vi "myRIO_BRig_RT_v0,79__PortC.vi"() -> ()   [LabVIEW 2014]
uses:
  myRIO_BRig_RT__Case_Exp_stateList.ctl
  myRIO_BRig_RT__Case_NonExp_stateList.ctl
  <vilib>/Platform/TimedLoop/XDataNode/timing_clust.ctl
  <vilib>/Platform/TimedLoop/XDataNode/nitl_modes.ctl
  <vilib>/Platform/TimedLoop/XDataNode/wakeup.ctl
  <vilib>/WebDAVClient/Advanced/SessionHandle.ctl
  <vilib>/myRIO/Common/Instrument Driver Framework/myRIO v1.0/UART/vis/myRIO v1.0 Close UART.vi
  <vilib>/FPGAPlugInAG/myRIO-1900/niLvFpga_Open_myRIO-1900.vi
  <vilib>/rvi/interface/common/dynamic/niFpgaDynamicAddResources.vi
  <vilib>/Utility/error.llb/Error Cluster From Error Code.vi
  <vilib>/rvi/errors/niLvFpgaAdjustHostInterfaceError.vi
  <vilib>/FPGAPlugInAG/Dynamic/niLvFpga_Close_Dynamic.vi
  <vilib>/myRIO/Common/Instrument Driver Framework/Utilities/vis/FPGA Ref Manager.vi
  <vilib>/myRIO/Common/Instrument Driver Framework/myRIO v1.0/myRIO v1.0 Reset FPGA.vi
  <vilib>/myRIO/Common/Instrument Driver Framework/myRIO v1.0/IRQ/vis/myRIO v1.0 IRQ Info FGV.vi
  <vilib>/myRIO/Common/Instrument Driver Framework/myRIO v1.0/IRQ/vis/myRIO v1.0 Timer IRQ Info FGV.vi
  <vilib>/myRIO/Common/Instrument Driver Framework/myRIO v1.0/IRQ/vis/myRIO v1.0 ISR Agent.vi
  <vilib>/rvi/interface/nirviOpenFPGA/nirviOpenFPGA.xnode
  FPGA Bitfiles/myRIOBRig_FPGATarget_myRIOBRigFPGAv3,_Jim92IOu6W4.lvbitx
  myRIO_BRig_FPGA_v3,70__PortC.vi
  <vilib>/rvi/interface/nirviReadWriteControl/nirviReadWriteControl.xnode
  <vilib>/Platform/TimedLoop/XDataNode/XDataNode.xnode
  <vilib>/rvi/interface/nirviCloseFPGA/nirviCloseFPGA.xnode
  <vilib>/Platform/TimedLoop/XDataNode/XDNodeRunTimeDep.lvlib
  <vilib>/rvi/interface/Simulation/niFpgaSimulationCallBeginRW.vi
  <vilib>/myRIO/Instrument Drivers/Utilities/Utilities.lvlib
  <vilib>/WebDAVClient/NI_WebDAV.lvlib
  NiFpgaLv.dll
panel:
  out "power_l2":dbl
  out "error out 6":errorcluster
  in  "MTrig_Laser_Switch":bool
  in  "Cue1Param_AudioLed_Count_NS":u16
  in  "Cue1Param_AudioLed_Count_Switch":u16
  in  "Cue1Param_AudioLed_Probability_NS":u16
  in  "Cue1Param_CueType_NS":u16(slide) max=2 step=1 scale=0.0..2.0
  in  "Cue1Param_AudioLed_Probability_Switch":u16
  in  "Cue1Param_CueType_Switch":u16(slide) max=2 step=1 scale=0.0..2.0
  in  "CueLed_Freq":dbl=10.0
  in  "CueLed_Tpeak":dbl=2.0
  in  "CueLed_duration":u16
  in  "Laser_power_step_l2":dbl
  in  "Laser_power_max_l2":dbl
  in  "Laser_power_min_l2":dbl
  in  "Laser_Tshutter_l2":dbl=2.0
  in  "Laser_Freq_l2":dbl=10.0
  in  "Laser_Tpeak_l2":dbl=2.0
  in  "Laser_duration_l2":u16
  in  "LC_Sel_Count_NS_l2":u16
  in  "LC_Sel_Count_Switch_l2":u16
  in  "LC_Sel_Probability_NS_l2":u16
  in  "LC_Sel_Block_NS_l2":u16(slide) max=2 step=1 scale=0.0..2.0
  in  "LC_Sel_OnOff_NS_l2":bool
  in  "LC_Sel_Probability_Switch_l2":u16
  in  "LC_Sel_Block_Switch_l2":u16(slide) max=2 step=1 scale=0.0..2.0
  in  "LC_Sel_OnOff_Switch_l2":bool
  in  "LC_Sel_Tdelay_NS_l2":u16
  in  "LC_Sel_Tdelay_Switch_l2":u16
  in  "LC_Cue1_Count_NS_l2":u16
  in  "LC_Cue1_Count_Switch_l2":u16
  in  "LC_Cue1_delayOpt_NS_l2":bool
  in  "LC_ENL1_delayOpt_NS_l2":bool
  in  "LC_ENL1_Count_NS_l2":u16
  in  "LC_ENL1_Count_Switch_l2":u16
  in  "LC_Cue1_delayOpt_Switch_l2":bool
  in  "LC_ENL1_delayOpt_Switch_l2":bool
  in  "LC_Cue1_Probability_NS_l2":u16
  in  "LC_Cue1_Block_NS_l2":u16(slide) max=2 step=1 scale=0.0..2.0
  in  "LC_Cue1_OnOff_NS_l2":bool
  in  "LC_Cue1_Probability_Switch_l2":u16
  in  "LC_Cue1_Block_Switch_l2":u16(slide) max=2 step=1 scale=0.0..2.0
  in  "LC_Cue1_OnOff_Switch_l2":bool
  in  "LC_ENL1_Probability_NS_l2":u16 max=100 step=1
  in  "LC_ENL1_Block_NS_l2":u16(slide) max=2 step=1 scale=0.0..2.0
  in  "LC_ENL1_OnOff_NS_l2":bool
  in  "LC_ENL1_Probability_Switch_l2":u16 max=100 step=1
  in  "LC_ENL1_Block_Switch_l2":u16(slide) max=2 step=1 scale=0.0..2.0
  in  "LC_Cue1_Tdelay_NS_l2":u16
  in  "LC_ENL1_Tdelay_NS_l2":u16
  in  "LC_Cue1_Tdelay_Switch_l2":u16
  in  "LC_ENL1_Tdelay_Switch_l2":u16
  in  "LC_ENL1_OnOff_Switch_l2":bool
  in  "LC_Wrong_Probability_l2":u16
  in  "LC_Wrong_Trial_l2":u16(slide) max=2 step=1 scale=0.0..2.0
  in  "LC_Wrong_Block_l2":u16(slide) max=2 step=1 scale=0.0..2.0
  in  "LC_Wrong_OnOff_l2":bool
  in  "LC_Reward_Probability_l2":u16
  in  "LC_Reward_Trial_l2":u16(slide) max=2 step=1 scale=0.0..2.0
  in  "LC_Reward_Block_l2":u16(slide) max=2 step=1 scale=0.0..2.0
  in  "LC_Reward_OnOff_l2":bool
  in  "LC_Wrong_Tdelay_l2":u16
  in  "LC_Reward_Tdelay_l2":u16
  in  "LC_Sel_Count_NS_l1":u16
  in  "LC_Sel_Count_Switch_l1":u16
  in  "LC_Sel_Probability_NS_l1":u16
  in  "LC_Sel_Block_NS_l1":u16(slide) max=2 step=1 scale=0.0..2.0
  in  "LC_Sel_OnOff_NS_l1":bool
  in  "LC_Sel_Probability_Switch_l1":u16
  in  "LC_Sel_Block_Switch_l1":u16(slide) max=2 step=1 scale=0.0..2.0
  in  "LC_Sel_OnOff_Switch_l1":bool
  in  "LC_Sel_Tdelay_NS_l1":u16
  in  "LC_Sel_Tdelay_Switch_l1":u16
  out "I_connect_TCP":bool
  out "error out 5":errorcluster
  in  "get_countPerMS":bool
  in  "count_warmup_R_reset":bool
  in  "count_warmup_L_reset":bool
  out "count_warmup_R":u16
  out "count_warmup_L":u16
  out "SolenoidReward":bool
  in  "SolenoidProbability_L":u16=50 caption="Reward Time [ms]" min=1 max=1000 step=1
  in  "SolenoidProbability_R":u16=50 caption="Reward Time [ms]" min=1 max=1000 step=1
  out "power_l1":dbl caption="LaserPower"
  out "error out 4":errorcluster
  in  "Laser_power_step_l1":dbl
  in  "Laser_power_max_l1":dbl
  in  "Recording":bool
  out "error out 3":errorcluster
  out "error out 2":errorcluster
  in  "Laser_power_min_l1":dbl
  in  "FPGA_count2ms":dbl=159.0
  in  "Laser_Tshutter_l1":dbl=2.0
  in  "Laser_Freq_l1":dbl=10.0
  in  "Laser_Tpeak_l1":dbl=2.0
  in  "Laser_duration_l1":u16
  out "error out":errorcluster
  in  "LC_Cue1_Count_NS_l1":u16
  in  "LC_Cue1_Count_Switch_l1":u16
  in  "LC_Cue1_delayOpt_NS_l1":bool
  in  "LC_ENL1_delayOpt_NS_l1":bool
  in  "LC_ENL1_Count_NS_l1":u16
  in  "LC_ENL1_Count_Switch_l1":u16
  in  "LC_Cue1_delayOpt_Switch_l1":bool
  in  "LC_ENL1_delayOpt_Switch_l1":bool
  in  "Tcycle_Cue_max":u16=1000 caption="Max" min=5 max=5000 step=5
  in  "Tcycle_Cue_min":u16=1000 caption="Min" min=5 max=5000 step=5
  in  "SendData":bool
  out "cSpout":enum16{"Left", "Right"}(ring) caption="Left or Right Spout"
  out "A4":u32 caption="LickCounter_Right"
  out "A2":u32 caption="LickCounter_Left"
  in  "LR_wrong_Event":bool
  out "error_initTrial":errorcluster
  out "error_Selection_pre":errorcluster
  out "error_Selection":errorcluster
  out "SelectWrong":bool
  out "SelectReward":bool
  in  "Left(F)_or_Right(T)":bool
  in  "ignoreWrong":bool
  in  "SelectionState":bool
  in  "LR_wrong_Laser":bool
  in  "LR_reward_Laser":bool
  in  "LR_reward_Event":bool
  out "nRewards_Right":u16 caption="# Rewards Total (Right)"
  out "nRewards_Left":u16 caption="# Rewards Total (Left)"
  out "nRewards_cur":u16 caption="# Rewards in Current Block"
  out "TpB_target":u16 caption="Target Trials Per Block"
  out "cState_NonExp":T1 caption="WarmUp State"
  out "iBlock":u16 caption="Current Block"
  out "cState":T2 caption="Experimental State"
  out "iTrial":u16 caption="Current Trial"
  in  "warmupType":u8(slide) max=2 step=1 scale=0.0..2.0
  in  "TestConnection":bool
  in  "warmup":bool caption="WarmUp"
  in  "Data Set Prefix":string="Exp1_TM2"
  out "Connected To Host?":bool
  in  "Host Password":string="sabalab"
  in  "Host UserName":string="Test2"
  in  "sp_RightSpout":u16(slide)=2 max=2 step=1 scale=0.0..2.0
  in  "sp_LeftSpout":u16(slide)=2 max=2 step=1 scale=0.0..2.0
  in  "BUR_max":u16 caption="Count Reward Structure  (0 = off)"
  in  "LC_Wrong_Probability_l1":u16
  in  "LC_Wrong_Trial_l1":u16(slide) max=2 step=1 scale=0.0..2.0
  in  "LC_Wrong_Block_l1":u16(slide) max=2 step=1 scale=0.0..2.0
  in  "LC_Wrong_OnOff_l1":bool
  in  "LC_Reward_Probability_l1":u16
  in  "LC_Reward_Trial_l1":u16(slide) max=2 step=1 scale=0.0..2.0
  in  "LC_Reward_Block_l1":u16(slide) max=2 step=1 scale=0.0..2.0
  in  "LC_Reward_OnOff_l1":bool
  in  "LC_Cue1_Probability_NS_l1":u16
  in  "LC_Cue1_Block_NS_l1":u16(slide) max=2 step=1 scale=0.0..2.0
  in  "LC_Cue1_OnOff_NS_l1":bool
  in  "LC_Cue1_Probability_Switch_l1":u16
  in  "LC_Cue1_Block_Switch_l1":u16(slide) max=2 step=1 scale=0.0..2.0
  in  "LC_Cue1_OnOff_Switch_l1":bool
  in  "LC_ENL1_Probability_NS_l1":u16 max=100 step=1
  in  "LC_ENL1_Block_NS_l1":u16(slide) max=2 step=1 scale=0.0..2.0
  in  "LC_ENL1_OnOff_NS_l1":bool
  in  "LC_ENL1_Probability_Switch_l1":u16 max=100 step=1
  in  "LC_ENL1_Block_Switch_l1":u16(slide) max=2 step=1 scale=0.0..2.0
  in  "Tcycle_Timeout":u16=1000 caption="Timeout Time [ms]" min=10 max=10000 step=1
  in  "Tcycle_Wrong":u16=1000 caption="Wrong Time [ms]" min=10 max=10000 step=1
  in  "Tcycle_Selection":u16=1000 caption="Answer Time [ms]" min=1 max=10000 step=1
  in  "Tcycle_RewardPost":u16=1000 caption="Consumption Time [ms]" min=250 max=10000 step=250
  in  "Tcycle_Reward_L":u16=500 caption="Reward Time [ms]" min=1 max=1000 step=1
  in  "Tcycle_Reward_R":u16=500 caption="Reward Time [ms]" min=1 max=1000 step=1
  in  "TpB_Max_R":u16=4 caption="Max TrialsPerBlock" min=1 max=12 step=1
  in  "TpB_Min_R":u16=4 caption="Min TrialsPerBlock" min=1 max=12 step=1
  in  "TpB_Max_L":u16=4 caption="Max TrialsPerBlock" min=1 max=12 step=1
  in  "TpB_Min_L":u16=4 caption="Min TrialsPerBlock" min=1 max=12 step=1
  in  "BUR_min":u16 caption="Count Reward Structure\n(0 = off)"
  in  "TrialUntilReward":bool caption="Ignore Wrong Selection"
  in  "CueCycles":u16=1 caption="Cue Structure" min=1 max=1 step=1
  in  "MTrig_Laser_Tcycle":u16=10 caption="Time [ms]"
  in  "MTrig_Laser_trig":bool
  in  "MTrig_Audio_trig__R":bool caption="Trigger Audio"
  in  "MTrig_Audio_trig__L":bool caption="Trigger Audio"
  in  "RewCalib_Trig_R":bool caption="Calibrate_R"
  in  "RewCalib_Trig_L":bool caption="Calibrate_L"
  in  "MTrig_Solenoid_Tcycle__R":u16=300 caption="Time [ms]"
  in  "MTrig_Solenoid_Tcycle__L":u16=300 caption="Time [ms]"
  in  "MTrig_Solenoid_trig__R":bool caption="Solenoid"
  in  "MTrig_Solenoid_trig__L":bool caption="Solenoid"
  in  "STOP_abort":bool caption="Stop LabView\n(Stops myRio and FPGA)"
  in  "STOP_endBlock":bool caption="Stop Experiment\n@ End of Block"
  in  "STOP_endTrial":bool caption="Stop Experiment\n@ End of Trial"
  in  "START":bool caption="Start Experiment"
  in  "Tcycle_CuePenalty":u16=1000 caption="Penalty" min=1 max=10000 step=1
  in  "Audio_Amp__R":u16=100 caption="Amp"
  in  "Audio_Freq__R":u8=5 caption="Freq [kHz]" max=14 step=1
  in  "Audio_Amp__L":u16=100 caption="Amp"
  in  "Audio_Freq__L":u8=5 caption="Freq [kHz]" max=14 step=1
  in  "LC_Wrong_Tdelay_l1":u16
  in  "LC_Cue1_Tdelay_NS_l1":u16
  in  "LC_ENL1_Tdelay_NS_l1":u16
  in  "LC_Reward_Tdelay_l1":u16
  in  "LC_Cue1_Tdelay_Switch_l1":u16
  in  "LC_ENL1_Tdelay_Switch_l1":u16
  in  "LC_ENL1_OnOff_Switch_l1":bool
  in  "Tcycle_ENLPenalty":u16=100 caption="Penalty" min=10 max=10000 step=10
  in  "Tcycle_ENL_max":u16=1000 caption="Max" min=250 max=10000 step=250
  in  "Tcycle_ENL_min":u16=1000 caption="Min" min=250 max=10000 step=250
  # "Communication (Host PC)"
  # "Recording Rig"
  # "Experimental Run"
  # "Current State"
  # "STOP experiment at"
  # "Global Parameters                                                         Trial Parameters"
  # "Left/Right        Give Reward?        Laser Power [V]"
  # "Laser1      Laser2"
  # "FPGA Count per [ms]"
  # "Experiment Task Structure"
  # "Timing [ms]"
  # "Block                   Trial            Target Trials       # Rewards \n                                                            Per Block             Current"
  # "Min            Max            Penalty"
  # "(1) = Switching\n(2) = Two Choice"
  # "WarmUp State"
  # "Lick Counter"
  # "Enforced\nNonLick"
  # "WarmUp"
  # "Left           Right"
  # "Cue then reward (no lick)\n \nLeft                    Right"
  # "# Rewards Total\n                                                                  Left                    Right"
  # "Cue"
  # "Experimental State"
  # "Selection\n \n\n \nReward\n    Dispense\n    Time\n \n    Dispense\n    Probability\n \n\n    Consumption\n    Time\n\nWrong Choice\n \n \nTimeout Penalty"
  # "Left                  Right"
  # "Manual Control"
  # "Min"
  # "Max"
  # "Solenoid\n \nLeft              Right"
  # "Speaker\n \nLeft                    Right"
  # "Laser 1  |  Laser 2"
  # "Trial Per Block Structure \n               Left                        Right"
  # "Time\n[ms]"
  # "Time\n[ms]"
  # "Time = Cue Min"
  # "Min"
  # "Power = Min"
  # "Max"
  # "Cue1 Control\n                                  Cue Type           LED Probability [%]      Count"
  # "Laser1 Control\n                               On/Off      Block        Probability [%]   Delay [ms]                              Count"
  # "Laser2 Control\n                               On/Off      Block        Probability [%]   Delay [ms]                              Count"
  # "Audio or LED"
  # "Cue 1"
  # "Enforced\nNonLick\n      1"
  # "Enforced\nNonLick\n      1"
  # "from end"
  # "from end"
  # "Switch\nTrial"
  # "Switch\nTrial"
  # "Switch\nTrial"
  # "from start"
  # "from start"
  # "from end"
  # "from end"
  # "NonSwitch\nTrials"
  # "NonSwitch\nTrials"
  # "NonSwitch\nTrials"
  # "from start"
  # "from start"
  # "Cue 1"
  # "Cue 1"
  # "from end"
  # "from end"
  # "Switch\nTrial"
  # "Switch\nTrial"
  # "Cue Audio Parameters"
  # "Cue LED Parameters"
  # "from start"
  # "from start"
  # "Left                  Right"
  # "Frequency\n[Hz]"
  # "Frequency\n[kHz]"
  # "from end"
  # "from end"
  # "NonSwitch\nTrials"
  # "NonSwitch\nTrials"
  # "Timing [ms]\n Duration     Peak Width"
  # "from start"
  # "from start"
  # "Amp\n(0 - 32,000)"
  # "Selection"
  # "Selection"
  # "from start"
  # "from start"
  # "Switch\nTrial"
  # "Switch\nTrial"
  # "Speaker\nPattern\nDuring Cue"
  # "from start"
  # "from start"
  # "NonSwitch\nTrials"
  # "NonSwitch\nTrials"
  # "Laser1 Parameters"
  # "Laser2 Parameters"
  # "Laser1 Response\n                               On/Off      Block       Trial       Probability [%]   Delay [ms]"
  # "Laser2 Response\n                               On/Off      Block       Trial       Probability [%]   Delay [ms]"
  # "Frequency\n[Hz]"
  # "Frequency\n[Hz]"
  # "Timing [ms]\n Duration     Peak Width   Shutter"
  # "Timing [ms]\n Duration     Peak Width   Shutter"
  # "Selection Reward"
  # "Selection Reward"
  # "Laser Power [V]\nMin          Max              Step"
  # "Laser Power [V]\nMin          Max              Step"
  # "Selection Wrong"
  # "Selection Wrong"
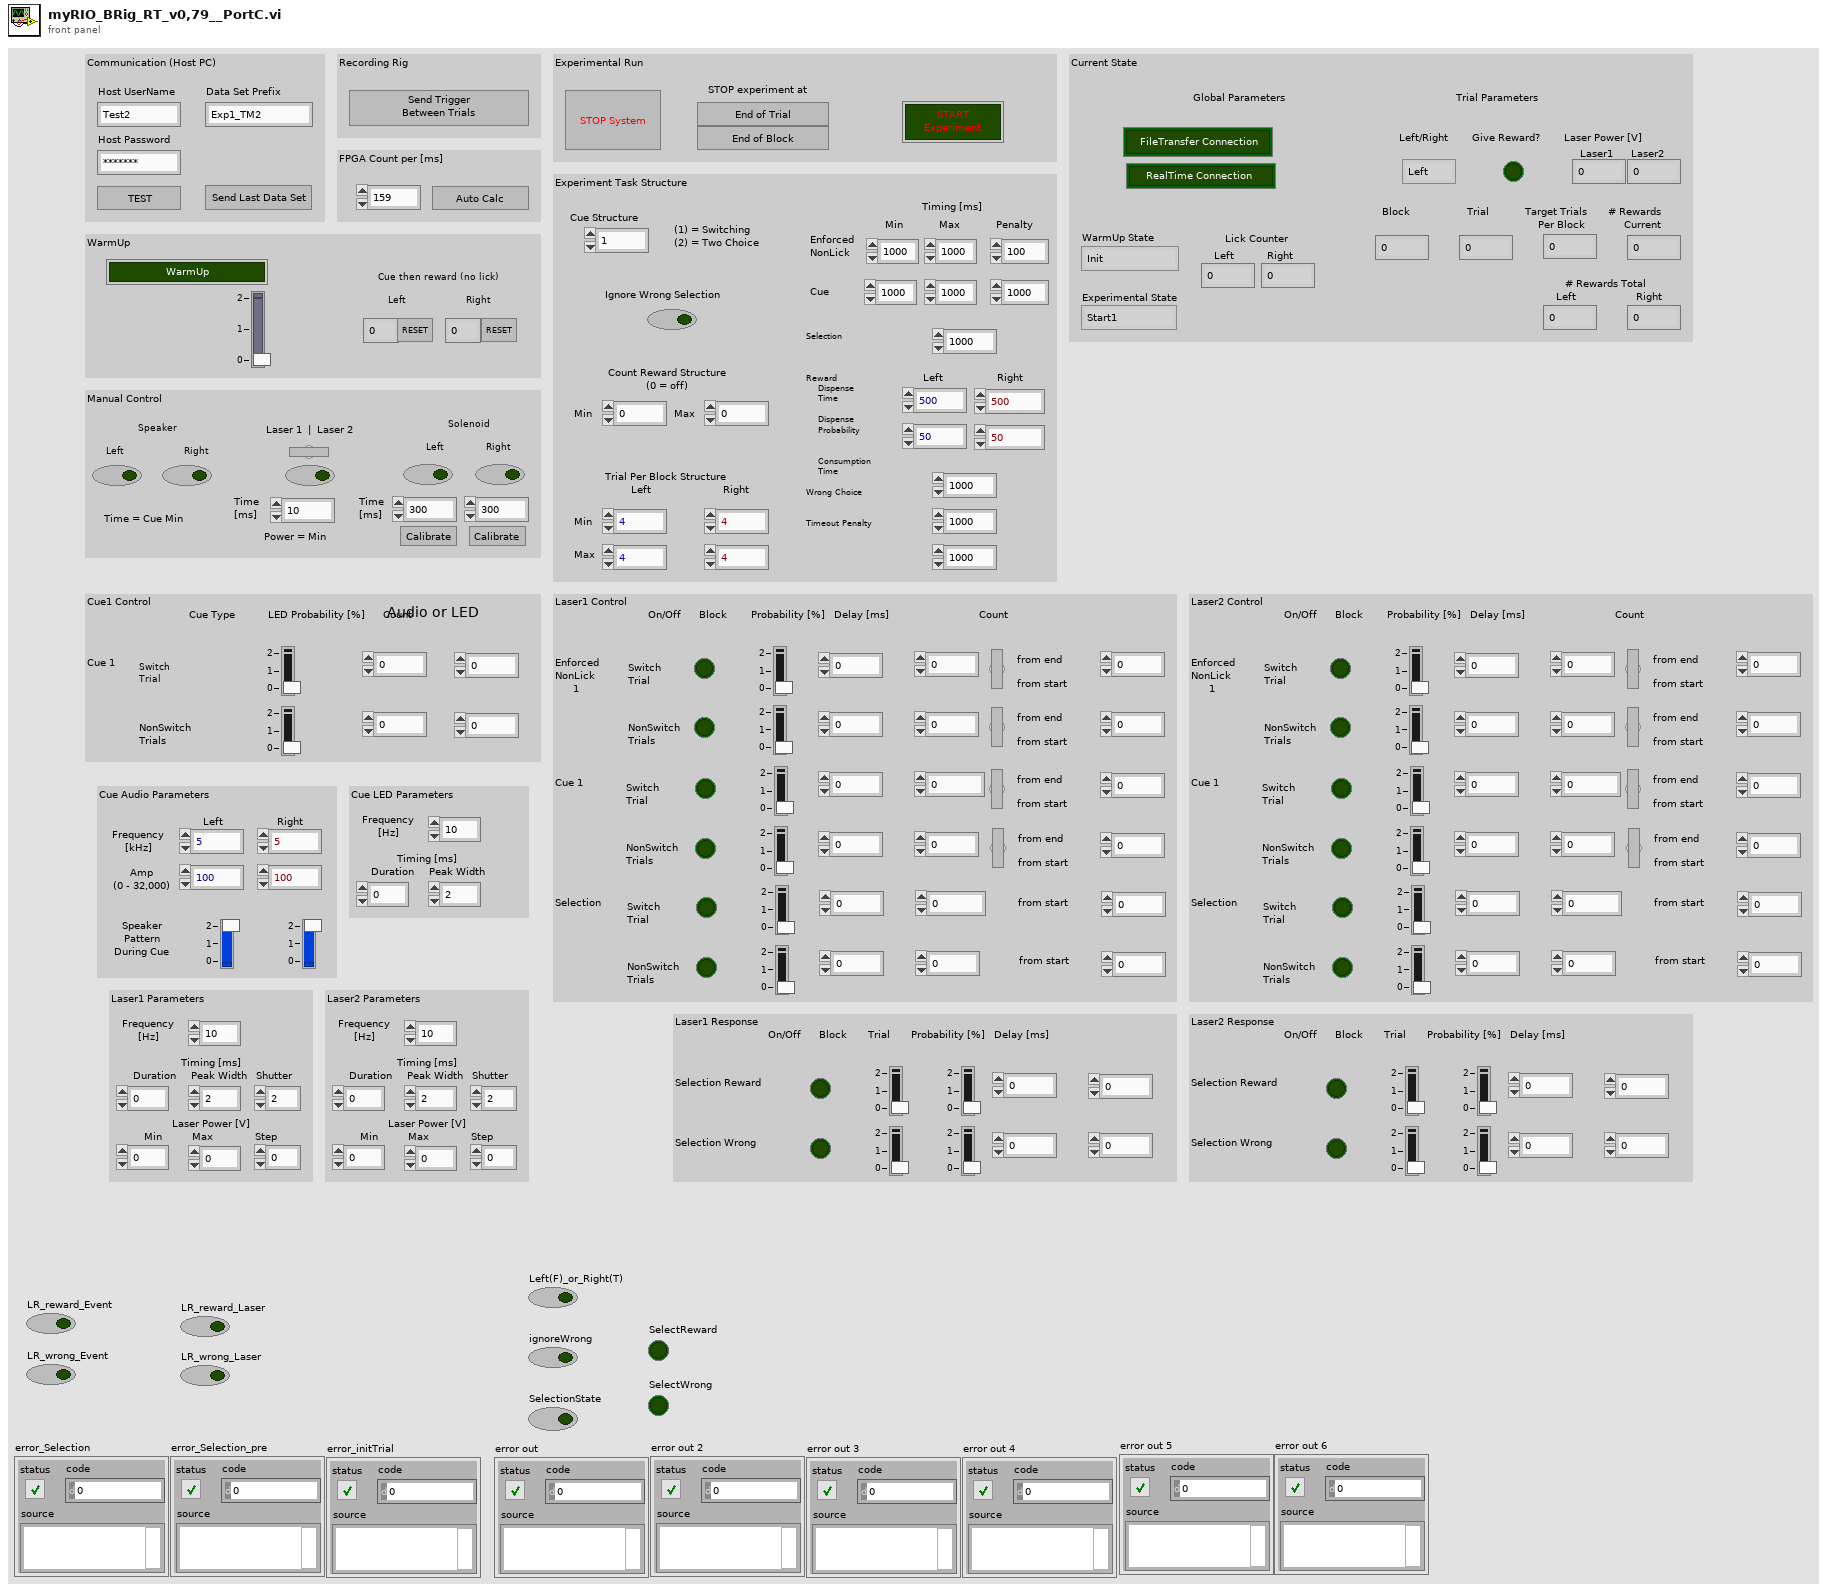
[diagram p1: front panel]
types:
  T1 = typedef "myRIO_BRig_RT__Case_NonExp_stateList.ctl" = enum16{"Init", "UploadSettings_pre", "UploadSettings_Read_dataExp", "UploadSettings_dataExp_1", "UploadSettings_dataExp_2", "UploadSettings_Read_dataLC", "UploadSettings_dataLC_1", "UploadSettings_dataLC_2", "UploadSettings_dataLC_3", "UploadSettings_dataLC_4", "UploadSettings_Read_dataMTrig", "UploadSettings_dataMTrig_1", "UploadSettings_post", "Idle_pre", "IdleEmpty", "IdleEmpty2", "IdleEmpty3", "IdleEmpty4", "Idle", "Idle_2", "Idle_3", "Idle_4", "Idle_5", "Idle_6", "Idle_post", "Cue_pre__pre", "Cue_pre", "Cue", "Cue_LED", "Cue_post", "RewardCalibration_pre", "DispenseWater_pre__pre", "DispenseWater_pre", "DispenseWater", "DispenseWater_post", "TestConnection", "SendData", "Get_FPGA_count_per_ms", "End"}
  T2 = typedef "myRIO_BRig_RT__Case_Exp_stateList.ctl" = enum16{"Start1", "Start2", "Start3", "saveSettings1", "saveSettings2", "saveSettings3", "saveSettings4", "saveSettings_LC_ENL_l1", "saveSettings_LC_ENL_l2", "saveSettings_LC_Cue_l1", "saveSettings_LC_Cue_l2", "saveSettings6_LC_l1_Other", "SaveSettings6_LC_l2_Other", "setSettings_Audio", "setSettings_Laser", "initBlock_pre", "initBlock", "initBlock2", "initBlock_post", "initTrial_pre", "initTrial", "initTrial2", "initTrial3", "initTrial4", "initTrial_LC_ENL1", "initTrial_LC_Cue1", "initTrial_LC_Cue1_2", "initTrial_LC_Sel", "initTrial_post", "ENL1_pre", "ENL1", "ENL1_post", "ENL1Penalty_pre", "ENL1Penalty", "ENL2_pre", "ENL2", "ENL2Penalty_pre", "ENL2Penalty", "Cue1_pre", "Cue1", "Cue1_post", "Cue1Penalty_pre", "Cue1Penalty", "Cue2_pre", "Cue2", "Cue2Penalty_pre", "Cue2Penalty", "Selection_pre", "Selection", "Select_post", "SelectReward_pre", "SelectReward", "SelectRewardPost_pre", "SelectRewardPost", "SelectWrong_pre", "SelectWrong", "SelectWrong_post", "SelectTimeout_pre", "SelectTimeout", "SelectTimeout_post", "endTrial_pre", "endTrial1", "endTrial2", "endTrial3", "endTrial_post", "endBlock_pre", "endBlock", "endBlock_post", "endExp", "commConnect", "commUpload_pre", "commUpload_dataBlock", "commUpload_dataCurrent", "commUpload_dataExp", "commUpload_dataLC", "commUpload_dataTrial", "commUpload_post", "saveData_pre", "saveData_dataBlock", "saveData_dataCurrent", "saveData_dataExp", "saveData_dataLC", "saveData_dataTrial", "saveData_post", "empty_endBlock1", "empty_endBlock2", "empty_endTrial1", "empty_endTrial2", "empty_endTrial3", "empty_endTrial4", "empty_endTrial5", "dummyState", "dummyState_endBlock"}
  T3 = typedef "XDNodeRunTimeDep.lvlib/timing_clust.ctl" = cluster{"Expected End [f-1]":u64, "Actual End [f-1]":u64, "Finished Late? [f-1]":bool, "Expected End [i-1]":u64, "Actual End [i-1]":u64, "Finished Late? [i-1]":bool, "Expected Start [i]":u64, "Actual Start [i]":u64, "Expected Start [f]":u64, "Actual Start [f]":u64, "Source Name":string, "Structure Name":string, "Period":i64, "Deadline":i64, "Offset":i64, "Start":i64, "Priority":i32, "Timeout":i32, "Mode":T4, "Wakeup Reason":T5, "Error":errorcluster, "Source Type":string, "Secondary Source Type":string, "Global End Time":u64, "Global Start Time":u64, "Frame Duration":u64, "Iteration Duration":u64, "Assigned CPU":i32, "I/O Scan Engine Mode":u32}
  T4 = typedef "XDNodeRunTimeDep.lvlib/nitl_modes.ctl" = enum32{"No Change", "Process missed periods, maintain original phase", "Discard missed periods, maintain original phase", "Process missed periods, ignore original phase", "Discard missed periods, ignore original phase"}
  T5 = typedef "XDNodeRunTimeDep.lvlib/wakeup.ctl" = enum32{"Normal", "Aborted", "Asynchronous wakeup", "Timing source error", "Timed loop error", "Timeout"}
  T6 = typedef "NI_WebDAV.lvlib/SessionHandle.ctl" = refnum<k1>
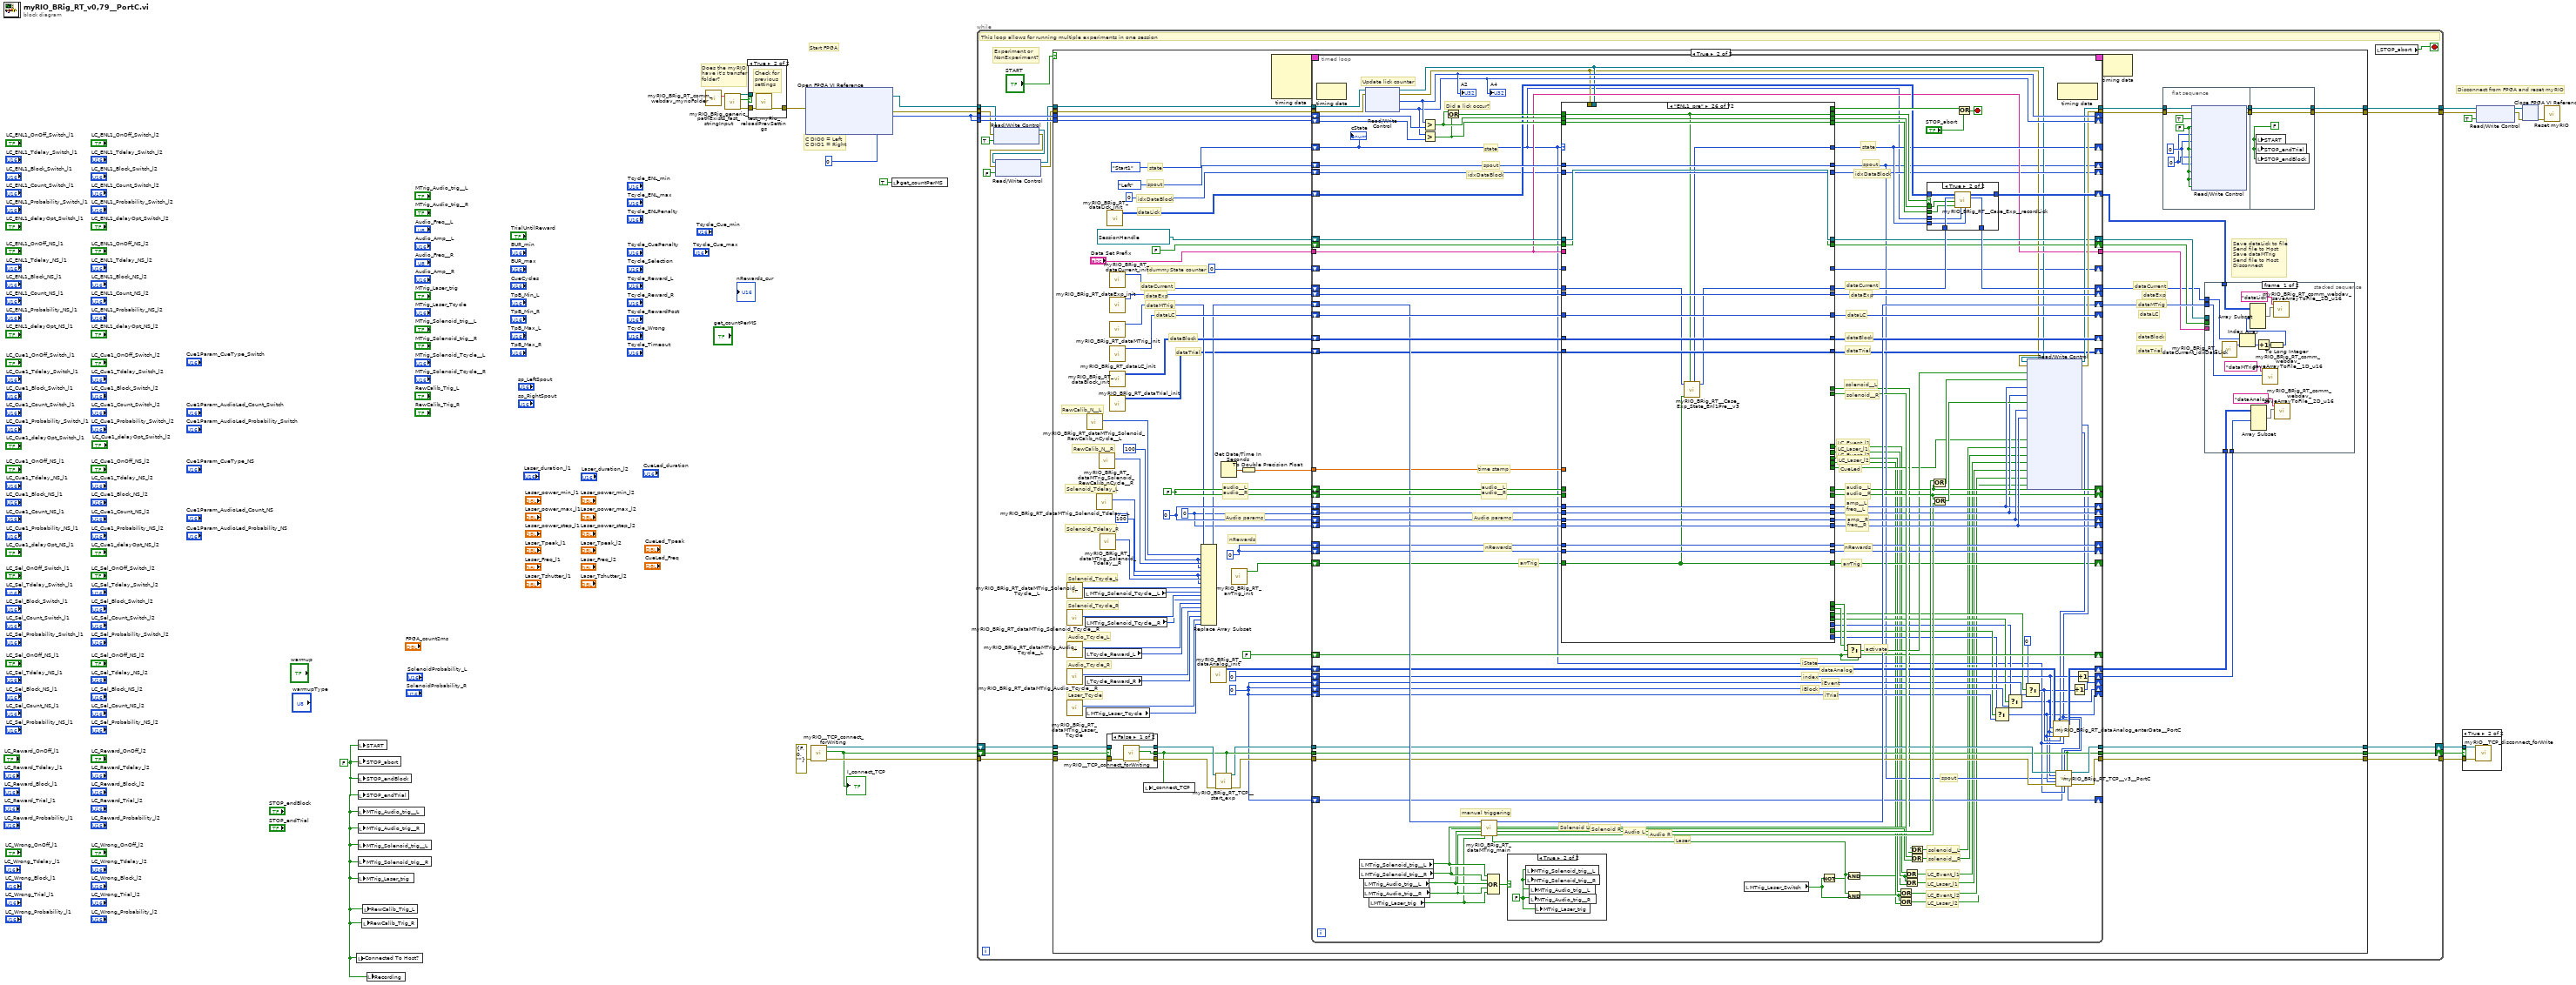
[diagram p0: block diagram]
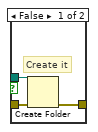
[diagram p3: hidden frame]
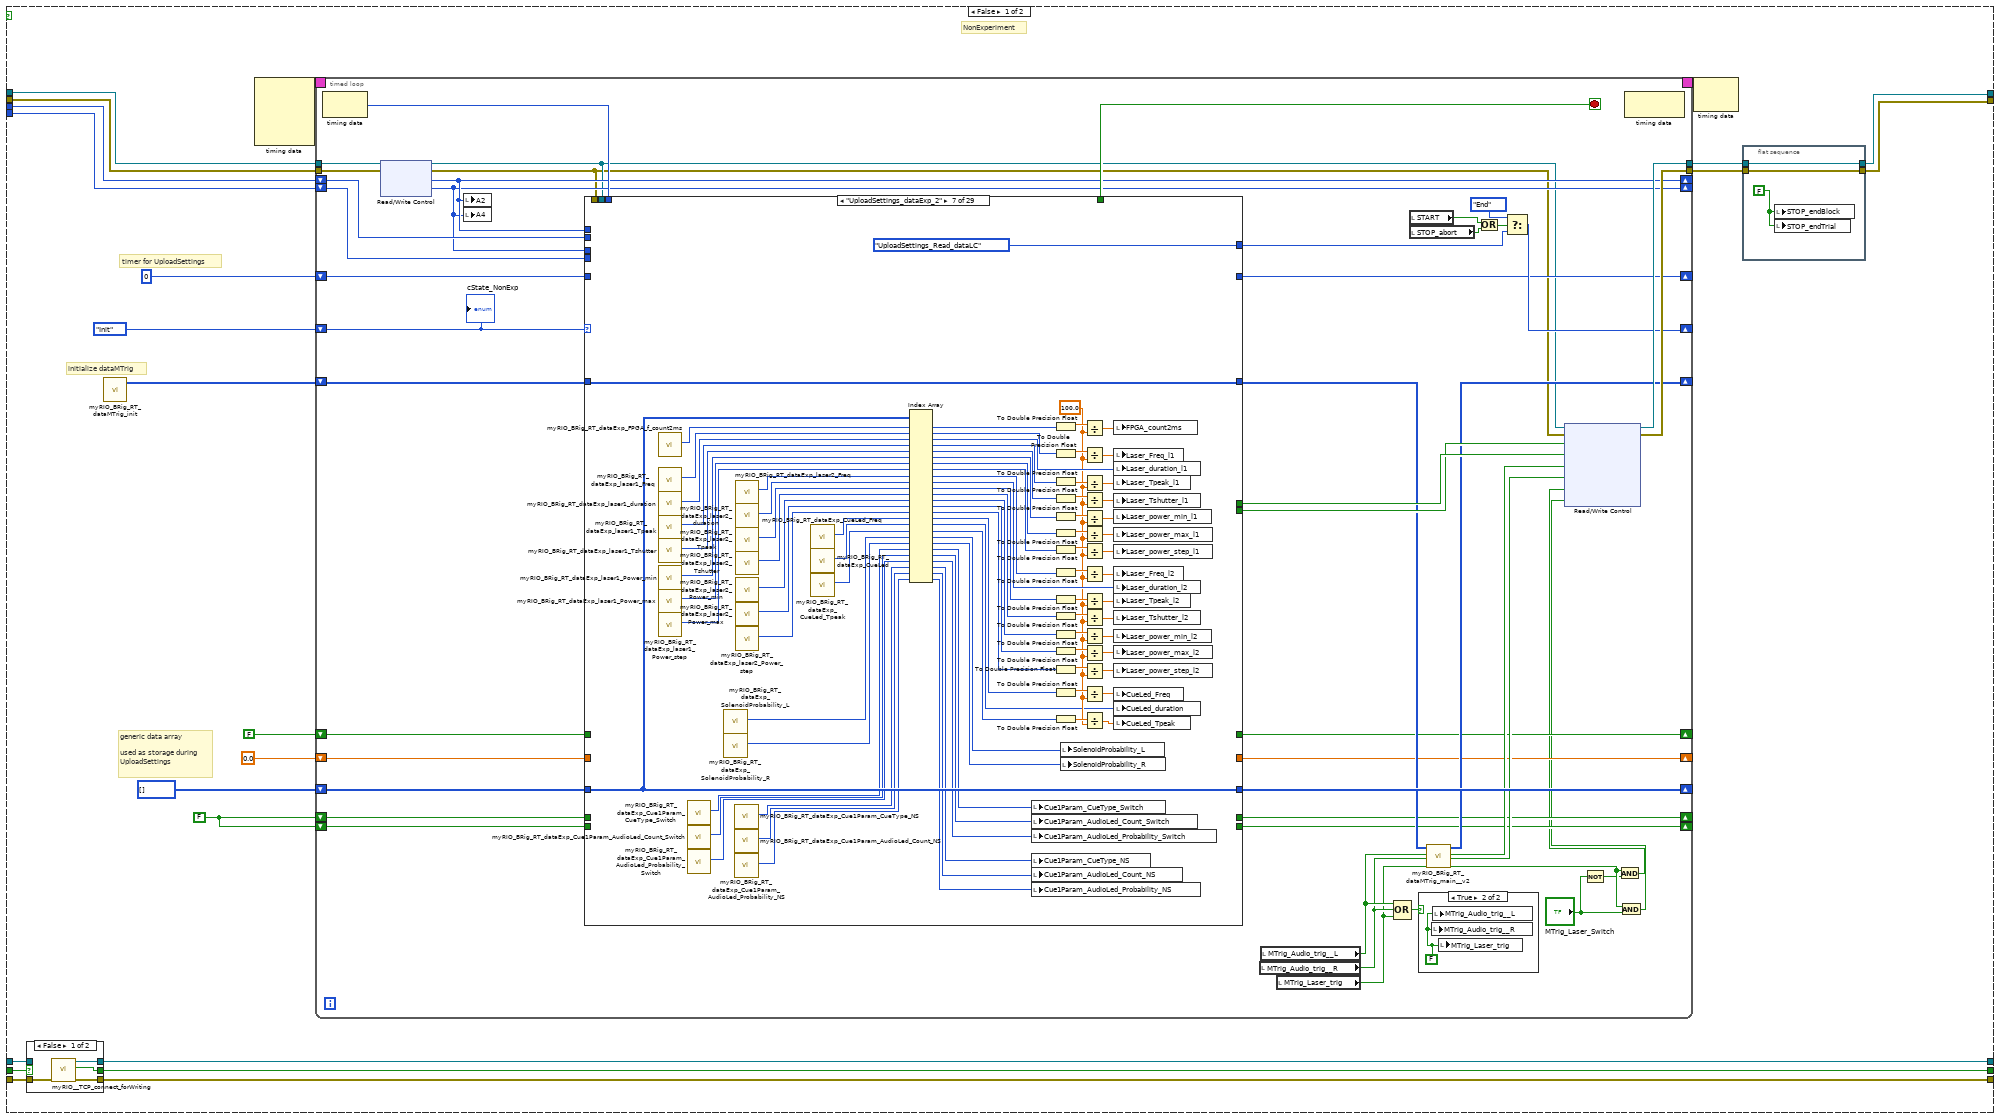
[diagram p4: hidden frame]
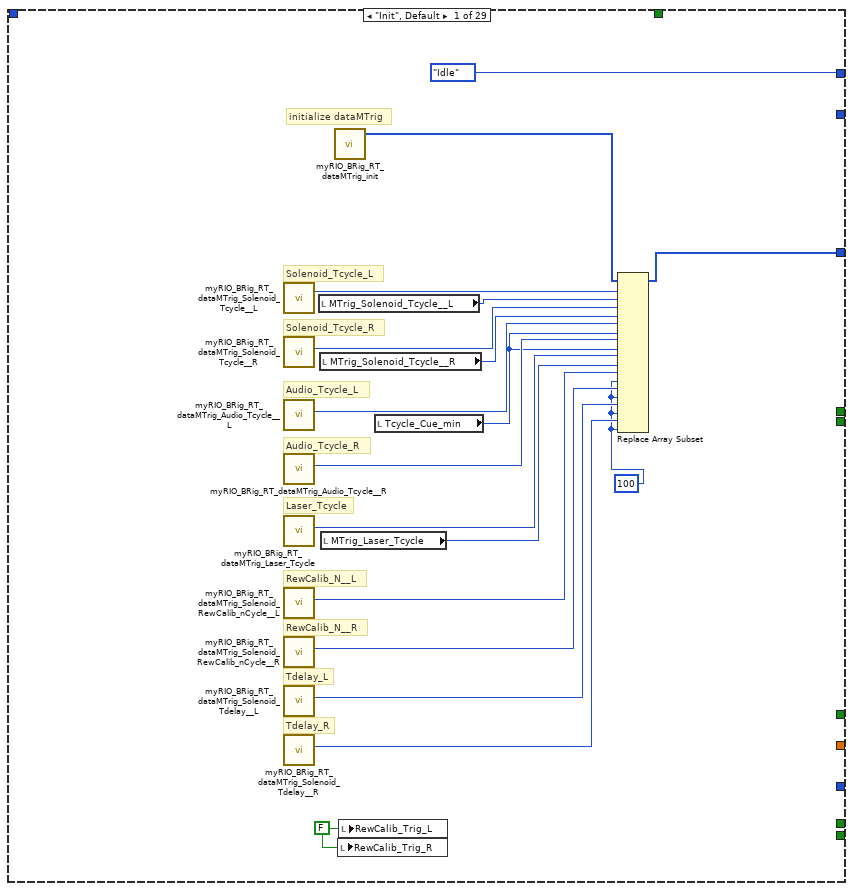
[diagram p7: hidden frame]
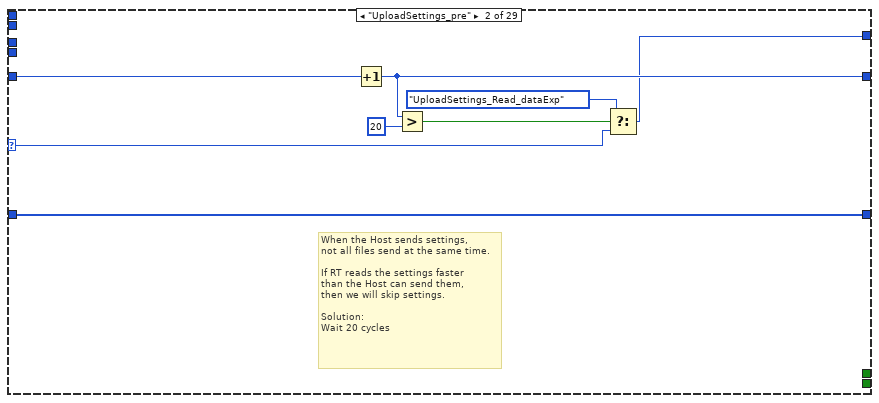
[diagram p8: hidden frame]
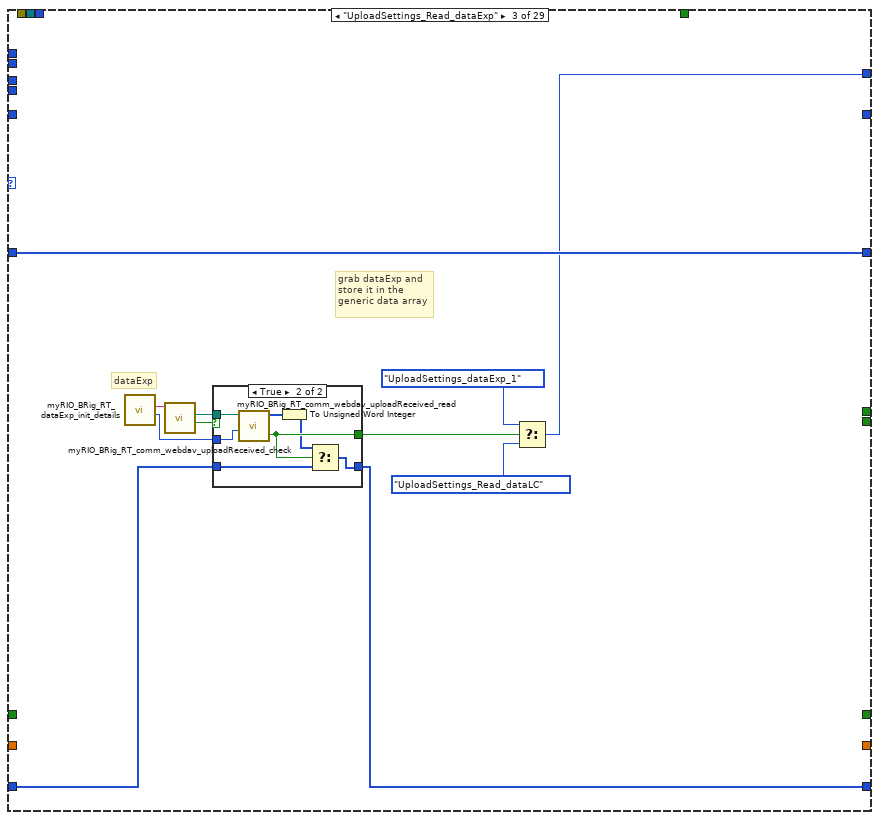
[diagram p9: hidden frame]
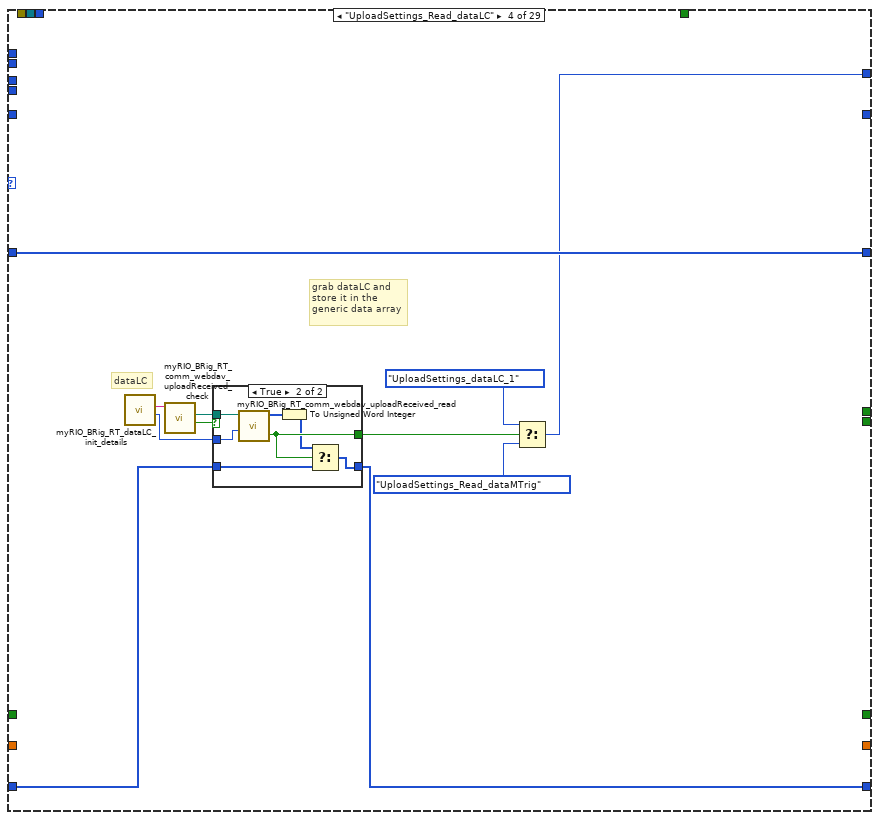
[diagram p11: hidden frame]
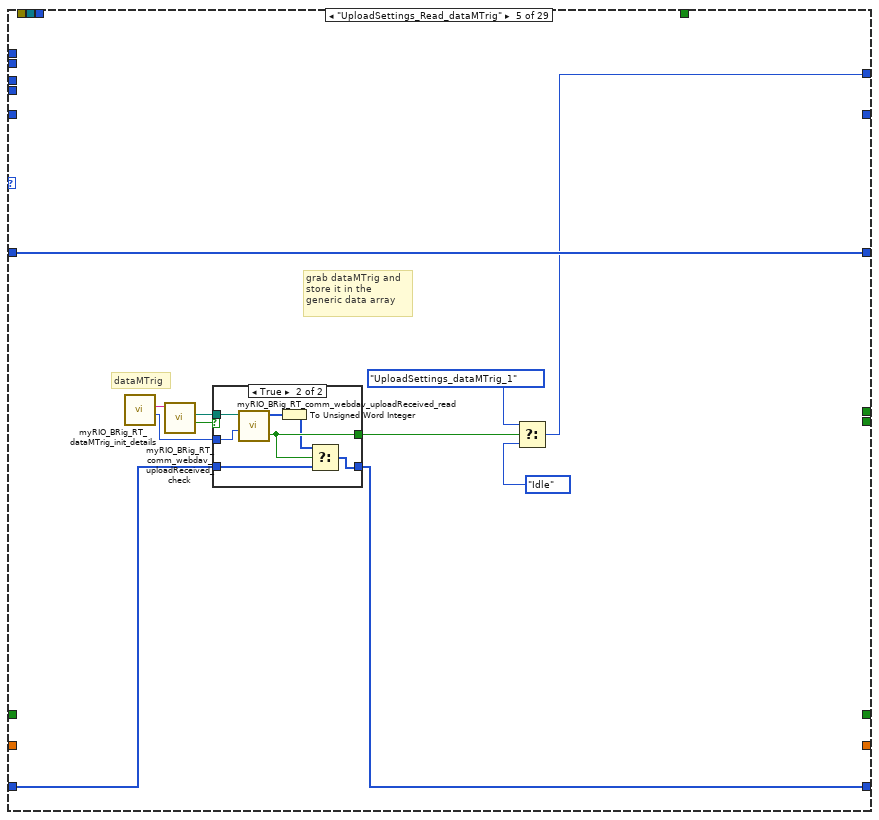
[diagram p13: hidden frame]
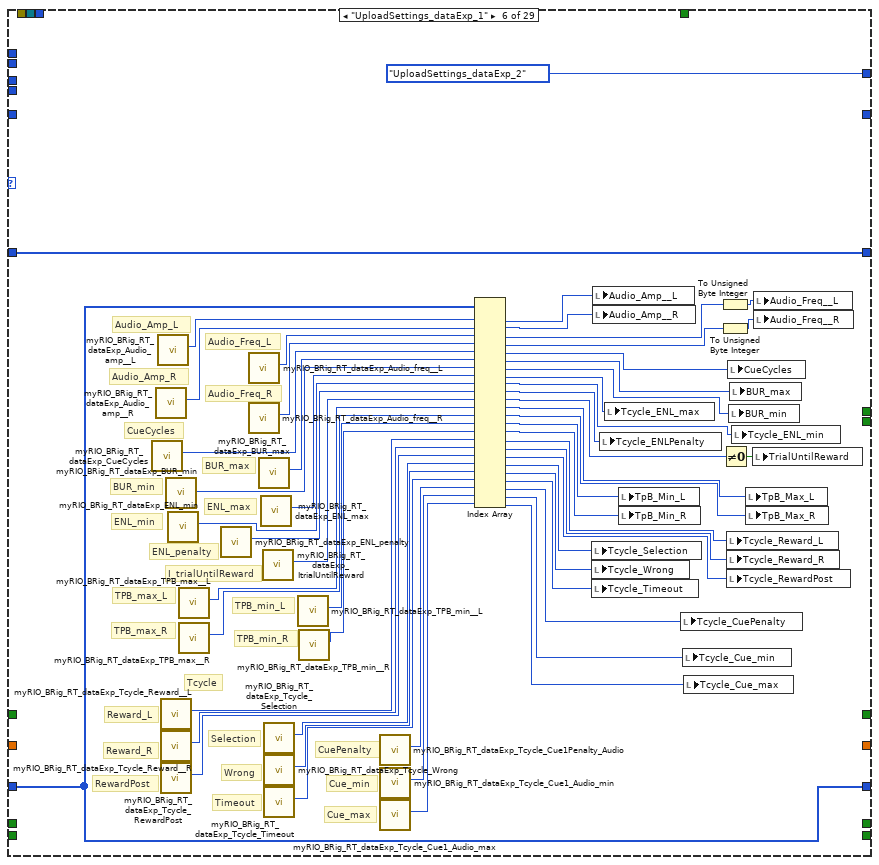
[diagram p15: hidden frame]
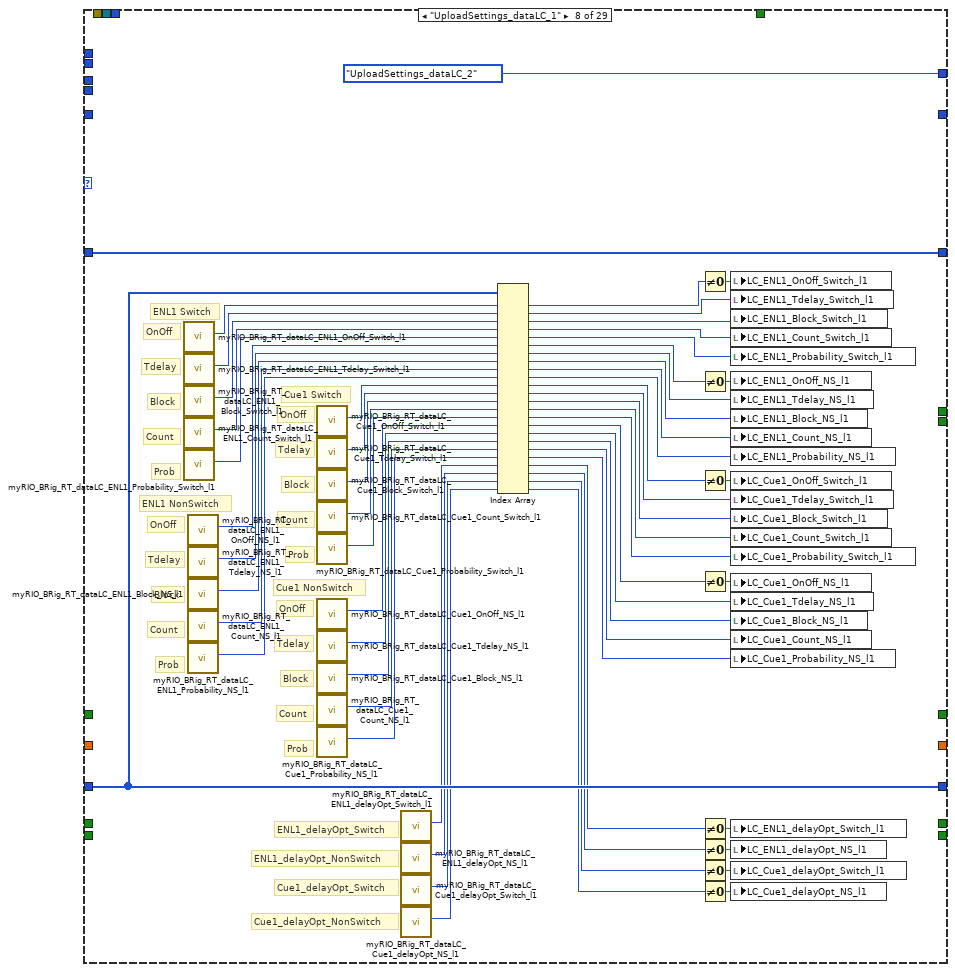
[diagram p16: hidden frame]
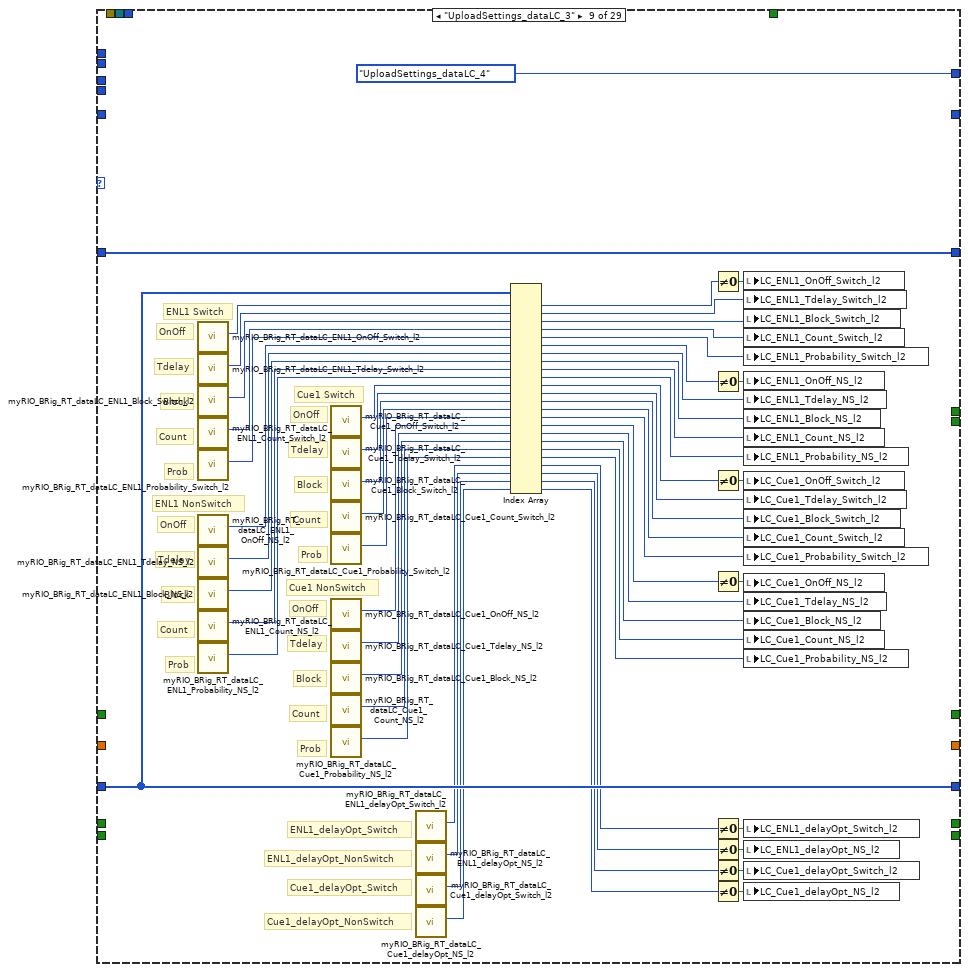
[diagram p17: hidden frame]
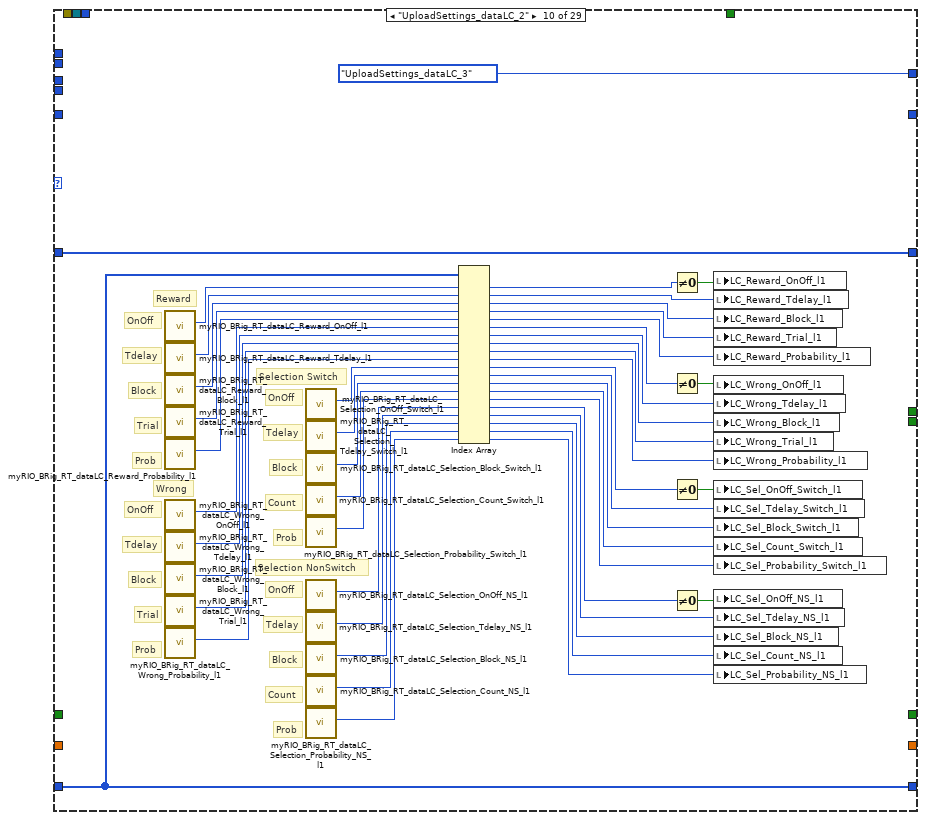
[diagram p18: hidden frame]
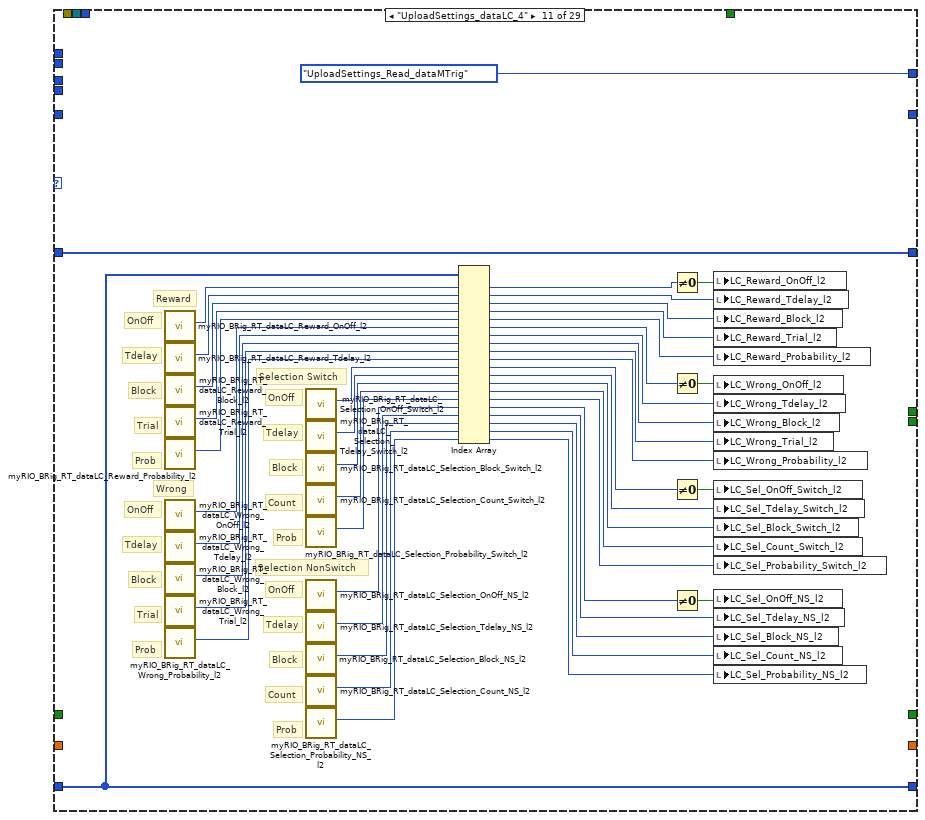
[diagram p19: hidden frame]
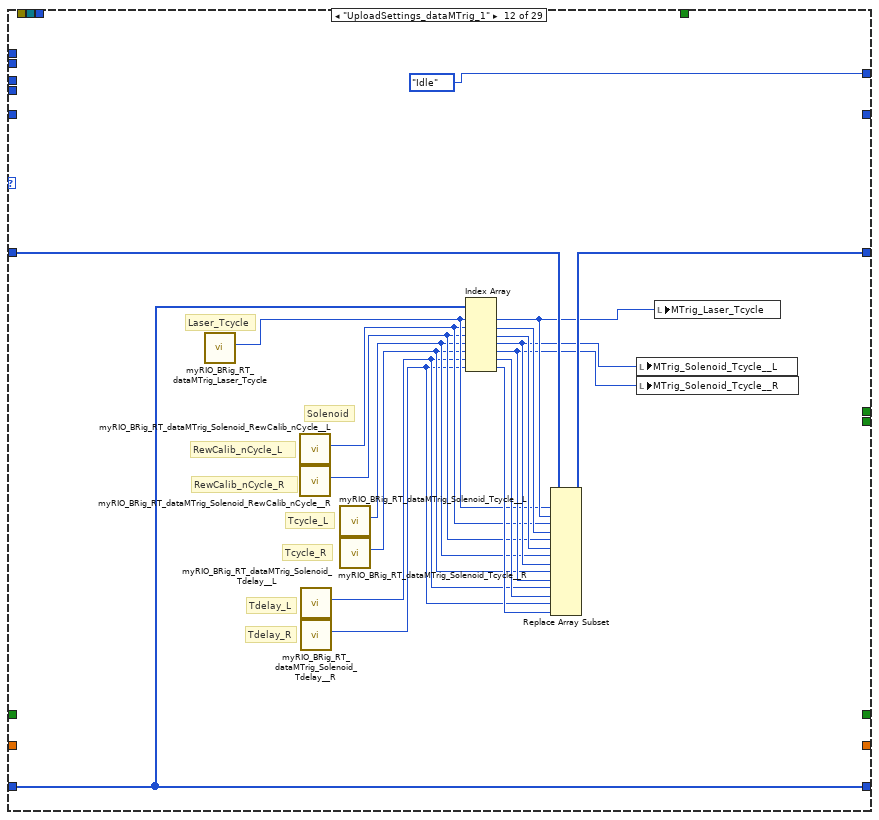
[diagram p20: hidden frame]
diagram:
  w17 = u32 0
  w1 = FALSE
  # "Does the myRIO\nhave it's transfer\nfolder?"
  # "C DIO0 = Left\nC DIO1 = Right"
  # "Start FPGA"
  # "Disconnect from FPGA and reset myRIO"
  n1 = local write "Connected To Host?"(w1) -> ()
  n2 = local write "START"(w1) -> ()
  n3 = local write "STOP_abort"(w1) -> ()
  n4 = local write "STOP_endBlock"(w1) -> ()
  n5 = local write "STOP_endTrial"(w1) -> ()
  n6 = local write "MTrig_Audio_trig__L"(w1) -> ()
  n7 = local write "MTrig_Audio_trig__R"(w1) -> ()
  n8 = local write "MTrig_Solenoid_trig__L"(w1) -> ()
  n9 = local write "MTrig_Solenoid_trig__R"(w1) -> ()
  n10 = local write "MTrig_Laser_trig"(w1) -> ()
  n11 = local write "RewCalib_Trig_R"(w1) -> ()
  n12 = local write "RewCalib_Trig_L"(w1) -> ()
  n13 = local write "Recording"(w1) -> ()
  n14 = call "myRIO_BRig_RT_comm_webdav_myrioFolder.vi"() -> ("output_myrioFolder"=w14:string)  [unwired: 11 in]
  n15 = call "myRIO_BRig_generic_pathExists_fast_stringInput.vi"("input_filePath"=w14) -> ("output_error"=w13:errorcluster, "output_Iexist"=w12:bool, "output_filePath"=w11:path)  [unwired: 8 in]
  n16 = case shown="True" w12 {
    tunnel: w11 -> [w26 _]
    tunnel: w13 -> [w25 w28]
    tunnel: [w24 w27] -> w9
    frame False {
      # "Create it"
      n17 = Create Folder(path (use dialog)=w26, error in=w25) -> (error out=w24:errorcluster)  [unwired: 1 in, 2 out]
    }
    frame True {
      # "Check for\nprevious\nsettings"
      n18 = call "test_myRio_reloadPrevSettings.vi"("input_error"=w28) -> ("output_error"=w27:errorcluster)  [unwired: 10 in]
    }
  }
  n19 = xnode "Open FPGA VI Reference"("error in"=w9) -> ("FPGA VI Reference Out"=w19:refnum<k20>, "error out"=w18:errorcluster)  [unwired: 1 in]
  n20 = call "myRIO__TCP_connect_forWriting.vi"("input_error"=errorcluster {"status"=FALSE, "code"=0, "source"=""}) -> ("output_error"=w7:errorcluster, "output_connected"=w6:bool, "output_hTCP"=w10:refnum<k5>)  [unwired: 8 in]
  "I_connect_TCP" <- w6
  n21 = local write "get_countPerMS"(TRUE ("get_countPerMS")) -> ()
  n22 = while {
    tunnel: w19 -> [w38]
    tunnel: w18 -> [w43]
    tunnel: w17 -> [w46]
    tunnel: w17 -> [w45]
    tunnel: [w36] -> w16
    tunnel: [w35] -> w15
    shift-right: [w32] -> w5
    shift-left: w6 -> [w33]
    tunnel: w7 -> [w31]
    shift-right: [w30] -> w4
    shift-left: w10 -> [w34]
    tunnel: [w29] -> w3
    stop <- w44 stop-if-true
    # "Experiment or\nNonExperiment?"
    # "This loop allows for running multiple experiments in one session"
    n23 = xnode "Read/Write Control"("FPGA VI Reference In"=w38, "error in"=w43, "Counts_Reset"=TRUE) -> ("FPGA VI Reference Out"=w40:refnum<k20>, "error out"=w41:errorcluster)
    n24 = xnode "Read/Write Control"("FPGA VI Reference In"=w40, "error in"=w41, "Counts_Reset"=FALSE) -> ("FPGA VI Reference Out"=w37:refnum<k20>, "error out"=w39:errorcluster)
    n25 = case shown="True" "START" {
      tunnel: w46 -> [w67 w1290]
      tunnel: w45 -> [w66 w1289]
      tunnel: w39 -> [w64 w1221]
      tunnel: w37 -> [w65 w1222]
      tunnel: [w62 w1286] -> w36
      tunnel: [w60 w1281] -> w35
      tunnel: w34 -> [w53 w1232]
      tunnel: [w51 w1236] -> w30
      tunnel: w33 -> [w52 w1234]
      tunnel: [w50 w1235] -> w32
      tunnel: w31 -> [w54 w1233]
      tunnel: [w49 w1231] -> w29
      frame False {
        w57 = FALSE
        # "generic data array\n\nused as storage during\nUploadSettings"
        # "timer for UploadSettings"
        # "initialize dataMTrig"
        # "NonExperiment"
        n26 = case shown="False" w52 {
          selector: w52 -> [_ w76]
          tunnel: w54 -> [w73 w78]
          tunnel: [w74 w78] -> w49
          tunnel: w53 -> [_ w77]
          tunnel: [w75 w77] -> w51
          tunnel: [w72 w76] -> w50
          frame False {
            n27 = call "myRIO__TCP_connect_forWriting.vi"("input_error"=w73) -> ("output_error"=w74:errorcluster, "output_connected"=w72:bool, "output_hTCP"=w75:refnum<k5>)  [unwired: 8 in]
          }
          frame True {
          }
        }
        n28 = call "myRIO_BRig_RT_dataMTrig_init.vi"() -> ("output_dataMTrig"=w68:u16[])  [unwired: 5 in]
        n29 = node-c288() -> (w71:T3)  [unwired: 4 in]
        n30 = timed-loop {
          timing: w71 -> [_]
          timing-out: [_] -> w70
          shift-right: [w115] -> _
          shift-left: w68 -> [w127]
          shift-right: [w109] -> _
          shift-left: myRIO_BRig_RT__Case_NonExp_stateList."Init" ("Enum") -> [w121]
          shift-right: [w103] -> _
          shift-left: w67 -> [w104]
          shift-right: [w101] -> _
          shift-left: w66 -> [w102]
          tunnel: [w123] -> w63
          tunnel: [w122] -> w61
          tunnel: w64 -> [w125]
          tunnel: w65 -> [w124]
          shift-right: [w120] -> _
          shift-left: u16[] [] ("output_data") -> [w119]
          shift-right: [w105] -> _
          shift-left: u16 0 ("Audio_Amp__L") -> [w106]
          shift-right: [w98] -> _
          shift-left: w57 -> [w100]
          shift-right: [w97] -> _
          shift-left: w57 -> [w99]
          shift-right: [w93] -> _
          shift-left: FALSE -> [w94]
          shift-right: [w91] -> _
          shift-left: 0.0 -> [w92]
          stop <- w128 stop-if-true
          n31 = node-c288() -> (w126:i64)  [unwired: 1 in]
          n32 = xnode "Read/Write Control"("FPGA VI Reference In"=w124, "error in"=w125) -> ("FPGA VI Reference Out"=w96:refnum<k20>, "error out"=w95:errorcluster, "A2_LickL"=w103:u32, "A4_LickR"=w101:u32)
          n33 = local write "A2"(w103) -> ()
          n34 = local write "A4"(w101) -> ()
          n35 = case shown="\"UploadSettings_dataExp_2\"" w121 {
            selector: w121 -> [_ w151 _ _ _ _ _ _ _ _ _ _ _ _ _ _ _ _ _ w840 w896 _ _ w1101 _ _ _ w1173 w1215]
            tunnel: [myRIO_BRig_RT__Case_NonExp_stateList."Idle" ("Enum") w149 w156 w175 w194 myRIO_BRig_RT__Case_NonExp_stateList."UploadSettings_dataExp_2" ("Enum") myRIO_BRig_RT__Case_NonExp_stateList."UploadSettings_Read_dataLC" ("Enum") myRIO_BRig_RT__Case_NonExp_stateList."UploadSettings_dataLC_2" ("Enum") myRIO_BRig_RT__Case_NonExp_stateList."UploadSettings_dataLC_4" ("Enum") myRIO_BRig_RT__Case_NonExp_stateList."UploadSettings_dataLC_3" ("f") myRIO_BRig_RT__Case_NonExp_stateList."UploadSettings_Read_dataMTrig" ("f") myRIO_BRig_RT__Case_NonExp_stateList."Idle" ("Enum") w600 w615 myRIO_BRig_RT__Case_NonExp_stateList."Idle_4" ("Enum") myRIO_BRig_RT__Case_NonExp_stateList."Idle_5" ("Enum") w712 w792 w802 w835 w891 myRIO_BRig_RT__Case_NonExp_stateList."DispenseWater_pre" ("Enum") w1047 w1099 w1121 myRIO_BRig_RT__Case_NonExp_stateList."Idle" ("Enum") myRIO_BRig_RT__Case_NonExp_stateList."Idle" ("Enum") w1172 w1215] -> w110
            tunnel: [w139 w148 w166 w185 w204 w266 w352 w405 w464 w517 w564 w580 w604 w630 w643 w698 w717 w790 w817 w841 w897 w958 w1084 w1106 w1132 w1166 w1171 w1183 w1213] -> w116
            tunnel: [_ _ _ _ _ _ _ _ _ _ _ _ _ _ _ _ _ _ _ _ _ _ _ _ _ _ _ _ TRUE] -> w128
            tunnel: w127 -> [_ w148 w166 w185 w204 w266 w352 w405 w464 w517 w564 w581 w603 w630 w643 w698 w718 w790 w818 w842 w898 w944 w1080 w1107 w1133 w1166 w1171 w1183 w1213]
            tunnel: w126 -> [_ _ _ _ _ _ _ _ _ _ _ _ _ _ _ _ _ _ _ _ _ _ _ w1111 _ _ _ _ _]
            tunnel: [_ _ w157 w176 w195 w215 w350 w406 w465 w513 w560 w565 _ _ _ _ _ _ w798 _ w885 _ _ _ _ _ _ _ _] -> w120
            tunnel: w119 -> [_ _ w158 w177 w196 w215 w350 w406 w465 w513 w560 w565 _ _ _ _ _ _ _ _ w886 _ _ _ _ _ _ _ _]
            tunnel: [_ _ _ _ _ _ _ _ _ _ _ _ _ _ _ _ _ _ _ _ _ _ _ w1108 _ _ _ _ _] -> w118
            tunnel: [_ _ _ _ _ _ _ _ _ _ _ _ _ _ _ _ _ _ _ _ _ _ _ w1090 _ _ _ _ _] -> w117
            tunnel: w106 -> [_ w155 _ _ _ _ _ _ _ _ _ _ _ _ _ _ _ _ _ _ _ _ _ _ _ _ _ _ _]
            tunnel: [_ w154 _ _ _ _ _ _ _ _ _ _ _ _ _ _ _ _ _ _ _ _ _ _ _ _ _ _ _] -> w105
            tunnel: w104 -> [_ _ _ _ _ _ _ _ _ _ _ _ _ _ _ _ _ _ _ w846 w902 _ _ _ _ _ _ _ _]
            tunnel: w103 -> [_ _ _ _ _ _ _ _ _ _ _ _ _ _ _ _ _ _ _ w847 w903 _ _ _ _ _ _ _ _]
            tunnel: w102 -> [_ _ _ _ _ _ _ _ _ _ _ _ _ _ _ _ _ _ _ w844 w900 _ _ _ _ _ _ _ _]
            tunnel: w101 -> [_ _ _ _ _ _ _ _ _ _ _ _ _ _ _ _ _ _ _ w845 w901 _ _ _ _ _ _ _ _]
            tunnel: w100 -> [_ _ _ _ _ _ _ _ _ _ _ _ _ _ _ _ _ _ _ w832 w888 _ _ _ _ _ _ _ _]
            tunnel: w99 -> [_ _ _ _ _ _ _ _ _ _ _ _ _ _ _ _ _ _ _ w831 w887 _ _ _ _ _ _ _ _]
            tunnel: [_ _ _ _ _ _ _ _ _ _ _ _ _ _ _ _ _ _ w800 w832 w888 _ _ _ _ _ _ _ _] -> w98
            tunnel: [_ _ _ _ _ _ _ _ _ _ _ _ _ _ _ _ _ _ w799 w831 w887 _ _ _ _ _ _ _ _] -> w97
            tunnel: w96 -> [_ _ _ _ _ _ _ _ _ _ _ _ w593 _ w664 w700 _ _ _ _ w884 _ _ _ _ _ _ w1178 _]
            tunnel: w95 -> [_ _ _ _ _ _ _ _ _ _ _ _ w592 _ w663 w699 _ _ _ _ w883 _ _ _ _ _ _ w1177 _]
            tunnel: w94 -> [_ _ _ _ _ _ _ _ _ _ _ _ _ _ _ _ _ _ _ _ _ _ _ _ _ _ _ w1182 _]
            tunnel: [_ _ _ _ _ _ _ _ _ _ _ _ _ _ _ _ _ _ _ _ _ _ _ _ _ _ _ TRUE _] -> w93
            tunnel: w92 -> [_ _ _ _ _ _ _ _ _ _ _ _ _ _ _ _ _ _ _ _ _ _ _ _ _ _ _ w1180 _]
            tunnel: [_ _ _ _ _ _ _ _ _ _ _ _ _ _ _ _ _ _ _ _ _ _ _ _ _ _ _ w1179 _] -> w91
            frame "Init", Default {
              w133 = FALSE ("RewCalib_Trig_L")
              w130 = u16 100 ("new element/subarray")
              # "Tdelay_R"
              # "Tdelay_L"
              # "RewCalib_N__R"
              # "RewCalib_N__L"
              # "Solenoid_Tcycle_R"
              # "Solenoid_Tcycle_L"
              # "Laser_Tcycle"
              # "Audio_Tcycle_R"
              # "Audio_Tcycle_L"
              # "initialize dataMTrig"
              n36 = call "myRIO_BRig_RT_dataMTrig_Solenoid_Tcycle__L.vi"() -> ("output_Solenoid_Tcycle__L"=w141:i32)  [unwired: 11 in]
              n37 = call "myRIO_BRig_RT_dataMTrig_Solenoid_Tcycle__R.vi"() -> ("output_Solenoid_Tcycle__R"=w142:i32)  [unwired: 11 in]
              n38 = call "myRIO_BRig_RT_dataMTrig_Audio_Tcycle__L.vi"() -> ("output_Audio_Tcycle__L"=w143:i32)  [unwired: 11 in]
              n39 = call "myRIO_BRig_RT_dataMTrig_Audio_Tcycle__R.vi"() -> ("output_Audio_Tcycle__R"=w144:i32)  [unwired: 11 in]
              n40 = call "myRIO_BRig_RT_dataMTrig_Laser_Tcycle.vi"() -> ("output_Laser_Tcycle"=w145:i32)  [unwired: 11 in]
              n41 = call "myRIO_BRig_RT_dataMTrig_Solenoid_RewCalib_nCycle__L.vi"() -> ("output_Solenoid_RewCalib_nCycle__L"=w137:i32)  [unwired: 11 in]
              n42 = call "myRIO_BRig_RT_dataMTrig_Solenoid_RewCalib_nCycle__R.vi"() -> ("output_Solenoid_RewCalib_nCycle__R"=w136:i32)  [unwired: 11 in]
              n43 = call "myRIO_BRig_RT_dataMTrig_Solenoid_Tdelay__L.vi"() -> ("output_Solenoid_Tdelay__L"=w135:i32)  [unwired: 11 in]
              n44 = call "myRIO_BRig_RT_dataMTrig_Solenoid_Tdelay__R.vi"() -> ("output_Solenoid_Tdelay__R"=w134:i32)  [unwired: 11 in]
              n45 = local read "MTrig_Solenoid_Tcycle__L"() -> (w146:u16)
              n46 = local read "MTrig_Solenoid_Tcycle__R"() -> (w147:u16)
              n47 = local read "MTrig_Laser_Tcycle"() -> (w131:u16)
              n48 = call "myRIO_BRig_RT_dataMTrig_init.vi"() -> ("output_dataMTrig"=w140:u16[])  [unwired: 5 in]
              n49 = local write "RewCalib_Trig_R"(w133) -> ()
              n50 = local write "RewCalib_Trig_L"(w133) -> ()
              n51 = local read "Tcycle_Cue_min"() -> (w132:u16)
              n52 = Replace Array Subset(array=w140, new element #1=w146, index #1=w141, new element #2=w147, index #2=w142, new element #3=w132, index #3=w143, new element #4=w132, index #4=w144, new element #5=w131, index #5=w145, new element #6=w130, index #6=w137, new element #7=w130, index #7=w136, new element #8=w130, index #8=w135, new element #9=w130, index #9=w134) -> (w139:u16[])
            }
            frame "UploadSettings_pre" {
              # "When the Host sends settings,\nnot all files send at the same time.\n\nIf RT reads the settings faster\nthan the Host can send them,\nthen we will skip settings.\n\nSolution:\nWait 20 cycles"
              n53 = Increment(x=w155) -> (x+1=w154:u16)
              n54 = Greater?(x=w154, y=u16 20) -> (0:w152:bool)
              n55 = Select(t=myRIO_BRig_RT__Case_NonExp_stateList."UploadSettings_Read_dataExp", s=w152, f=w151) -> (s? t:f=w149:T1)
            }
            frame "UploadSettings_Read_dataExp" {
              # "grab dataExp and\nstore it in the\ngeneric data array"
              # "dataExp"
              n56 = call "myRIO_BRig_RT_dataExp_init_details.vi"() -> ("output_dataSize"=w162:i32, "output_dataName"=w165:string)  [unwired: 10 in]
              n57 = call "myRIO_BRig_RT_comm_webdav_uploadReceived_check.vi"("input_dataName"=w165) -> ("output_Iexist"=w164:bool, "output_dataPath"=w163:path)  [unwired: 9 in]
              n58 = case shown="True" w164 {
                tunnel: w163 -> [_ w174]
                tunnel: w162 -> [_ w173]
                tunnel: [_ w172] -> w161
                tunnel: w158 -> [w167 w171]
                tunnel: [w167 w168] -> w157
                frame False {
                }
                frame True {
                  n59 = call "myRIO_BRig_RT_comm_webdav_uploadReceived_read.vi"("input_dataSize"=w173, "input_filePath"=w174) -> ("output_Ivalid"=w172:bool, "output_data"=w170:i64[])  [unwired: 8 in]
                  n60 = To Unsigned Word Integer(number=w170) -> (unsigned 16bit integer=w169:u16[])
                  n61 = Select(t=w169, s=w172, f=w171) -> (s? t:f=w168:u16[])
                }
              }
              n62 = Select(t=myRIO_BRig_RT__Case_NonExp_stateList."UploadSettings_dataExp_1", s=w161, f=myRIO_BRig_RT__Case_NonExp_stateList."UploadSettings_Read_dataLC" ("t")) -> (s? t:f=w156:T1)
            }
            frame "UploadSettings_Read_dataLC" {
              # "grab dataLC and\nstore it in the\ngeneric data array"
              # "dataLC"
              n63 = call "myRIO_BRig_RT_dataLC_init_details.vi"() -> ("output_dataSize"=w181:i32, "output_dataName"=w184:string)  [unwired: 10 in]
              n64 = call "myRIO_BRig_RT_comm_webdav_uploadReceived_check.vi"("input_dataName"=w184) -> ("output_Iexist"=w183:bool, "output_dataPath"=w182:path)  [unwired: 9 in]
              n65 = case shown="True" w183 {
                tunnel: w182 -> [_ w193]
                tunnel: w181 -> [_ w192]
                tunnel: [_ w191] -> w180
                tunnel: w177 -> [w186 w190]
                tunnel: [w186 w187] -> w176
                frame False {
                }
                frame True {
                  n66 = call "myRIO_BRig_RT_comm_webdav_uploadReceived_read.vi"("input_dataSize"=w192, "input_filePath"=w193) -> ("output_Ivalid"=w191:bool, "output_data"=w189:i64[])  [unwired: 8 in]
                  n67 = To Unsigned Word Integer(number=w189) -> (unsigned 16bit integer=w188:u16[])
                  n68 = Select(t=w188, s=w191, f=w190) -> (s? t:f=w187:u16[])
                }
              }
              n69 = Select(t=myRIO_BRig_RT__Case_NonExp_stateList."UploadSettings_dataLC_1", s=w180, f=myRIO_BRig_RT__Case_NonExp_stateList."UploadSettings_Read_dataMTrig" ("t")) -> (s? t:f=w175:T1)
            }
            frame "UploadSettings_Read_dataMTrig" {
              # "grab dataMTrig and\nstore it in the\ngeneric data array"
              # "dataMTrig"
              n70 = call "myRIO_BRig_RT_dataMTrig_init_details.vi"() -> ("output_dataSize"=w200:i32, "output_dataName"=w203:string)  [unwired: 10 in]
              n71 = call "myRIO_BRig_RT_comm_webdav_uploadReceived_check.vi"("input_dataName"=w203) -> ("output_Iexist"=w202:bool, "output_dataPath"=w201:path)  [unwired: 9 in]
              n72 = case shown="True" w202 {
                tunnel: w201 -> [_ w212]
                tunnel: w200 -> [_ w211]
                tunnel: [_ w210] -> w199
                tunnel: w196 -> [w205 w209]
                tunnel: [w205 w206] -> w195
                frame False {
                }
                frame True {
                  n73 = call "myRIO_BRig_RT_comm_webdav_uploadReceived_read.vi"("input_dataSize"=w211, "input_filePath"=w212) -> ("output_Ivalid"=w210:bool, "output_data"=w208:i64[])  [unwired: 8 in]
                  n74 = To Unsigned Word Integer(number=w208) -> (unsigned 16bit integer=w207:u16[])
                  n75 = Select(t=w207, s=w210, f=w209) -> (s? t:f=w206:u16[])
                }
              }
              n76 = Select(t=myRIO_BRig_RT__Case_NonExp_stateList."UploadSettings_dataMTrig_1", s=w199, f=myRIO_BRig_RT__Case_NonExp_stateList."Idle" ("t")) -> (s? t:f=w194:T1)
            }
            frame "UploadSettings_dataExp_1" {
              # "Cue_max"
              # "Cue_min"
              # "CuePenalty"
              # "Timeout"
              # "Wrong"
              # "Selection"
              # "RewardPost"
              # "Reward_R"
              # "Reward_L"
              # "Tcycle"
              # "TPB_min_R"
              # "TPB_min_L"
              # "TPB_max_R"
              # "TPB_max_L"
              # "I_trialUntilReward"
              # "ENL_penalty"
              # "ENL_min"
              # "ENL_max"
              # "BUR_max"
              # "BUR_min"
              # "CueCycles"
              # "Audio_Freq_R"
              # "Audio_Freq_L"
              # "Audio_Amp_R"
              # "Audio_Amp_L"
              n77 = call "myRIO_BRig_RT_dataExp_CueCycles.vi"() -> ("output_CueCycles"=w258:i32)  [unwired: 11 in]
              n78 = call "myRIO_BRig_RT_dataExp_Audio_amp__R.vi"() -> ("output_Audio_amp__R"=w262:i32)  [unwired: 11 in]
              n79 = call "myRIO_BRig_RT_dataExp_Audio_amp__L.vi"() -> ("output_Audio_amp__L"=w264:i32)  [unwired: 11 in]
              n80 = call "myRIO_BRig_RT_dataExp_Tcycle_Reward__L.vi"() -> ("output_Tcycle_Reward__L"=w235:i32)  [unwired: 11 in]
              n81 = call "myRIO_BRig_RT_dataExp_Tcycle_Reward__R.vi"() -> ("output_Tcycle_Reward__R"=w234:i32)  [unwired: 11 in]
              n82 = call "myRIO_BRig_RT_dataExp_Tcycle_RewardPost.vi"() -> ("output_Tcycle_RewardPost"=w233:i32)  [unwired: 11 in]
              n83 = call "myRIO_BRig_RT_dataExp_BUR_min.vi"() -> ("output_BUR_min"=w255:i32)  [unwired: 11 in]
              n84 = call "myRIO_BRig_RT_dataExp_ENL_min.vi"() -> ("output_ENL_min"=w251:i32)  [unwired: 11 in]
              n85 = call "myRIO_BRig_RT_dataExp_TPB_max__L.vi"() -> ("output_TPB_max__L"=w243:i32)  [unwired: 11 in]
              n86 = call "myRIO_BRig_RT_dataExp_TPB_max__R.vi"() -> ("output_TPB_max__R"=w242:i32)  [unwired: 11 in]
              n87 = call "myRIO_BRig_RT_dataExp_ENL_penalty.vi"() -> ("output_ENL_penalty"=w250:i32)  [unwired: 11 in]
              n88 = call "myRIO_BRig_RT_dataExp_Audio_freq__L.vi"() -> ("output_Audio_freq__L"=w260:i32)  [unwired: 11 in]
              n89 = call "myRIO_BRig_RT_dataExp_Audio_freq__R.vi"() -> ("output_Audio_freq__R"=w259:i32)  [unwired: 11 in]
              n90 = call "myRIO_BRig_RT_dataExp_BUR_max.vi"() -> ("output_BUR_max"=w256:i32)  [unwired: 11 in]
              n91 = call "myRIO_BRig_RT_dataExp_ENL_max.vi"() -> ("output_ENL_max"=w252:i32)  [unwired: 11 in]
              n92 = call "myRIO_BRig_RT_dataExp_ItrialUntilReward.vi"() -> ("output_I_trialUntilReward"=w246:i32)  [unwired: 11 in]
              n93 = call "myRIO_BRig_RT_dataExp_Tcycle_Selection.vi"() -> ("output_Tcycle_Selection"=w232:i32)  [unwired: 11 in]
              n94 = call "myRIO_BRig_RT_dataExp_Tcycle_Wrong.vi"() -> ("output_Tcycle_Wrong"=w231:i32)  [unwired: 11 in]
              n95 = call "myRIO_BRig_RT_dataExp_Tcycle_Timeout.vi"() -> ("output_Tcycle_Timeout"=w230:i32)  [unwired: 11 in]
              n96 = call "myRIO_BRig_RT_dataExp_TPB_min__L.vi"() -> ("output_TPB_min__L"=w241:i32)  [unwired: 11 in]
              n97 = call "myRIO_BRig_RT_dataExp_TPB_min__R.vi"() -> ("output_TPB_min__R"=w240:i32)  [unwired: 11 in]
              n98 = call "myRIO_BRig_RT_dataExp_Tcycle_Cue1Penalty_Audio.vi"() -> ("output_Tcycle_Cue1Penalty_Audio"=w223:i32)  [unwired: 11 in]
              n99 = call "myRIO_BRig_RT_dataExp_Tcycle_Cue1_Audio_min.vi"() -> ("output_Tcycle_Cue1_Audio_min"=w222:i32)  [unwired: 11 in]
              n100 = call "myRIO_BRig_RT_dataExp_Tcycle_Cue1_Audio_max.vi"() -> ("output_Tcycle_Cue1_Audio_max"=w221:i32)  [unwired: 11 in]
              n101 = Index Array(array=w215, index #1=w264, index #2=w262, index #3=w260, index #4=w259, index #5=w258, index #6=w256, index #7=w255, index #8=w252, index #9=w251, index #10=w250, index #11=w246, index #12=w243, index #13=w242, index #14=w241, index #15=w240, index #16=w235, index #17=w234, index #18=w233, index #19=w232, index #20=w231, index #21=w230, index #22=w223, index #23=w222, index #24=w221) -> (element #1=w263:u16, element #2=w261:u16, element #3=w218:u16, element #4=w217:u16, element #5=w257:u16, element #6=w254:u16, element #7=w253:u16, element #8=w249:u16, element #9=w248:u16, element #10=w247:u16, element #11=w244:u16, element #12=w239:u16, element #13=w238:u16, element #14=w237:u16, element #15=w236:u16, element #16=w229:u16, element #17=w228:u16, element #18=w227:u16, element #19=w226:u16, element #20=w225:u16, element #21=w224:u16, element #22=w220:u16, element #23=w214:u16, element #24=w213:u16)
              n102 = local write "Tcycle_Selection"(w226) -> ()
              n103 = local write "Tcycle_Wrong"(w225) -> ()
              n104 = local write "Tcycle_Timeout"(w224) -> ()
              n105 = local write "Audio_Amp__L"(w263) -> ()
              n106 = local write "Audio_Amp__R"(w261) -> ()
              n107 = local write "Tcycle_ENLPenalty"(w247) -> ()
              n108 = local write "Tcycle_ENL_max"(w249) -> ()
              n109 = local write "TpB_Min_L"(w237) -> ()
              n110 = local write "TpB_Min_R"(w236) -> ()
              n111 = local write "Tcycle_CuePenalty"(w220) -> ()
              n112 = local write "Tcycle_Cue_min"(w214) -> ()
              n113 = local write "Tcycle_Cue_max"(w213) -> ()
              n114 = To Unsigned Byte Integer(number=w218) -> (unsigned 8bit integer=w219:u8)
              n115 = To Unsigned Byte Integer(number=w217) -> (unsigned 8bit integer=w216:u8)
              n116 = Not Equal To 0?(x=w244) -> (x != 0?=w245:bool)
              n117 = local write "Tcycle_Reward_L"(w229) -> ()
              n118 = local write "Tcycle_Reward_R"(w228) -> ()
              n119 = local write "Tcycle_RewardPost"(w227) -> ()
              n120 = local write "CueCycles"(w257) -> ()
              n121 = local write "BUR_min"(w253) -> ()
              n122 = local write "BUR_max"(w254) -> ()
              n123 = local write "Tcycle_ENL_min"(w248) -> ()
              n124 = local write "TpB_Max_L"(w239) -> ()
              n125 = local write "TpB_Max_R"(w238) -> ()
              n126 = local write "TrialUntilReward"(w245) -> ()
              n127 = local write "Audio_Freq__L"(w219) -> ()
              n128 = local write "Audio_Freq__R"(w216) -> ()
            }
            frame "UploadSettings_dataExp_2" {
              w286 = 100.0 ("y")
              n129 = call "myRIO_BRig_RT_dataExp_FPGA_f_count2ms.vi"() -> ("output_FPGA_f_count2ms"=w349:i32)  [unwired: 11 in]
              n130 = call "myRIO_BRig_RT_dataExp_laser1_Freq.vi"() -> ("output_laser1_Freq"=w337:i32)  [unwired: 11 in]
              n131 = call "myRIO_BRig_RT_dataExp_laser1_duration.vi"() -> ("output_laser1_duration"=w336:i32)  [unwired: 11 in]
              n132 = call "myRIO_BRig_RT_dataExp_laser1_Tpeak.vi"() -> ("output_laser1_Tpeak"=w335:i32)  [unwired: 11 in]
              n133 = call "myRIO_BRig_RT_dataExp_laser1_Tshutter.vi"() -> ("output_laser1_Tshutter"=w334:i32)  [unwired: 11 in]
              n134 = call "myRIO_BRig_RT_dataExp_laser1_Power_min.vi"() -> ("output_laser1_Power_min"=w333:i32)  [unwired: 11 in]
              n135 = call "myRIO_BRig_RT_dataExp_laser1_Power_max.vi"() -> ("output_laser1_Power_max"=w332:i32)  [unwired: 11 in]
              n136 = call "myRIO_BRig_RT_dataExp_laser1_Power_step.vi"() -> ("output_laser1_Power_step"=w331:i32)  [unwired: 11 in]
              n137 = call "myRIO_BRig_RT_dataExp_Cue1Param_CueType_Switch.vi"() -> ("output_Cue1Param_CueType_Switch"=w278:i32)  [unwired: 11 in]
              n138 = call "myRIO_BRig_RT_dataExp_Cue1Param_AudioLed_Count_Switch.vi"() -> ("output_Cue1Param_AudioLed_Count_Switch"=w277:i32)  [unwired: 11 in]
              n139 = call "myRIO_BRig_RT_dataExp_Cue1Param_AudioLed_Probability_Switch.vi"() -> ("output_Cue1Param_AudioLed_Probability_Switch"=w276:i32)  [unwired: 11 in]
              n140 = call "myRIO_BRig_RT_dataExp_SolenoidProbability_L.vi"() -> ("output_SolenoidProbability_L"=w282:i32)  [unwired: 11 in]
              n141 = call "myRIO_BRig_RT_dataExp_SolenoidProbability_R.vi"() -> ("output_SolenoidProbability_R"=w281:i32)  [unwired: 11 in]
              n142 = call "myRIO_BRig_RT_dataExp_Cue1Param_CueType_NS.vi"() -> ("output_Cue1Param_CueType_NS"=w275:i32)  [unwired: 11 in]
              n143 = call "myRIO_BRig_RT_dataExp_Cue1Param_AudioLed_Count_NS.vi"() -> ("output_Cue1Param_AudioLed_Count_NS"=w274:i32)  [unwired: 11 in]
              n144 = call "myRIO_BRig_RT_dataExp_Cue1Param_AudioLed_Probability_NS.vi"() -> ("output_Cue1Param_AudioLed_Probability_NS"=w273:i32)  [unwired: 11 in]
              n145 = call "myRIO_BRig_RT_dataExp_laser2_Freq.vi"() -> ("output_laser2_Freq"=w330:i32)  [unwired: 11 in]
              n146 = call "myRIO_BRig_RT_dataExp_laser2_duration.vi"() -> ("output_laser2_duration"=w329:i32)  [unwired: 11 in]
              n147 = call "myRIO_BRig_RT_dataExp_laser2_Tpeak.vi"() -> ("output_laser2_Tpeak"=w328:i32)  [unwired: 11 in]
              n148 = call "myRIO_BRig_RT_dataExp_laser2_Tshutter.vi"() -> ("output_laser2_Tshutter"=w327:i32)  [unwired: 11 in]
              n149 = call "myRIO_BRig_RT_dataExp_laser2_Power_min.vi"() -> ("output_laser2_Power_min"=w326:i32)  [unwired: 11 in]
              n150 = call "myRIO_BRig_RT_dataExp_laser2_Power_max.vi"() -> ("output_laser2_Power_max"=w325:i32)  [unwired: 11 in]
              n151 = call "myRIO_BRig_RT_dataExp_laser2_Power_step.vi"() -> ("output_laser2_Power_step"=w324:i32)  [unwired: 11 in]
              n152 = call "myRIO_BRig_RT_dataExp_CueLed_Freq.vi"() -> ("output_CueLed_Freq"=w293:i32)  [unwired: 11 in]
              n153 = call "myRIO_BRig_RT_dataExp_CueLed.vi"() -> ("output_CueLed"=w292:i32)  [unwired: 11 in]
              n154 = call "myRIO_BRig_RT_dataExp_CueLed_Tpeak.vi"() -> ("output_CueLed_Tpeak"=w291:i32)  [unwired: 11 in]
              n155 = Index Array(array=w350, index #1=w349, index #2=w337, index #3=w336, index #4=w335, index #5=w334, index #6=w333, index #7=w332, index #8=w331, index #9=w330, index #10=w329, index #11=w328, index #12=w327, index #13=w326, index #14=w325, index #15=w324, index #16=w293, index #17=w292, index #18=w291, index #19=w282, index #20=w281, index #21=w278, index #22=w277, index #23=w276, index #24=w275, index #25=w274, index #26=w273) -> (element #1=w348:u16, element #2=w323:u16, element #3=w322:u16, element #4=w321:u16, element #5=w320:u16, element #6=w319:u16, element #7=w309:u16, element #8=w308:u16, element #9=w304:u16, element #10=w303:u16, element #11=w302:u16, element #12=w301:u16, element #13=w300:u16, element #14=w295:u16, element #15=w294:u16, element #16=w285:u16, element #17=w284:u16, element #18=w283:u16, element #19=w280:u16, element #20=w279:u16, element #21=w272:u16, element #22=w271:u16, element #23=w270:u16, element #24=w269:u16, element #25=w268:u16, element #26=w267:u16)
              n156 = local write "Cue1Param_CueType_Switch"(w272) -> ()
              n157 = local write "Cue1Param_AudioLed_Count_Switch"(w271) -> ()
              n158 = local write "Cue1Param_AudioLed_Probability_Switch"(w270) -> ()
              n159 = local write "Cue1Param_CueType_NS"(w269) -> ()
              n160 = local write "Cue1Param_AudioLed_Count_NS"(w268) -> ()
              n161 = local write "Cue1Param_AudioLed_Probability_NS"(w267) -> ()
              n162 = To Double Precision Float(number=w348) -> (double precision float=w347:dbl)
              n163 = To Double Precision Float(number=w323) -> (double precision float=w345:dbl)
              n164 = To Double Precision Float(number=w321) -> (double precision float=w342:dbl)
              n165 = To Double Precision Float(number=w320) -> (double precision float=w341:dbl)
              n166 = To Double Precision Float(number=w319) -> (double precision float=w343:dbl)
              n167 = To Double Precision Float(number=w309) -> (double precision float=w314:dbl)
              n168 = To Double Precision Float(number=w308) -> (double precision float=w310:dbl)
              n169 = To Double Precision Float(number=w304) -> (double precision float=w315:dbl)
              n170 = To Double Precision Float(number=w302) -> (double precision float=w317:dbl)
              n171 = To Double Precision Float(number=w301) -> (double precision float=w318:dbl)
              n172 = To Double Precision Float(number=w300) -> (double precision float=w316:dbl)
              n173 = To Double Precision Float(number=w295) -> (double precision float=w298:dbl)
              n174 = To Double Precision Float(number=w294) -> (double precision float=w299:dbl)
              n175 = To Double Precision Float(number=w285) -> (double precision float=w290:dbl)
              n176 = To Double Precision Float(number=w283) -> (double precision float=w289:dbl)
              n177 = local write "SolenoidProbability_L"(w280) -> ()
              n178 = local write "SolenoidProbability_R"(w279) -> ()
              n179 = Divide(x=w347, y=w286) -> (x/y=w346:dbl)
              n180 = Divide(x=w345, y=w286) -> (x/y=w344:dbl)
              n181 = Divide(x=w342, y=w286) -> (x/y=w339:dbl)
              n182 = Divide(x=w341, y=w286) -> (x/y=w338:dbl)
              n183 = Divide(x=w343, y=w286) -> (x/y=w340:dbl)
              n184 = Divide(x=w314, y=w286) -> (x/y=w312:dbl)
              n185 = Divide(x=w310, y=w286) -> (x/y=w311:dbl)
              n186 = Divide(x=w315, y=w286) -> (x/y=w313:dbl)
              n187 = Divide(x=w317, y=w286) -> (x/y=w307:dbl)
              n188 = Divide(x=w318, y=w286) -> (x/y=w306:dbl)
              n189 = Divide(x=w316, y=w286) -> (x/y=w305:dbl)
              n190 = Divide(x=w298, y=w286) -> (x/y=w297:dbl)
              n191 = Divide(x=w299, y=w286) -> (x/y=w296:dbl)
              n192 = Divide(x=w290, y=w286) -> (x/y=w288:dbl)
              n193 = Divide(x=w289, y=w286) -> (x/y=w287:dbl)
              n194 = local write "FPGA_count2ms"(w346) -> ()
              n195 = local write "Laser_Freq_l1"(w344) -> ()
              n196 = local write "Laser_duration_l1"(w322) -> ()
              n197 = local write "Laser_Tpeak_l1"(w339) -> ()
              n198 = local write "Laser_Tshutter_l1"(w338) -> ()
              n199 = local write "Laser_power_min_l1"(w340) -> ()
              n200 = local write "Laser_power_max_l1"(w312) -> ()
              n201 = local write "Laser_power_step_l1"(w311) -> ()
              n202 = local write "Laser_Freq_l2"(w313) -> ()
              n203 = local write "Laser_duration_l2"(w303) -> ()
              n204 = local write "Laser_Tpeak_l2"(w307) -> ()
              n205 = local write "Laser_Tshutter_l2"(w306) -> ()
              n206 = local write "Laser_power_min_l2"(w305) -> ()
              n207 = local write "Laser_power_max_l2"(w297) -> ()
              n208 = local write "Laser_power_step_l2"(w296) -> ()
              n209 = local write "CueLed_Freq"(w288) -> ()
              n210 = local write "CueLed_duration"(w284) -> ()
              n211 = local write "CueLed_Tpeak"(w287) -> ()
            }
            frame "UploadSettings_dataLC_1" {
              # "Cue1_delayOpt_NonSwitch"
              # "ENL1_delayOpt_NonSwitch"
              # "Cue1_delayOpt_Switch"
              # "ENL1_delayOpt_Switch"
              # "Count"
              # "Tdelay"
              # "Prob"
              # "OnOff"
              # "Block"
              # "Count"
              # "Tdelay"
              # "Prob"
              # "OnOff"
              # "Block"
              # "Count"
              # "Tdelay"
              # "Prob"
              # "OnOff"
              # "Block"
              # "ENL1 Switch"
              # "Cue1 NonSwitch"
              # "Cue1 Switch"
              # "ENL1 NonSwitch"
              # "Count"
              # "Tdelay"
              # "Prob"
              # "OnOff"
              # "Block"
              n212 = call "myRIO_BRig_RT_dataLC_ENL1_OnOff_Switch_l1.vi"() -> ("output_ENL1_OnOff_Switch_l1"=w404:i32)  [unwired: 11 in]
              n213 = call "myRIO_BRig_RT_dataLC_ENL1_Tdelay_Switch_l1.vi"() -> ("output_ENL1_Tdelay_Switch_l1"=w403:i32)  [unwired: 11 in]
              n214 = call "myRIO_BRig_RT_dataLC_ENL1_Block_Switch_l1.vi"() -> ("output_ENL1_Block_Switch_l1"=w402:i32)  [unwired: 11 in]
              n215 = call "myRIO_BRig_RT_dataLC_ENL1_Count_Switch_l1.vi"() -> ("output_ENL1_Count_Switch_l1"=w401:i32)  [unwired: 11 in]
              n216 = call "myRIO_BRig_RT_dataLC_ENL1_Probability_Switch_l1.vi"() -> ("output_ENL1_Probability_Switch_l1"=w400:i32)  [unwired: 11 in]
              n217 = call "myRIO_BRig_RT_dataLC_ENL1_OnOff_NS_l1.vi"() -> ("output_ENL1_OnOff_NS_l1"=w399:i32)  [unwired: 11 in]
              n218 = call "myRIO_BRig_RT_dataLC_ENL1_Tdelay_NS_l1.vi"() -> ("output_ENL1_Tdelay_NS_l1"=w398:i32)  [unwired: 11 in]
              n219 = call "myRIO_BRig_RT_dataLC_ENL1_Block_NS_l1.vi"() -> ("output_ENL1_All_Block"=w397:i32)  [unwired: 11 in]
              n220 = call "myRIO_BRig_RT_dataLC_ENL1_Count_NS_l1.vi"() -> ("output_ENL1_Count_NS_l1"=w396:i32)  [unwired: 11 in]
              n221 = call "myRIO_BRig_RT_dataLC_ENL1_Probability_NS_l1.vi"() -> ("output_ENL1_Probability_NS_l1"=w395:i32)  [unwired: 11 in]
              n222 = call "myRIO_BRig_RT_dataLC_Cue1_OnOff_Switch_l1.vi"() -> ("output_Cue1_OnOff_Switch_l1"=w394:i32)  [unwired: 11 in]
              n223 = call "myRIO_BRig_RT_dataLC_Cue1_Tdelay_Switch_l1.vi"() -> ("output_Cue1_Tdelay_Switch_l1"=w393:i32)  [unwired: 11 in]
              n224 = call "myRIO_BRig_RT_dataLC_Cue1_Block_Switch_l1.vi"() -> ("output_Cue1_Block_Switch_l1"=w392:i32)  [unwired: 11 in]
              n225 = call "myRIO_BRig_RT_dataLC_Cue1_Count_Switch_l1.vi"() -> ("output_Cue1_Count_Switch_l1"=w391:i32)  [unwired: 11 in]
              n226 = call "myRIO_BRig_RT_dataLC_Cue1_Probability_Switch_l1.vi"() -> ("output_Cue1_Probability_Switch_l1"=w390:i32)  [unwired: 11 in]
              n227 = call "myRIO_BRig_RT_dataLC_Cue1_OnOff_NS_l1.vi"() -> ("output_Cue1_OnOff_NS_l1"=w389:i32)  [unwired: 11 in]
              n228 = call "myRIO_BRig_RT_dataLC_Cue1_Tdelay_NS_l1.vi"() -> ("output_Cue1_Tdelay_NS_l1"=w388:i32)  [unwired: 11 in]
              n229 = call "myRIO_BRig_RT_dataLC_Cue1_Block_NS_l1.vi"() -> ("output_Cue1_Block_NS_l1"=w387:i32)  [unwired: 11 in]
              n230 = call "myRIO_BRig_RT_dataLC_Cue1_Count_NS_l1.vi"() -> ("output_Cue1_Count_NS_l1"=w386:i32)  [unwired: 11 in]
              n231 = call "myRIO_BRig_RT_dataLC_Cue1_Probability_NS_l1.vi"() -> ("output_Cue1_l1_All_Probability"=w385:i32)  [unwired: 11 in]
              n232 = call "myRIO_BRig_RT_dataLC_ENL1_delayOpt_Switch_l1.vi"() -> ("output_ENL1_delayOpt_Switch_l1"=w364:i32)  [unwired: 11 in]
              n233 = call "myRIO_BRig_RT_dataLC_ENL1_delayOpt_NS_l1.vi"() -> ("output_ENL1_delayOpt_NS_l1"=w363:i32)  [unwired: 11 in]
              n234 = call "myRIO_BRig_RT_dataLC_Cue1_delayOpt_Switch_l1.vi"() -> ("output_Cue1_delayOpt_Switch_l1"=w362:i32)  [unwired: 11 in]
              n235 = call "myRIO_BRig_RT_dataLC_Cue1_delayOpt_NS_l1.vi"() -> ("output_Cue1_delayOpt_NS_l1"=w361:i32)  [unwired: 11 in]
              n236 = Index Array(array=w406, index #1=w404, index #2=w403, index #3=w402, index #4=w401, index #5=w400, index #6=w399, index #7=w398, index #8=w397, index #9=w396, index #10=w395, index #11=w394, index #12=w393, index #13=w392, index #14=w391, index #15=w390, index #16=w389, index #17=w388, index #18=w387, index #19=w386, index #20=w385, index #21=w364, index #22=w363, index #23=w362, index #24=w361) -> (element #1=w384:u16, element #2=w383:u16, element #3=w382:u16, element #4=w381:u16, element #5=w380:u16, element #6=w379:u16, element #7=w378:u16, element #8=w377:u16, element #9=w376:u16, element #10=w375:u16, element #11=w374:u16, element #12=w373:u16, element #13=w372:u16, element #14=w371:u16, element #15=w370:u16, element #16=w369:u16, element #17=w368:u16, element #18=w367:u16, element #19=w366:u16, element #20=w365:u16, element #21=w356:u16, element #22=w355:u16, element #23=w354:u16, element #24=w353:u16)
              n237 = Not Equal To 0?(x=w384) -> (x != 0?=w408:bool)
              n238 = Not Equal To 0?(x=w379) -> (x != 0?=w407:bool)
              n239 = Not Equal To 0?(x=w374) -> (x != 0?=w410:bool)
              n240 = Not Equal To 0?(x=w369) -> (x != 0?=w409:bool)
              n241 = Not Equal To 0?(x=w356) -> (x != 0?=w358:bool)
              n242 = Not Equal To 0?(x=w355) -> (x != 0?=w359:bool)
              n243 = Not Equal To 0?(x=w354) -> (x != 0?=w360:bool)
              n244 = Not Equal To 0?(x=w353) -> (x != 0?=w357:bool)
              n245 = local write "LC_ENL1_OnOff_Switch_l1"(w408) -> ()
              n246 = local write "LC_ENL1_Tdelay_Switch_l1"(w383) -> ()
              n247 = local write "LC_ENL1_Block_Switch_l1"(w382) -> ()
              n248 = local write "LC_ENL1_Count_Switch_l1"(w381) -> ()
              n249 = local write "LC_ENL1_Probability_Switch_l1"(w380) -> ()
              n250 = local write "LC_ENL1_OnOff_NS_l1"(w407) -> ()
              n251 = local write "LC_ENL1_Tdelay_NS_l1"(w378) -> ()
              n252 = local write "LC_ENL1_Block_NS_l1"(w377) -> ()
              n253 = local write "LC_ENL1_Count_NS_l1"(w376) -> ()
              n254 = local write "LC_ENL1_Probability_NS_l1"(w375) -> ()
              n255 = local write "LC_Cue1_OnOff_Switch_l1"(w410) -> ()
              n256 = local write "LC_Cue1_Tdelay_Switch_l1"(w373) -> ()
              n257 = local write "LC_Cue1_Block_Switch_l1"(w372) -> ()
              n258 = local write "LC_Cue1_Count_Switch_l1"(w371) -> ()
              n259 = local write "LC_Cue1_Probability_Switch_l1"(w370) -> ()
              n260 = local write "LC_Cue1_OnOff_NS_l1"(w409) -> ()
              n261 = local write "LC_Cue1_Tdelay_NS_l1"(w368) -> ()
              n262 = local write "LC_Cue1_Block_NS_l1"(w367) -> ()
              n263 = local write "LC_Cue1_Count_NS_l1"(w366) -> ()
              n264 = local write "LC_Cue1_Probability_NS_l1"(w365) -> ()
              n265 = local write "LC_ENL1_delayOpt_Switch_l1"(w358) -> ()
              n266 = local write "LC_ENL1_delayOpt_NS_l1"(w359) -> ()
              n267 = local write "LC_Cue1_delayOpt_Switch_l1"(w360) -> ()
              n268 = local write "LC_Cue1_delayOpt_NS_l1"(w357) -> ()
            }
            frame "UploadSettings_dataLC_3" {
              # "Cue1_delayOpt_NonSwitch"
              # "ENL1_delayOpt_NonSwitch"
              # "Cue1_delayOpt_Switch"
              # "ENL1_delayOpt_Switch"
              # "Count"
              # "Tdelay"
              # "Prob"
              # "OnOff"
              # "Block"
              # "Count"
              # "Tdelay"
              # "Prob"
              # "OnOff"
              # "Block"
              # "Count"
              # "Tdelay"
              # "Prob"
              # "OnOff"
              # "Block"
              # "ENL1 Switch"
              # "Cue1 NonSwitch"
              # "Cue1 Switch"
              # "ENL1 NonSwitch"
              # "Count"
              # "Tdelay"
              # "Prob"
              # "OnOff"
              # "Block"
              n269 = call "myRIO_BRig_RT_dataLC_ENL1_OnOff_Switch_l2.vi"() -> ("output_ENL1_OnOff_Switch_l2"=w431:i32)  [unwired: 11 in]
              n270 = call "myRIO_BRig_RT_dataLC_ENL1_Tdelay_Switch_l2.vi"() -> ("output_ENL1_Tdelay_Switch_l2"=w432:i32)  [unwired: 11 in]
              n271 = call "myRIO_BRig_RT_dataLC_ENL1_Block_Switch_l2.vi"() -> ("output_ENL1_Block_Switch_l2"=w433:i32)  [unwired: 11 in]
              n272 = call "myRIO_BRig_RT_dataLC_ENL1_Count_Switch_l2.vi"() -> ("output_ENL1_Count_Switch_l2"=w434:i32)  [unwired: 11 in]
              n273 = call "myRIO_BRig_RT_dataLC_ENL1_Probability_Switch_l2.vi"() -> ("output_ENL1_Probability_Switch_l2"=w435:i32)  [unwired: 11 in]
              n274 = call "myRIO_BRig_RT_dataLC_ENL1_OnOff_NS_l2.vi"() -> ("output_ENL1_OnOff_NS_l2"=w426:i32)  [unwired: 11 in]
              n275 = call "myRIO_BRig_RT_dataLC_ENL1_Tdelay_NS_l2.vi"() -> ("output_ENL1_Tdelay_NS_l2"=w427:i32)  [unwired: 11 in]
              n276 = call "myRIO_BRig_RT_dataLC_ENL1_Block_NS_l2.vi"() -> ("output_ENL1_Block_NS_l2"=w428:i32)  [unwired: 11 in]
              n277 = call "myRIO_BRig_RT_dataLC_ENL1_Count_NS_l2.vi"() -> ("output_ENL1_Count_NS_l2"=w429:i32)  [unwired: 11 in]
              n278 = call "myRIO_BRig_RT_dataLC_ENL1_Probability_NS_l2.vi"() -> ("output_ENL1_Probability_NS_l2"=w430:i32)  [unwired: 11 in]
              n279 = call "myRIO_BRig_RT_dataLC_Cue1_OnOff_Switch_l2.vi"() -> ("output_Cue1_OnOff_Switch_l2"=w421:i32)  [unwired: 11 in]
              n280 = call "myRIO_BRig_RT_dataLC_Cue1_Tdelay_Switch_l2.vi"() -> ("output_Cue1_Tdelay_Switch_l2"=w422:i32)  [unwired: 11 in]
              n281 = call "myRIO_BRig_RT_dataLC_Cue1_Block_Switch_l2.vi"() -> ("output_Cue1_Block_Switch_l2"=w423:i32)  [unwired: 11 in]
              n282 = call "myRIO_BRig_RT_dataLC_Cue1_Count_Switch_l2.vi"() -> ("output_Cue1_Count_Switch_l2"=w424:i32)  [unwired: 11 in]
              n283 = call "myRIO_BRig_RT_dataLC_Cue1_Probability_Switch_l2.vi"() -> ("output_Cue1_l2_First_Probability"=w425:i32)  [unwired: 11 in]
              n284 = call "myRIO_BRig_RT_dataLC_Cue1_OnOff_NS_l2.vi"() -> ("output_Cue1_OnOff_NS_l2"=w416:i32)  [unwired: 11 in]
              n285 = call "myRIO_BRig_RT_dataLC_Cue1_Tdelay_NS_l2.vi"() -> ("output_Cue1_Tdelay_NS_l2"=w417:i32)  [unwired: 11 in]
              n286 = call "myRIO_BRig_RT_dataLC_Cue1_Block_NS_l2.vi"() -> ("output_Cue1_Block_NS_l2"=w418:i32)  [unwired: 11 in]
              n287 = call "myRIO_BRig_RT_dataLC_Cue1_Count_NS_l2.vi"() -> ("output_Cue1_Count_NS_l2"=w419:i32)  [unwired: 11 in]
              n288 = call "myRIO_BRig_RT_dataLC_Cue1_Probability_NS_l2.vi"() -> ("output_Cue1_l2_All_Probability"=w420:i32)  [unwired: 11 in]
              n289 = call "myRIO_BRig_RT_dataLC_ENL1_delayOpt_Switch_l2.vi"() -> ("output_ENL1_delayOpt_Switch_l2"=w412:i32)  [unwired: 11 in]
              n290 = call "myRIO_BRig_RT_dataLC_ENL1_delayOpt_NS_l2.vi"() -> ("output_ENL1_delayOpt_NS_l2"=w413:i32)  [unwired: 11 in]
              n291 = call "myRIO_BRig_RT_dataLC_Cue1_delayOpt_Switch_l2.vi"() -> ("output_Cue1_delayOpt_Switch_l2"=w414:i32)  [unwired: 11 in]
              n292 = call "myRIO_BRig_RT_dataLC_Cue1_delayOpt_NS_l2.vi"() -> ("output_Cue1_delayOpt_NS_l2"=w415:i32)  [unwired: 11 in]
              n293 = Index Array(array=w465, index #1=w431, index #2=w432, index #3=w433, index #4=w434, index #5=w435, index #6=w426, index #7=w427, index #8=w428, index #9=w429, index #10=w430, index #11=w421, index #12=w422, index #13=w423, index #14=w424, index #15=w425, index #16=w416, index #17=w417, index #18=w418, index #19=w419, index #20=w420, index #21=w412, index #22=w413, index #23=w414, index #24=w415) -> (element #1=w463:u16, element #2=w462:u16, element #3=w461:u16, element #4=w460:u16, element #5=w459:u16, element #6=w458:u16, element #7=w457:u16, element #8=w456:u16, element #9=w455:u16, element #10=w454:u16, element #11=w453:u16, element #12=w452:u16, element #13=w451:u16, element #14=w450:u16, element #15=w449:u16, element #16=w448:u16, element #17=w447:u16, element #18=w446:u16, element #19=w445:u16, element #20=w444:u16, element #21=w439:u16, element #22=w438:u16, element #23=w437:u16, element #24=w436:u16)
              n294 = Not Equal To 0?(x=w463) -> (x != 0?=w467:bool)
              n295 = Not Equal To 0?(x=w458) -> (x != 0?=w466:bool)
              n296 = Not Equal To 0?(x=w453) -> (x != 0?=w469:bool)
              n297 = Not Equal To 0?(x=w448) -> (x != 0?=w468:bool)
              n298 = Not Equal To 0?(x=w439) -> (x != 0?=w441:bool)
              n299 = Not Equal To 0?(x=w438) -> (x != 0?=w442:bool)
              n300 = Not Equal To 0?(x=w437) -> (x != 0?=w443:bool)
              n301 = Not Equal To 0?(x=w436) -> (x != 0?=w440:bool)
              n302 = local write "LC_ENL1_OnOff_Switch_l2"(w467) -> ()
              n303 = local write "LC_ENL1_Tdelay_Switch_l2"(w462) -> ()
              n304 = local write "LC_ENL1_Block_Switch_l2"(w461) -> ()
              n305 = local write "LC_ENL1_Count_Switch_l2"(w460) -> ()
              n306 = local write "LC_ENL1_Probability_Switch_l2"(w459) -> ()
              n307 = local write "LC_ENL1_OnOff_NS_l2"(w466) -> ()
              n308 = local write "LC_ENL1_Tdelay_NS_l2"(w457) -> ()
              n309 = local write "LC_ENL1_Block_NS_l2"(w456) -> ()
              n310 = local write "LC_ENL1_Count_NS_l2"(w455) -> ()
              n311 = local write "LC_ENL1_Probability_NS_l2"(w454) -> ()
              n312 = local write "LC_Cue1_OnOff_Switch_l2"(w469) -> ()
              n313 = local write "LC_Cue1_Tdelay_Switch_l2"(w452) -> ()
              n314 = local write "LC_Cue1_Block_Switch_l2"(w451) -> ()
              n315 = local write "LC_Cue1_Count_Switch_l2"(w450) -> ()
              n316 = local write "LC_Cue1_Probability_Switch_l2"(w449) -> ()
              n317 = local write "LC_Cue1_OnOff_NS_l2"(w468) -> ()
              n318 = local write "LC_Cue1_Tdelay_NS_l2"(w447) -> ()
              n319 = local write "LC_Cue1_Block_NS_l2"(w446) -> ()
              n320 = local write "LC_Cue1_Count_NS_l2"(w445) -> ()
              n321 = local write "LC_Cue1_Probability_NS_l2"(w444) -> ()
              n322 = local write "LC_ENL1_delayOpt_Switch_l2"(w441) -> ()
              n323 = local write "LC_ENL1_delayOpt_NS_l2"(w442) -> ()
              n324 = local write "LC_Cue1_delayOpt_Switch_l2"(w443) -> ()
              n325 = local write "LC_Cue1_delayOpt_NS_l2"(w440) -> ()
            }
            frame "UploadSettings_dataLC_2" {
              # "Count"
              # "Tdelay"
              # "Prob"
              # "OnOff"
              # "Block"
              # "Selection NonSwitch"
              # "Count"
              # "Tdelay"
              # "Prob"
              # "OnOff"
              # "Block"
              # "Selection Switch"
              # "Trial"
              # "Tdelay"
              # "Prob"
              # "OnOff"
              # "Block"
              # "Wrong"
              # "Reward"
              # "Trial"
              # "Tdelay"
              # "Prob"
              # "OnOff"
              # "Block"
              n326 = call "myRIO_BRig_RT_dataLC_Reward_OnOff_l1.vi"() -> ("output_Reward_OnOff_l1"=w512:i32)  [unwired: 11 in]
              n327 = call "myRIO_BRig_RT_dataLC_Reward_Tdelay_l1.vi"() -> ("output_Reward_Tdelay_l1"=w511:i32)  [unwired: 11 in]
              n328 = call "myRIO_BRig_RT_dataLC_Reward_Block_l1.vi"() -> ("output_Reward_Block_l1"=w510:i32)  [unwired: 11 in]
              n329 = call "myRIO_BRig_RT_dataLC_Reward_Trial_l1.vi"() -> ("output_Reward_Trial_l1"=w509:i32)  [unwired: 11 in]
              n330 = call "myRIO_BRig_RT_dataLC_Reward_Probability_l1.vi"() -> ("output_Reward_Probability_l1"=w508:i32)  [unwired: 11 in]
              n331 = call "myRIO_BRig_RT_dataLC_Wrong_OnOff_l1.vi"() -> ("output_Wrong_OnOff_l1"=w501:i32)  [unwired: 11 in]
              n332 = call "myRIO_BRig_RT_dataLC_Wrong_Tdelay_l1.vi"() -> ("output_Wrong_Tdelay_l1"=w500:i32)  [unwired: 11 in]
              n333 = call "myRIO_BRig_RT_dataLC_Wrong_Block_l1.vi"() -> ("output_Wrong_Block_l1"=w499:i32)  [unwired: 11 in]
              n334 = call "myRIO_BRig_RT_dataLC_Wrong_Trial_l1.vi"() -> ("output_Wrong_Trial_l1"=w498:i32)  [unwired: 11 in]
              n335 = call "myRIO_BRig_RT_dataLC_Wrong_Probability_l1.vi"() -> ("output_Wrong_Probability_l1"=w497:i32)  [unwired: 11 in]
              n336 = call "myRIO_BRig_RT_dataLC_Selection_OnOff_Switch_l1.vi"() -> ("output_Selection_OnOff_Switch_l1"=w492:i32)  [unwired: 11 in]
              n337 = call "myRIO_BRig_RT_dataLC_Selection_Tdelay_Switch_l1.vi"() -> ("output_Selection_Tdelay_Switch_l1"=w491:i32)  [unwired: 11 in]
              n338 = call "myRIO_BRig_RT_dataLC_Selection_Block_Switch_l1.vi"() -> ("output_Selection_Block_Switch_l1"=w490:i32)  [unwired: 11 in]
              n339 = call "myRIO_BRig_RT_dataLC_Selection_Count_Switch_l1.vi"() -> ("output_Selection_Count_Switch_l1"=w489:i32)  [unwired: 11 in]
              n340 = call "myRIO_BRig_RT_dataLC_Selection_Probability_Switch_l1.vi"() -> ("output_Selection_Probability_Switch_l1"=w488:i32)  [unwired: 11 in]
              n341 = call "myRIO_BRig_RT_dataLC_Selection_OnOff_NS_l1.vi"() -> ("output_Selection_OnOff_NS_l1"=w487:i32)  [unwired: 11 in]
              n342 = call "myRIO_BRig_RT_dataLC_Selection_Tdelay_NS_l1.vi"() -> ("output_Selection_Tdelay_NS_l1"=w486:i32)  [unwired: 11 in]
              n343 = call "myRIO_BRig_RT_dataLC_Selection_Block_NS_l1.vi"() -> ("output_Selection_Block_NS_l1"=w485:i32)  [unwired: 11 in]
              n344 = call "myRIO_BRig_RT_dataLC_Selection_Count_NS_l1.vi"() -> ("output_Selection_Count_NS_l1"=w484:i32)  [unwired: 11 in]
              n345 = call "myRIO_BRig_RT_dataLC_Selection_Probability_NS_l1.vi"() -> ("output_Selection_Probability_NS_l1"=w483:i32)  [unwired: 11 in]
              n346 = Index Array(array=w513, index #1=w512, index #2=w511, index #3=w510, index #4=w509, index #5=w508, index #6=w501, index #7=w500, index #8=w499, index #9=w498, index #10=w497, index #11=w492, index #12=w491, index #13=w490, index #14=w489, index #15=w488, index #16=w487, index #17=w486, index #18=w485, index #19=w484, index #20=w483) -> (element #1=w507:u16, element #2=w506:u16, element #3=w505:u16, element #4=w504:u16, element #5=w503:u16, element #6=w502:u16, element #7=w496:u16, element #8=w495:u16, element #9=w494:u16, element #10=w493:u16, element #11=w480:u16, element #12=w479:u16, element #13=w478:u16, element #14=w477:u16, element #15=w476:u16, element #16=w475:u16, element #17=w474:u16, element #18=w473:u16, element #19=w472:u16, element #20=w471:u16)
              n347 = Not Equal To 0?(x=w507) -> (x != 0?=w515:bool)
              n348 = Not Equal To 0?(x=w502) -> (x != 0?=w514:bool)
              n349 = Not Equal To 0?(x=w480) -> (x != 0?=w482:bool)
              n350 = Not Equal To 0?(x=w475) -> (x != 0?=w481:bool)
              n351 = local write "LC_Reward_OnOff_l1"(w515) -> ()
              n352 = local write "LC_Reward_Tdelay_l1"(w506) -> ()
              n353 = local write "LC_Reward_Block_l1"(w505) -> ()
              n354 = local write "LC_Reward_Trial_l1"(w504) -> ()
              n355 = local write "LC_Reward_Probability_l1"(w503) -> ()
              n356 = local write "LC_Wrong_OnOff_l1"(w514) -> ()
              n357 = local write "LC_Wrong_Tdelay_l1"(w496) -> ()
              n358 = local write "LC_Wrong_Block_l1"(w495) -> ()
              n359 = local write "LC_Wrong_Trial_l1"(w494) -> ()
              n360 = local write "LC_Wrong_Probability_l1"(w493) -> ()
              n361 = local write "LC_Sel_OnOff_Switch_l1"(w482) -> ()
              n362 = local write "LC_Sel_Tdelay_Switch_l1"(w479) -> ()
              n363 = local write "LC_Sel_Block_Switch_l1"(w478) -> ()
              n364 = local write "LC_Sel_Count_Switch_l1"(w477) -> ()
              n365 = local write "LC_Sel_Probability_Switch_l1"(w476) -> ()
              n366 = local write "LC_Sel_OnOff_NS_l1"(w481) -> ()
              n367 = local write "LC_Sel_Tdelay_NS_l1"(w474) -> ()
              n368 = local write "LC_Sel_Block_NS_l1"(w473) -> ()
              n369 = local write "LC_Sel_Count_NS_l1"(w472) -> ()
              n370 = local write "LC_Sel_Probability_NS_l1"(w471) -> ()
            }
            frame "UploadSettings_dataLC_4" {
              # "Count"
              # "Tdelay"
              # "Prob"
              # "OnOff"
              # "Block"
              # "Selection NonSwitch"
              # "Count"
              # "Tdelay"
              # "Prob"
              # "OnOff"
              # "Block"
              # "Selection Switch"
              # "Trial"
              # "Tdelay"
              # "Prob"
              # "OnOff"
              # "Block"
              # "Wrong"
              # "Reward"
              # "Trial"
              # "Tdelay"
              # "Prob"
              # "OnOff"
              # "Block"
              n371 = call "myRIO_BRig_RT_dataLC_Reward_OnOff_l2.vi"() -> ("output_Reward_OnOff_l2"=w523:i32)  [unwired: 11 in]
              n372 = call "myRIO_BRig_RT_dataLC_Reward_Tdelay_l2.vi"() -> ("output_Reward_Tdelay_l2"=w524:i32)  [unwired: 11 in]
              n373 = call "myRIO_BRig_RT_dataLC_Reward_Block_l2.vi"() -> ("output_Reward_Block_l2"=w525:i32)  [unwired: 11 in]
              n374 = call "myRIO_BRig_RT_dataLC_Reward_Trial_l2.vi"() -> ("output_Reward_Trial_l2"=w526:i32)  [unwired: 11 in]
              n375 = call "myRIO_BRig_RT_dataLC_Reward_Probability_l2.vi"() -> ("output_Reward_Probability_l2"=w527:i32)  [unwired: 11 in]
              n376 = call "myRIO_BRig_RT_dataLC_Wrong_OnOff_l2.vi"() -> ("output_Wrong_OnOff_l2"=w518:i32)  [unwired: 11 in]
              n377 = call "myRIO_BRig_RT_dataLC_Wrong_Tdelay_l2.vi"() -> ("output_Wrong_Tdelay_l2"=w519:i32)  [unwired: 11 in]
              n378 = call "myRIO_BRig_RT_dataLC_Wrong_Block_l2.vi"() -> ("output_Wrong_Block_l2"=w520:i32)  [unwired: 11 in]
              n379 = call "myRIO_BRig_RT_dataLC_Wrong_Trial_l2.vi"() -> ("output_Wrong_Trial_l2"=w521:i32)  [unwired: 11 in]
              n380 = call "myRIO_BRig_RT_dataLC_Wrong_Probability_l2.vi"() -> ("output_Wrong_Probability_l2"=w522:i32)  [unwired: 11 in]
              n381 = call "myRIO_BRig_RT_dataLC_Selection_OnOff_Switch_l2.vi"() -> ("output_Selection_OnOff_Switch_l2"=w533:i32)  [unwired: 11 in]
              n382 = call "myRIO_BRig_RT_dataLC_Selection_Tdelay_Switch_l2.vi"() -> ("output_Selection_Tdelay_Switch_l2"=w534:i32)  [unwired: 11 in]
              n383 = call "myRIO_BRig_RT_dataLC_Selection_Block_Switch_l2.vi"() -> ("output_Selection_Block_Switch_l2"=w535:i32)  [unwired: 11 in]
              n384 = call "myRIO_BRig_RT_dataLC_Selection_Count_Switch_l2.vi"() -> ("output_Selection_Count_Switch_l2"=w536:i32)  [unwired: 11 in]
              n385 = call "myRIO_BRig_RT_dataLC_Selection_Probability_Switch_l2.vi"() -> ("output_Selection_Probability_Switch_l1"=w537:i32)  [unwired: 11 in]
              n386 = call "myRIO_BRig_RT_dataLC_Selection_OnOff_NS_l2.vi"() -> ("output_Selection_OnOff_NS_l2"=w528:i32)  [unwired: 11 in]
              n387 = call "myRIO_BRig_RT_dataLC_Selection_Tdelay_NS_l2.vi"() -> ("output_Selection_Tdelay_NS_l2"=w529:i32)  [unwired: 11 in]
              n388 = call "myRIO_BRig_RT_dataLC_Selection_Block_NS_l2.vi"() -> ("output_Selection_Block_NS_l2"=w530:i32)  [unwired: 11 in]
              n389 = call "myRIO_BRig_RT_dataLC_Selection_Count_NS_l2.vi"() -> ("output_Selection_Count_NS_l2"=w531:i32)  [unwired: 11 in]
              n390 = call "myRIO_BRig_RT_dataLC_Selection_Probability_NS_l2.vi"() -> ("output_Selection_Probability_NS_l2"=w532:i32)  [unwired: 11 in]
              n391 = Index Array(array=w560, index #1=w523, index #2=w524, index #3=w525, index #4=w526, index #5=w527, index #6=w518, index #7=w519, index #8=w520, index #9=w521, index #10=w522, index #11=w533, index #12=w534, index #13=w535, index #14=w536, index #15=w537, index #16=w528, index #17=w529, index #18=w530, index #19=w531, index #20=w532) -> (element #1=w559:u16, element #2=w558:u16, element #3=w557:u16, element #4=w556:u16, element #5=w555:u16, element #6=w554:u16, element #7=w553:u16, element #8=w552:u16, element #9=w551:u16, element #10=w550:u16, element #11=w547:u16, element #12=w546:u16, element #13=w545:u16, element #14=w544:u16, element #15=w543:u16, element #16=w542:u16, element #17=w541:u16, element #18=w540:u16, element #19=w539:u16, element #20=w538:u16)
              n392 = Not Equal To 0?(x=w559) -> (x != 0?=w562:bool)
              n393 = Not Equal To 0?(x=w554) -> (x != 0?=w561:bool)
              n394 = Not Equal To 0?(x=w547) -> (x != 0?=w549:bool)
              n395 = Not Equal To 0?(x=w542) -> (x != 0?=w548:bool)
              n396 = local write "LC_Reward_OnOff_l2"(w562) -> ()
              n397 = local write "LC_Reward_Tdelay_l2"(w558) -> ()
              n398 = local write "LC_Reward_Block_l2"(w557) -> ()
              n399 = local write "LC_Reward_Trial_l2"(w556) -> ()
              n400 = local write "LC_Reward_Probability_l2"(w555) -> ()
              n401 = local write "LC_Wrong_OnOff_l2"(w561) -> ()
              n402 = local write "LC_Wrong_Tdelay_l2"(w553) -> ()
              n403 = local write "LC_Wrong_Block_l2"(w552) -> ()
              n404 = local write "LC_Wrong_Trial_l2"(w551) -> ()
              n405 = local write "LC_Wrong_Probability_l2"(w550) -> ()
              n406 = local write "LC_Sel_OnOff_Switch_l2"(w549) -> ()
              n407 = local write "LC_Sel_Tdelay_Switch_l2"(w546) -> ()
              n408 = local write "LC_Sel_Block_Switch_l2"(w545) -> ()
              n409 = local write "LC_Sel_Count_Switch_l2"(w544) -> ()
              n410 = local write "LC_Sel_Probability_Switch_l2"(w543) -> ()
              n411 = local write "LC_Sel_OnOff_NS_l2"(w548) -> ()
              n412 = local write "LC_Sel_Tdelay_NS_l2"(w541) -> ()
              n413 = local write "LC_Sel_Block_NS_l2"(w540) -> ()
              n414 = local write "LC_Sel_Count_NS_l2"(w539) -> ()
              n415 = local write "LC_Sel_Probability_NS_l2"(w538) -> ()
            }
            frame "UploadSettings_dataMTrig_1" {
              # "Tdelay_R"
              # "Tdelay_L"
              # "Tcycle_R"
              # "Tcycle_L"
              # "RewCalib_nCycle_R"
              # "RewCalib_nCycle_L"
              # "Solenoid"
              # "Laser_Tcycle"
              n416 = call "myRIO_BRig_RT_dataMTrig_Laser_Tcycle.vi"() -> ("output_Laser_Tcycle"=w572:i32)  [unwired: 11 in]
              n417 = call "myRIO_BRig_RT_dataMTrig_Solenoid_RewCalib_nCycle__L.vi"() -> ("output_Solenoid_RewCalib_nCycle__L"=w571:i32)  [unwired: 11 in]
              n418 = call "myRIO_BRig_RT_dataMTrig_Solenoid_RewCalib_nCycle__R.vi"() -> ("output_Solenoid_RewCalib_nCycle__R"=w570:i32)  [unwired: 11 in]
              n419 = call "myRIO_BRig_RT_dataMTrig_Solenoid_Tdelay__L.vi"() -> ("output_Solenoid_Tdelay__L"=w567:i32)  [unwired: 11 in]
              n420 = call "myRIO_BRig_RT_dataMTrig_Solenoid_Tdelay__R.vi"() -> ("output_Solenoid_Tdelay__R"=w566:i32)  [unwired: 11 in]
              n421 = call "myRIO_BRig_RT_dataMTrig_Solenoid_Tcycle__L.vi"() -> ("output_Solenoid_Tcycle__L"=w569:i32)  [unwired: 11 in]
              n422 = call "myRIO_BRig_RT_dataMTrig_Solenoid_Tcycle__R.vi"() -> ("output_Solenoid_Tcycle__R"=w568:i32)  [unwired: 11 in]
              n423 = Index Array(array=w565, index #1=w572, index #2=w571, index #3=w570, index #4=w569, index #5=w568, index #6=w567, index #7=w566) -> (element #1=w579:u16, element #2=w578:u16, element #3=w577:u16, element #4=w576:u16, element #5=w575:u16, element #6=w574:u16, element #7=w573:u16)
              n424 = Replace Array Subset(array=w581, new element #1=w579, index #1=w572, new element #2=w578, index #2=w571, new element #3=w577, index #3=w570, new element #4=w576, index #4=w569, new element #5=w575, index #5=w568, new element #6=w574, index #6=w567, new element #7=w573, index #7=w566) -> (w580:u16[])
              n425 = local write "MTrig_Solenoid_Tcycle__L"(w576) -> ()
              n426 = local write "MTrig_Solenoid_Tcycle__R"(w575) -> ()
              n427 = local write "MTrig_Laser_Tcycle"(w579) -> ()
            }
            frame "Idle" {
              # "To ensure timing, we split the\nidle state into 4 phases"
              # "Laser_Tcycle"
              # "Audio_Tcycle_R"
              # "Audio_Tcycle_L"
              n428 = local read "Laser_power_min_l1"() -> (w587:dbl)
              n429 = local read "Laser_power_min_l2"() -> (w585:dbl)
              n430 = local read "Audio_Amp__R"() -> (w589:u16)
              n431 = local read "Audio_Amp__L"() -> (w591:u16)
              n432 = local read "Audio_Freq__R"() -> (w588:u8)
              n433 = local read "Audio_Freq__L"() -> (w590:u8)
              n434 = Select(t=myRIO_BRig_RT__Case_NonExp_stateList."SendData" ("Enum"), s="SendData", f=myRIO_BRig_RT__Case_NonExp_stateList."Idle_2" ("Enum")) -> (s? t:f=w596:T1)
              n435 = call "myRIO__convert__Voltage_to_FPGAvalue.vi"("input_voltage"=w587) -> ("output_PortC"=w586:i16)  [unwired: 9 in, 1 out]
              n436 = call "myRIO__convert__Voltage_to_FPGAvalue.vi"("input_voltage"=w585) -> ("output_PortC"=w584:i16)  [unwired: 9 in, 1 out]
              n437 = Select(t=myRIO_BRig_RT__Case_NonExp_stateList."TestConnection" ("Enum"), s="TestConnection", f=w596) -> (s? t:f=w600:T1)
              n438 = xnode "Read/Write Control"("FPGA VI Reference In"=w593, "error in"=w592, "audioAmp_L"=w591, "audioFreq_L_kHz"=w590, "audioAmp_R"=w589, "audioFreq_R_kHz"=w588, "AnaOut_0"=w586, "AnaOut_1"=w584) -> ("error out"=w583:errorcluster)  [unwired: 1 out]
              n439 = local write "error out"(w583) -> ()
              n440 = call "myRIO_BRig_RT_dataMTrig_Audio_Tcycle__L.vi"() -> ("output_Audio_Tcycle__L"=w607:i32)  [unwired: 11 in]
              n441 = call "myRIO_BRig_RT_dataMTrig_Audio_Tcycle__R.vi"() -> ("output_Audio_Tcycle__R"=w606:i32)  [unwired: 11 in]
              n442 = call "myRIO_BRig_RT_dataMTrig_Laser_Tcycle.vi"() -> ("output_Laser_Tcycle"=w605:i32)  [unwired: 11 in]
              n443 = local read "MTrig_Laser_Tcycle"() -> (w594:u16)
              n444 = local read "Tcycle_Cue_min"() -> (w595:u16)
              n445 = Replace Array Subset(array=w603, new element #1=w595, index #1=w607, new element #2=w595, index #2=w606, new element #3=w594, index #3=w605) -> (w604:u16[])
            }
            frame "Idle_2" {
              w609 = u16 0 ("t")
              # "To ensure timing, we split the\nidle state into 4 phases"
              # "Ncycles"
              # "Ncycles"
              # "RewCalib"
              # "RewCalib"
              # "Solenoid R"
              # "Solenoid L"
              n446 = call "myRIO_BRig_RT_dataMTrig_Solenoid_RewCalib_OnOff__L.vi"() -> ("output_Solenoid_RewCalib_OnOff__L"=w639:i32)  [unwired: 11 in]
              n447 = call "myRIO_BRig_RT_dataMTrig_Solenoid_N__L.vi"() -> ("output_Solenoid_N__L"=w627:i32)  [unwired: 11 in]
              n448 = call "myRIO_BRig_RT_dataMTrig_Solenoid_RewCalib_OnOff__R.vi"() -> ("output_Solenoid_RewCalib_OnOff__R"=w624:i32)  [unwired: 11 in]
              n449 = call "myRIO_BRig_RT_dataMTrig_Solenoid_N__R.vi"() -> ("output_Solenoid_N__R"=w623:i32)  [unwired: 11 in]
              n450 = Index Array(array=w630, index #1=w639, index #2=w627, index #3=w624, index #4=w623) -> (element #1=w626:u16, element #2=w621:u16, element #3=w622:u16, element #4=w620:u16)
              n451 = local read "RewCalib_Trig_L"() -> (w619:bool)
              n452 = local read "RewCalib_Trig_R"() -> (w618:bool)
              n453 = Equal To 0?(x=w621) -> (x = 0?=w629:bool)
              n454 = Equal To 0?(x=w620) -> (x = 0?=w628:bool)
              n455 = Not Equal To 0?(x=w622) -> (x != 0?=w640:bool)
              n456 = Not Equal To 0?(x=w626) -> (x != 0?=w641:bool)
              n457 = And(x=w629, y=w628) -> (x .and. y?=w633:bool)
              n458 = Or(x=w619, y=w618) -> (x .or. y?=w634:bool)
              n459 = Not Exclusive Or(1:w641, 2:w619) -> (0:w636:bool)
              n460 = Not Exclusive Or(1:w640, 2:w618) -> (0:w638:bool)
              n461 = And(x=w634, y=w633) -> (x .and. y?=w616:bool)
              n462 = Not(x=w636) -> (.not. x?=w635:bool)
              n463 = Not(x=w638) -> (.not. x?=w637:bool)
              n464 = Or(x=w635, y=w637) -> (x .or. y?=w617:bool)
              n465 = Or(x=w616, y=w617) -> (x .or. y?=w632:bool)
              n466 = local read "count_warmup_R"() -> (w608:u16)
              n467 = local read "count_warmup_L"() -> (w613:u16)
              n468 = Select(t=myRIO_BRig_RT__Case_NonExp_stateList."RewardCalibration_pre" ("Enum"), s=w632, f=myRIO_BRig_RT__Case_NonExp_stateList."Idle_3" ("Enum")) -> (s? t:f=w615:T1)
              n469 = Select(t=w609, s="count_warmup_L_reset", f=w613) -> (s? t:f=→"count_warmup_L":u16)
              n470 = Select(t=w609, s="count_warmup_R_reset", f=w608) -> (s? t:f=→"count_warmup_R":u16)
            }
            frame "Idle_3" {
              n471 = local read "MTrig_Laser_Switch"() -> (w656:bool)
              n472 = case shown="False" w656 {
                tunnel: "LR_reward_Event" -> [w668 w672]
                tunnel: "LR_wrong_Event" -> [w667 w671]
                tunnel: "LR_reward_Laser" -> [w666 w670]
                tunnel: "LR_wrong_Laser" -> [w665 w669]
                tunnel: [w668 _] -> w651
                tunnel: [w667 _] -> w650
                tunnel: [w666 _] -> w649
                tunnel: [w665 _] -> w648
                tunnel: [_ w672] -> w647
                tunnel: [_ w671] -> w646
                tunnel: [_ w670] -> w645
                tunnel: [_ w669] -> w644
                frame False {
                }
                frame True {
                }
              }
              n473 = xnode "Read/Write Control"("FPGA VI Reference In"=w664, "error in"=w663, "Left(F)_or_Right(T)"="Left(F)_or_Right(T)", "SelectionState"="SelectionState", "ignoreWrong"="ignoreWrong", "LR_reward_Event_l1"=w651, "LR_wrong_Event_l1"=w650, "LR_reward_Laser_l1"=w649, "LR_wrong_Laser_l1"=w648, "LR_reward_Event_l2"=w647, "LR_wrong_Event_l2"=w646, "LR_reward_Laser_l2"=w645, "LR_wrong_laser_l2"=w644) -> ("error out"=→"error out 6":errorcluster, "SelectReward"=→"SelectReward":bool, "SelectWrong"=→"SelectWrong":bool)  [unwired: 1 out]
            }
            frame "Idle_4" {
              n474 = local read "Laser_Tshutter_l1"() -> (w692:dbl)
              n475 = local read "Laser_duration_l1"() -> (w691:u16)
              n476 = local read "Laser_Tshutter_l2"() -> (w688:dbl)
              n477 = local read "Laser_duration_l2"() -> (w687:u16)
              n478 = local read "CueLed_duration"() -> (w683:u16)
              n479 = local read "Laser_Tpeak_l1"() -> (w694:dbl)
              n480 = local read "Laser_Tpeak_l2"() -> (w690:dbl)
              n481 = local read "CueLed_Tpeak"() -> (w685:dbl)
              n482 = local read "Laser_Freq_l1"() -> (w693:dbl)
              n483 = local read "Laser_Freq_l2"() -> (w689:dbl)
              n484 = local read "CueLed_Freq"() -> (w684:dbl)
              n485 = local read "FPGA_count2ms"() -> (w686:dbl)
              n486 = To Unsigned Word Integer(number=w686) -> (unsigned 16bit integer=w695:u16)
              n487 = call "myRIO_BRig_RT__calc_laser_FPGA_N.vi"("input_FPGA_count2ms"=w686, "input_Tpeak"=w694, "input_Freq"=w693, "input_Tshutter"=w692, "input_duration"=w691) -> ("output_laser_Npeak"=w682:u32, "output_laser_Nvalley"=w680:u32, "output_laser_Nshutter"=w678:u32, "output_laser_Nduration"=w676:u32)  [unwired: 6 in, 1 out]
              n488 = call "myRIO_BRig_RT__calc_laser_FPGA_N.vi"("input_FPGA_count2ms"=w686, "input_Tpeak"=w690, "input_Freq"=w689, "input_Tshutter"=w688, "input_duration"=w687) -> ("output_laser_Npeak"=w681:u32, "output_laser_Nvalley"=w679:u32, "output_laser_Nshutter"=w677:u32, "output_laser_Nduration"=w675:u32)  [unwired: 6 in, 1 out]
              n489 = call "myRIO_BRig_RT__calc_laser_FPGA_N__CueLed.vi"("input_FPGA_count2ms"=w686, "input_Tpeak"=w685, "input_Freq"=w684, "input_duration"=w683) -> ("output_laser_Npeak"=w674:u32, "output_laser_Nvalley"=w673:u32)  [unwired: 9 in, 1 out]
              n490 = xnode "Read/Write Control"("FPGA VI Reference In"=w700, "error in"=w699, "k1__counter_per_ms"=w695, "LC_nPeak_l1"=w682, "LC_nPeak_l2"=w681, "LC_nValley_l1"=w680, "LC_nValley_l2"=w679, "LC_nShutter_l1"=w678, "LC_nShutter_l2"=w677, "LR_reward_nTotal_l1"=w676, "LR_wrong_nTotal_l1"=w676, "LR_reward_nTotal_l2"=w675, "LR_wrong_nTotal_l2"=w675, "CueLed_nPeak"=w674, "CueLed_nValley"=w673) -> ("error out"=w696:errorcluster)  [unwired: 1 out]
              n491 = local write "error out"(w696) -> ()
            }
            frame "Idle_5" {
              w722 = u8 0 ("f")
              # "To ensure timing, we split the\nidle state into 4 phases"
              n492 = local read "MTrig_Solenoid_trig__L"() -> (w713:bool)
              n493 = local read "MTrig_Solenoid_trig__R"() -> (w723:bool)
              n494 = local read "warmupType"() -> (w706:u8)
              n495 = local read "warmup"() -> (w715:bool)
              n496 = Not Equal To 0?(x=w706) -> (x != 0?=w705:bool)
              n497 = Not(x=w705) -> (.not. x?=w716:bool)
              n498 = Select(t=u8 1, s=w713, f=w722) -> (s? t:f=w721:u8)
              n499 = Select(t=u8 2, s=w723, f=w722) -> (s? t:f=w720:u8)
              n500 = And(x=w715, y=w716) -> (x .and. y?=w714:bool)
              n501 = And(x=w715, y=w705) -> (x .and. y?=w709:bool)
              n502 = Add(x=w721, y=w720) -> (x+y=w719:u8)
              n503 = case shown="3" w719 {
                tunnel: w718 -> [w726 w730 w748 w766]
                tunnel: [w726 w729 w747 w765] -> w717
                tunnel: w714 -> [_ w728 w746 w764]
                tunnel: [_ TRUE TRUE TRUE] -> w711
                frame 0, Default {
                }
                frame 1 {
                  n504 = case shown="True" w728 {
                    tunnel: w730 -> [w739 w744]
                    tunnel: [w738 w743] -> w729
                    frame True {
                      # "Audio_L"
                      # "Solenoid_L"
                      n505 = call "myRIO_BRig_RT_dataMTrig_Solenoid_N__L.vi"() -> ("output_Solenoid_N__L"=w735:i32)  [unwired: 11 in]
                      n506 = call "myRIO_BRig_RT_dataMTrig_Audio_N__L.vi"() -> ("output_Audio_N__L"=w733:i32)  [unwired: 11 in]
                      n507 = Index Array(array=w739, index #1=w735, index #2=w733) -> (element #1=w737:u16, element #2=w736:u16)
                      n508 = Increment(x=w737) -> (x+1=w734:u16)
                      n509 = Increment(x=w736) -> (x+1=w732:u16)
                      n510 = Replace Array Subset(array=w739, new element #1=w734, index #1=w735, new element #2=w732, index #2=w733) -> (w738:u16[])
                    }
                    frame False {
                      # "Solenoid_L"
                      n511 = call "myRIO_BRig_RT_dataMTrig_Solenoid_N__L.vi"() -> ("output_Solenoid_N__L"=w741:i32)  [unwired: 11 in]
                      n512 = Index Array(array=w744, index=w741) -> (element=w742:u16)
                      n513 = Increment(x=w742) -> (x+1=w740:u16)
                      n514 = Replace Array Subset(array=w744, new element=w740, index=w741) -> (w743:u16[])
                    }
                  }
                  n515 = local write "MTrig_Solenoid_trig__L"(FALSE) -> ()
                }
                frame 2 {
                  n516 = case shown="True" w746 {
                    tunnel: w748 -> [w757 w762]
                    tunnel: [w756 w761] -> w747
                    frame True {
                      # "Audio_R"
                      # "Solenoid_R"
                      n517 = call "myRIO_BRig_RT_dataMTrig_Solenoid_N__R.vi"() -> ("output_Solenoid_N__R"=w753:i32)  [unwired: 11 in]
                      n518 = call "myRIO_BRig_RT_dataMTrig_Audio_N__R.vi"() -> ("output_Audio_N__R"=w752:i32)  [unwired: 11 in]
                      n519 = Index Array(array=w757, index #1=w753, index #2=w752) -> (element #1=w755:u16, element #2=w754:u16)
                      n520 = Increment(x=w754) -> (x+1=w750:u16)
                      n521 = Increment(x=w755) -> (x+1=w751:u16)
                      n522 = Replace Array Subset(array=w757, new element #1=w751, index #1=w753, new element #2=w750, index #2=w752) -> (w756:u16[])
                    }
                    frame False {
                      # "Solenoid_R"
                      n523 = call "myRIO_BRig_RT_dataMTrig_Solenoid_N__R.vi"() -> ("output_Solenoid_N__R"=w758:i32)  [unwired: 11 in]
                      n524 = Index Array(array=w762, index=w758) -> (element=w760:u16)
                      n525 = Increment(x=w760) -> (x+1=w759:u16)
                      n526 = Replace Array Subset(array=w762, new element=w759, index=w758) -> (w761:u16[])
                    }
                  }
                  n527 = local write "MTrig_Solenoid_trig__R"(FALSE) -> ()
                }
                frame 3 {
                  w767 = FALSE
                  n528 = case shown="True" w764 {
                    tunnel: w766 -> [w781 w789]
                    tunnel: [w780 w788] -> w765
                    frame True {
                      # "Audio_R"
                      # "Solenoid_R"
                      # "Audio_L"
                      # "Solenoid_L"
                      n529 = call "myRIO_BRig_RT_dataMTrig_Solenoid_N__L.vi"() -> ("output_Solenoid_N__L"=w775:i32)  [unwired: 11 in]
                      n530 = call "myRIO_BRig_RT_dataMTrig_Audio_N__L.vi"() -> ("output_Audio_N__L"=w773:i32)  [unwired: 11 in]
                      n531 = call "myRIO_BRig_RT_dataMTrig_Solenoid_N__R.vi"() -> ("output_Solenoid_N__R"=w771:i32)  [unwired: 11 in]
                      n532 = call "myRIO_BRig_RT_dataMTrig_Audio_N__R.vi"() -> ("output_Audio_N__R"=w770:i32)  [unwired: 11 in]
                      n533 = Index Array(array=w781, index #1=w775, index #2=w773, index #3=w771, index #4=w770) -> (element #1=w779:u16, element #2=w778:u16, element #3=w777:u16, element #4=w776:u16)
                      n534 = Increment(x=w776) -> (x+1=w768:u16)
                      n535 = Increment(x=w779) -> (x+1=w774:u16)
                      n536 = Increment(x=w778) -> (x+1=w772:u16)
                      n537 = Increment(x=w777) -> (x+1=w769:u16)
                      n538 = Replace Array Subset(array=w781, new element #1=w774, index #1=w775, new element #2=w772, index #2=w773, new element #3=w769, index #3=w771, new element #4=w768, index #4=w770) -> (w780:u16[])
                    }
                    frame False {
                      # "Solenoid_R"
                      # "Solenoid_L"
                      n539 = call "myRIO_BRig_RT_dataMTrig_Solenoid_N__L.vi"() -> ("output_Solenoid_N__L"=w785:i32)  [unwired: 11 in]
                      n540 = call "myRIO_BRig_RT_dataMTrig_Solenoid_N__R.vi"() -> ("output_Solenoid_N__R"=w782:i32)  [unwired: 11 in]
                      n541 = Index Array(array=w789, index #1=w785, index #2=w782) -> (element #1=w787:u16, element #2=w786:u16)
                      n542 = Increment(x=w787) -> (x+1=w784:u16)
                      n543 = Increment(x=w786) -> (x+1=w783:u16)
                      n544 = Replace Array Subset(array=w789, new element #1=w784, index #1=w785, new element #2=w783, index #2=w782) -> (w788:u16[])
                    }
                  }
                  n545 = local write "MTrig_Solenoid_trig__L"(w767) -> ()
                  n546 = local write "MTrig_Solenoid_trig__R"(w767) -> ()
                }
              }
              n547 = local read "get_countPerMS"() -> (w704:bool)
              n548 = Select(t=myRIO_BRig_RT__Case_NonExp_stateList."Get_FPGA_count_per_ms" ("Enum"), s=w704, f=myRIO_BRig_RT__Case_NonExp_stateList."Idle_6" ("Enum")) -> (s? t:f=w702:T1)
              n549 = Select(t=myRIO_BRig_RT__Case_NonExp_stateList."Cue_pre", s=w709, f=myRIO_BRig_RT__Case_NonExp_stateList."DispenseWater_pre" ("Enum")) -> (s? t:f=w707:T1)
              n550 = Select(t=w707, s=w711, f=w702) -> (s? t:f=w712:T1)
            }
            frame "Idle_6" {
              # "use dataMTrig as it is one of the last to transfer"
              # "To ensure timing, we split the\nidle state into 4 phases"
              n551 = call "myRIO_BRig_RT_comm_webdav_uploadReceived_check_v2,0.vi"("input_dataName"="dataMTrig") -> ("output_Iexist"=w794:bool)  [unwired: 9 in, 1 out]
              n552 = Select(t=myRIO_BRig_RT__Case_NonExp_stateList."UploadSettings_pre" ("Enum"), s=w794, f=myRIO_BRig_RT__Case_NonExp_stateList."Idle") -> (s? t:f=w792:T1)
            }
            frame "Cue_pre" {
              w813 = u16 1 ("t")
              w812 = u16 0 ("new element/subarray")
              w809 = u16 0 ("new element/subarray")
              # "Ncycle"
              # "count"
              # "Audio_R"
              # "Solenoid_R"
              # "Solenoid_L"
              # "Ncycle"
              # "count"
              # "Audio_L"
              n553 = local read "Cue1Param_CueType_Switch"() -> (w807:u16)
              n554 = case shown="2" w807 {
                tunnel: [TRUE _ w824] -> w804
                frame 0, Default {
                }
                frame 1 {
                }
                frame 2 {
                  n555 = Random Number (0-1)() -> (number: 0 to 1=w830:dbl)
                  n556 = local read "Cue1Param_AudioLed_Probability_Switch"() -> (w825:u16)
                  n557 = Multiply(x=w830, y=100.0) -> (x*y=w829:dbl)
                  n558 = Round To Nearest(number=w829) -> (nearest integer value=w828:dbl)
                  n559 = To Unsigned Word Integer(number=w828) -> (unsigned 16bit integer=w826:u16)
                  n560 = Less?(x=w825, y=w826) -> (x < y?=w824:bool)
                }
              }
              n561 = call "myRIO_BRig_RT_dataMTrig_Solenoid_N__L.vi"() -> ("output_Solenoid_N__L"=w822:i32)  [unwired: 11 in]
              n562 = call "myRIO_BRig_RT_dataMTrig_Solenoid_N__R.vi"() -> ("output_Solenoid_N__R"=w821:i32)  [unwired: 11 in]
              n563 = Index Array(array=w818, index #1=w822, index #2=w821) -> (element #1=w820:u16, element #2=w819:u16)
              n564 = Not Equal To 0?(x=w819) -> (x != 0?=w799:bool)
              n565 = Not Equal To 0?(x=w820) -> (x != 0?=w800:bool)
              n566 = And(x=w804, y=w800) -> (x .and. y?=w805:bool)
              n567 = And(x=w804, y=w799) -> (x .and. y?=w806:bool)
              n568 = Select(t=w813, s=w805, f=w812) -> (s? t:f=w814:u16)
              n569 = Select(t=w813, s=w806, f=w812) -> (s? t:f=w808:u16)
              n570 = Select(t=myRIO_BRig_RT__Case_NonExp_stateList."Cue", s=w804, f=myRIO_BRig_RT__Case_NonExp_stateList."Cue_LED") -> (s? t:f=w802:T1)
              n571 = call "myRIO_BRig_RT_dataMTrig_Audio_c__L.vi"() -> ("output_Audio_c__L"=w816:i32)  [unwired: 11 in]
              n572 = call "myRIO_BRig_RT_dataMTrig_Audio_N__L.vi"() -> ("output_Audio_N__L"=w815:i32)  [unwired: 11 in]
              n573 = call "myRIO_BRig_RT_dataMTrig_Audio_c__R.vi"() -> ("output_Audio_c__R"=w811:i32)  [unwired: 11 in]
              n574 = call "myRIO_BRig_RT_dataMTrig_Audio_N__R.vi"() -> ("output_Audio_N__R"=w810:i32)  [unwired: 11 in]
              n575 = Initialize Array(u16 0 ("element"), 1 ("dimension size")) -> (w798:u16[])
              n576 = Replace Array Subset(array=w818, new element #1=w809, index #1=w816, new element #2=w814, index #2=w815, new element #3=w809, index #3=w811, new element #4=w808, index #4=w810) -> (w817:u16[])
            }
            frame "Cue" {
              # "lick did not occur or warmupType==1"
              # "lick occurred?"
              # "Ncycle"
              # "Audio_R"
              # "Ncycle"
              # "Audio_L"
              n577 = local read "warmupType"() -> (w839:u8)
              n578 = Greater?(x=w845, y=w844) -> (0:w848:bool)
              n579 = Greater?(x=w847, y=w846) -> (0:w843:bool)
              n580 = Or(x=w843, y=w848) -> (x .or. y?=w837:bool)
              n581 = Equal?(x=w839, y=u8 1) -> (x = y?=w833:bool)
              n582 = Not(x=w837) -> (.not. x?=w836:bool)
              n583 = call "myRIO_BRig_RT_dataMTrig_Audio_N__L.vi"() -> ("output_Audio_N__L"=w850:i32)  [unwired: 11 in]
              n584 = call "myRIO_BRig_RT_dataMTrig_Audio_N__R.vi"() -> ("output_Audio_N__R"=w849:i32)  [unwired: 11 in]
              n585 = Or(x=w836, y=w833) -> (x .or. y?=w834:bool)
              n586 = case shown="True" w834 {
                tunnel: w850 -> [w856 w874]
                tunnel: w849 -> [w855 w873]
                tunnel: w842 -> [w858 w868]
                tunnel: [w857 w868] -> w841
                tunnel: w840 -> [_ w866]
                tunnel: [myRIO_BRig_RT__Case_NonExp_stateList."Idle" ("t") w865] -> w835
                tunnel: w833 -> [_ w864]
                tunnel: w832 -> [_ w860]
                tunnel: w831 -> [_ w859]
                frame False {
                  w851 = u16 0 ("new element/subarray")
                  # "lick occurred and warmupType==2"
                  n587 = call "myRIO_BRig_RT_dataMTrig_Solenoid_N__R.vi"() -> ("output_Solenoid_N__R"=w852:i32)  [unwired: 11 in]
                  n588 = call "myRIO_BRig_RT_dataMTrig_Solenoid_N__L.vi"() -> ("output_Solenoid_N__L"=w853:i32)  [unwired: 11 in]
                  n589 = Replace Array Subset(array=w858, new element #1=w851, index #1=w856, new element #2=w851, index #2=w855, new element #3=w851, index #3=w853, new element #4=w851, index #4=w852) -> (w857:u16[])
                }
                frame True {
                  n590 = Not(x=w864) -> (.not. x?=w863:bool)
                  n591 = Index Array(array=w868, index #1=w874, index #2=w873) -> (element #1=w872:u16, element #2=w871:u16)
                  n592 = Equal To 0?(x=w872) -> (x = 0?=w870:bool)
                  n593 = Equal To 0?(x=w871) -> (x = 0?=w869:bool)
                  n594 = And(x=w870, y=w869) -> (x .and. y?=w862:bool)
                  n595 = And(x=w862, y=w863) -> (x .and. y?=w861:bool)
                  n596 = case shown="True" w861 {
                    tunnel: w860 -> [_ w882]
                    tunnel: w859 -> [_ w877]
                    frame False {
                    }
                    frame True {
                      n597 = local read "count_warmup_R"() -> (w875:u16)
                      n598 = local read "count_warmup_L"() -> (w880:u16)
                      n599 = Increment(x=w875) -> (x+1=w878:u16)
                      n600 = Increment(x=w880) -> (x+1=w881:u16)
                      n601 = Select(t=w878, s=w877, f=w875) -> (s? t:f=w876:u16)
                      n602 = Select(t=w881, s=w882, f=w880) -> (s? t:f=w879:u16)
                      n603 = local write "count_warmup_R"(w876) -> ()
                      n604 = local write "count_warmup_L"(w879) -> ()
                    }
                  }
                  n605 = Select(t=myRIO_BRig_RT__Case_NonExp_stateList."DispenseWater_pre", s=w862, f=w866) -> (s? t:f=w865:T1)
                }
              }
            }
            frame "Cue_LED" {
              # "lick did not occur or warmupType==1"
              # "lick occurred?"
              n606 = local read "warmupType"() -> (w895:u8)
              n607 = Greater?(x=w901, y=w900) -> (0:w904:bool)
              n608 = Greater?(x=w903, y=w902) -> (0:w899:bool)
              n609 = Or(x=w899, y=w904) -> (x .or. y?=w893:bool)
              n610 = Equal?(x=w895, y=u8 1) -> (x = y?=w889:bool)
              n611 = Not(x=w893) -> (.not. x?=w892:bool)
              n612 = Or(x=w892, y=w889) -> (x .or. y?=w890:bool)
              n613 = case shown="True" w890 {
                tunnel: w898 -> [w911 w931]
                tunnel: [w910 w931] -> w897
                tunnel: w896 -> [_ w917]
                tunnel: [myRIO_BRig_RT__Case_NonExp_stateList."Idle" ("t") w930] -> w891
                tunnel: w889 -> [_ w916]
                tunnel: w888 -> [_ w928]
                tunnel: w887 -> [_ w927]
                tunnel: w886 -> [w905 w926]
                tunnel: [w905 w919] -> w885
                tunnel: w884 -> [_ w914]
                tunnel: w883 -> [_ w913]
                frame False {
                  w906 = u16 0 ("new element/subarray")
                  # "lick occurred and warmupType==2"
                  n614 = call "myRIO_BRig_RT_dataMTrig_Solenoid_N__R.vi"() -> ("output_Solenoid_N__R"=w907:i32)  [unwired: 11 in]
                  n615 = call "myRIO_BRig_RT_dataMTrig_Solenoid_N__L.vi"() -> ("output_Solenoid_N__L"=w908:i32)  [unwired: 11 in]
                  n616 = Replace Array Subset(array=w911, new element #1=w906, new element #2=w906, index #2=w908, new element #3=w906, index #3=w907) -> (w910:u16[])  [unwired: 1 in]
                }
                frame True {
                  w924 = 0 ("index")
                  n617 = local read "CueLed_duration"() -> (w920:u16)
                  n618 = Index Array(array=w926, index=w924) -> (element=w925:u16)
                  n619 = Increment(x=w925) -> (x+1=w923:u16)
                  n620 = Multiply(x=w923, y=u16 5) -> (x*y=w921:u16)
                  n621 = Replace Array Subset(array=w926, new element=w923, index=w924) -> (w919:u16[])
                  n622 = Less?(x=w921, y=w920) -> (x < y?=w915:bool)
                  n623 = Not Or(1:w916, 2:w915) -> (0:w929:bool)
                  n624 = case shown="True" w929 {
                    tunnel: w928 -> [_ w939]
                    tunnel: w927 -> [_ w934]
                    frame False {
                    }
                    frame True {
                      n625 = local read "count_warmup_R"() -> (w932:u16)
                      n626 = local read "count_warmup_L"() -> (w937:u16)
                      n627 = Increment(x=w932) -> (x+1=w935:u16)
                      n628 = Increment(x=w937) -> (x+1=w938:u16)
                      n629 = Select(t=w935, s=w934, f=w932) -> (s? t:f=w933:u16)
                      n630 = Select(t=w938, s=w939, f=w937) -> (s? t:f=w936:u16)
                      n631 = local write "count_warmup_R"(w933) -> ()
                      n632 = local write "count_warmup_L"(w936) -> ()
                    }
                  }
                  n633 = Select(t=w917, s=w915, f=myRIO_BRig_RT__Case_NonExp_stateList."DispenseWater_pre" ("t")) -> (s? t:f=w930:T1)
                  n634 = xnode "Read/Write Control"("FPGA VI Reference In"=w914, "error in"=w913, "CueLed_Event"=w915) -> ("error out"=w912:errorcluster)  [unwired: 1 out]
                  n635 = local write "error out"(w912) -> ()
                }
              }
            }
            frame "RewardCalibration_pre" {
              (unwired) FALSE
              w940 = FALSE
              w951 = u8 0
              w967 = u8 0
              # "Are we starting a RewardCalibration?\nOr are we stopping a RewardCalibration?\nOr is a RewardCalibration over?"
              # "RewCalib\nOnOff"
              # "N"
              # "Solenoid R"
              # "RewCalib\nOnOff"
              # "N"
              # "Solenoid L"
              n636 = local read "RewCalib_Trig_L"() -> (w974:bool)
              n637 = local read "RewCalib_Trig_R"() -> (w943:bool)
              n638 = call "myRIO_BRig_RT_dataMTrig_Solenoid_N__R.vi"() -> ("output_Solenoid_N__R"=w945:i32)  [unwired: 11 in]
              n639 = call "myRIO_BRig_RT_dataMTrig_Solenoid_RewCalib_OnOff__R.vi"() -> ("output_Solenoid_RewCalib_OnOff__R"=w942:i32)  [unwired: 11 in]
              n640 = call "myRIO_BRig_RT_dataMTrig_Solenoid_N__L.vi"() -> ("output_Solenoid_N__L"=w960:i32)  [unwired: 11 in]
              n641 = call "myRIO_BRig_RT_dataMTrig_Solenoid_RewCalib_OnOff__L.vi"() -> ("output_Solenoid_RewCalib_OnOff__L"=w961:i32)  [unwired: 11 in]
              n642 = Index Array(array=w944, index #1=w945, index #2=w942) -> (element #1=w955:u16, element #2=w950:u16)
              n643 = Index Array(array=w944, index #1=w960, index #2=w961) -> (element #1=w971:u16, element #2=w966:u16)
              n644 = Equal To 0?(x=w955) -> (x = 0?=w956:bool)
              n645 = Not Equal To 0?(x=w950) -> (x != 0?=w953:bool)
              n646 = Equal To 0?(x=w971) -> (x = 0?=w972:bool)
              n647 = Not Equal To 0?(x=w966) -> (x != 0?=w969:bool)
              n648 = local write "MTrig_Solenoid_trig__L"(w940) -> ()
              n649 = local write "MTrig_Solenoid_trig__R"(w940) -> ()
              n650 = Select(t=u8 1, s=w943, f=w951) -> (s? t:f=w947:u8)
              n651 = Select(t=u8 1, s=w974, f=w967) -> (s? t:f=w963:u8)
              n652 = Select(t=u8 2, s=w956, f=w951) -> (s? t:f=w948:u8)
              n653 = Select(t=u8 4, s=w953, f=w951) -> (s? t:f=w949:u8)
              n654 = Select(t=u8 2, s=w972, f=w967) -> (s? t:f=w964:u8)
              n655 = Select(t=u8 4, s=w969, f=w967) -> (s? t:f=w965:u8)
              n656 = Compound Arithmetic op=ADD(w947, w948, w949) -> (w946:u8)
              n657 = Compound Arithmetic op=ADD(w963, w964, w965) -> (w962:u8)
              n658 = case shown="7" w962 {
                tunnel: w944 -> [w1004 w1009 w1011 w1016 w1021 w1023 w1026 w1031]
                tunnel: [w1004 w1010 w1011 w1017 w1022 w1023 w1027 w1032] -> w959
                tunnel: w961 -> [_ w1007 _ w1014 w1019 _ w1025 w1030]
                tunnel: w960 -> [_ w1008 _ w1015 w1020 _ _ _]
                frame 0, Default {
                }
                frame 1 {
                  n659 = Replace Array Subset(array=w1009, new element #1=u16 100 ("new element/subarray"), index #1=w1008, new element #2=u16 1 ("new element/subarray"), index #2=w1007) -> (w1010:u16[])
                }
                frame 2 {
                }
                frame 3 {
                  n660 = Replace Array Subset(array=w1016, new element #1=u16 100 ("new element/subarray"), index #1=w1015, new element #2=u16 1 ("new element/subarray"), index #2=w1014) -> (w1017:u16[])
                }
                frame 4 {
                  w1018 = u16 0 ("new element/subarray")
                  n661 = Replace Array Subset(array=w1021, new element #1=w1018, index #1=w1020, new element #2=w1018, index #2=w1019) -> (w1022:u16[])
                }
                frame 5 {
                }
                frame 6 {
                  n662 = Replace Array Subset(array=w1026, new element=u16 0 ("new element/subarray"), index=w1025) -> (w1027:u16[])
                }
                frame 7 {
                  n663 = local write "RewCalib_Trig_L"(FALSE ("RewCalib_Trig_L")) -> ()
                  n664 = Replace Array Subset(array=w1031, new element=u16 0 ("new element/subarray"), index=w1030) -> (w1032:u16[])
                }
              }
              n665 = case shown="7" w946 {
                tunnel: w959 -> [w975 w980 w982 w987 w992 w994 w997 w1002]
                tunnel: [w975 w981 w982 w988 w993 w994 w998 w1003] -> w958
                tunnel: w942 -> [_ w978 _ w985 w990 _ w996 w1001]
                tunnel: w945 -> [_ w979 _ w986 w991 _ _ _]
                frame 0, Default {
                }
                frame 1 {
                  n666 = Replace Array Subset(array=w980, new element #1=u16 100 ("new element/subarray"), index #1=w979, new element #2=u16 1 ("new element/subarray"), index #2=w978) -> (w981:u16[])
                }
                frame 2 {
                }
                frame 3 {
                  n667 = Replace Array Subset(array=w987, new element #1=u16 100 ("new element/subarray"), index #1=w986, new element #2=u16 1 ("new element/subarray"), index #2=w985) -> (w988:u16[])
                }
                frame 4 {
                  w989 = u16 0 ("new element/subarray")
                  n668 = Replace Array Subset(array=w992, new element #1=w989, index #1=w991, new element #2=w989, index #2=w990) -> (w993:u16[])
                }
                frame 5 {
                }
                frame 6 {
                  n669 = Replace Array Subset(array=w997, new element=u16 0 ("new element/subarray"), index=w996) -> (w998:u16[])
                }
                frame 7 {
                  n670 = local write "RewCalib_Trig_R"(FALSE ("RewCalib_Trig_L")) -> ()
                  n671 = Replace Array Subset(array=w1002, new element=u16 0 ("new element/subarray"), index=w1001) -> (w1003:u16[])
                }
              }
            }
            frame "DispenseWater_pre" {
              w1038 = u16 0 ("t")
              w1081 = u16 0 ("new element/subarray")
              # "just trust me on this one"
              # "RewCalib\nOnOff"
              # "RewCalib\nOnOff"
              # "nCycle"
              # "Solenoid__R"
              # "Tdelay"
              # "delay"
              # "nCycle"
              # "Solenoid__L"
              # "Tdelay"
              # "delay"
              # "Solenoid__R"
              # "count"
              # "Solenoid_Tcycle_R"
              # "Solenoid_Tcycle_L"
              # "Solenoid__L"
              # "count"
              n672 = call "myRIO_BRig_RT_dataMTrig_Solenoid_RewCalib_OnOff__L.vi"() -> ("output_Solenoid_RewCalib_OnOff__L"=w1045:i32)  [unwired: 11 in]
              n673 = call "myRIO_BRig_RT_dataMTrig_Solenoid_N__L.vi"() -> ("output_Solenoid_N__L"=w1036:i32)  [unwired: 11 in]
              n674 = call "myRIO_BRig_RT_dataMTrig_Solenoid_delay__L.vi"() -> ("output_Solenoid_delay__L"=w1079:i32)  [unwired: 11 in]
              n675 = call "myRIO_BRig_RT_dataMTrig_Solenoid_Tdelay__L.vi"() -> ("output_Solenoid_Tdelay__L"=w1078:i32)  [unwired: 11 in]
              n676 = call "myRIO_BRig_RT_dataMTrig_Solenoid_N__R.vi"() -> ("output_Solenoid_N__R"=w1034:i32)  [unwired: 11 in]
              n677 = call "myRIO_BRig_RT_dataMTrig_Solenoid_delay__R.vi"() -> ("output_Solenoid_delay__R"=w1068:i32)  [unwired: 11 in]
              n678 = call "myRIO_BRig_RT_dataMTrig_Solenoid_Tdelay__R.vi"() -> ("output_Solenoid_Tdelay__R"=w1067:i32)  [unwired: 11 in]
              n679 = call "myRIO_BRig_RT_dataMTrig_Solenoid_RewCalib_OnOff__R.vi"() -> ("output_Solenoid_RewCalib_OnOff__R"=w1041:i32)  [unwired: 11 in]
              n680 = Index Array(array=w1080, index #1=w1036, index #2=w1079, index #3=w1078, index #4=w1034, index #5=w1068, index #6=w1067, index #7=w1045, index #8=w1041) -> (element #1=w1037:u16, element #2=w1077:u16, element #3=w1072:u16, element #4=w1040:u16, element #5=w1062:u16, element #6=w1061:u16, element #7=w1046:u16, element #8=w1043:u16)
              n681 = Equal To 0?(x=w1077) -> (x = 0?=w1076:bool)
              n682 = Equal To 0?(x=w1062) -> (x = 0?=w1066:bool)
              n683 = local read "RewCalib_Trig_L"() -> (w1057:bool)
              n684 = local read "RewCalib_Trig_R"() -> (w1052:bool)
              n685 = Not Equal To 0?(x=w1037) -> (x != 0?=w1075:bool)
              n686 = Not Equal To 0?(x=w1040) -> (x != 0?=w1065:bool)
              n687 = local read "MTrig_Solenoid_Tcycle__L"() -> (w1074:u16)
              n688 = local read "MTrig_Solenoid_Tcycle__R"() -> (w1060:u16)
              n689 = Not Equal To 0?(x=w1046) -> (x != 0?=w1056:bool)
              n690 = Not Equal To 0?(x=w1043) -> (x != 0?=w1054:bool)
              n691 = Not(x=w1057) -> (.not. x?=w1055:bool)
              n692 = Not(x=w1052) -> (.not. x?=w1053:bool)
              n693 = And(x=w1056, y=w1055) -> (x .and. y?=w1051:bool)
              n694 = And(x=w1054, y=w1053) -> (x .and. y?=w1050:bool)
              n695 = call "myRIO_BRig_RT_dataMTrig_Solenoid_c__L.vi"() -> ("output_Solenoid_c__L"=w1083:i32)  [unwired: 11 in]
              n696 = call "myRIO_BRig_RT_dataMTrig_Solenoid_c__R.vi"() -> ("output_Solenoid_c__R"=w1082:i32)  [unwired: 11 in]
              n697 = Select(t=w1074, s=w1075, f=u16 0) -> (s? t:f=w1071:u16)
              n698 = Or(x=w1051, y=w1050) -> (x .or. y?=w1039:bool)
              n699 = Select(t=w1060, s=w1065, f=u16 0) -> (s? t:f=w1063:u16)
              n700 = Select(t=w1071, s=w1076, f=w1072) -> (s? t:f=w1069:u16)
              n701 = Select(t=w1063, s=w1066, f=w1061) -> (s? t:f=w1058:u16)
              n702 = call "myRIO_BRig_RT_dataMTrig_Solenoid_Tcycle__L.vi"() -> ("output_Solenoid_Tcycle__L"=w1070:i32)  [unwired: 11 in]
              n703 = call "myRIO_BRig_RT_dataMTrig_Solenoid_Tcycle__R.vi"() -> ("output_Solenoid_Tcycle__R"=w1059:i32)  [unwired: 11 in]
              n704 = Select(t=w1038, s=w1039, f=w1037) -> (s? t:f=w1035:u16)
              n705 = Select(t=w1038, s=w1039, f=w1040) -> (s? t:f=w1033:u16)
              n706 = Select(t=myRIO_BRig_RT__Case_NonExp_stateList."Idle" ("Enum"), s=w1039, f=myRIO_BRig_RT__Case_NonExp_stateList."DispenseWater" ("Enum")) -> (s? t:f=w1047:T1)
              n707 = Select(t=w1038, s=w1039, f=w1046) -> (s? t:f=w1044:u16)
              n708 = Select(t=w1038, s=w1039, f=w1043) -> (s? t:f=w1042:u16)
              n709 = Replace Array Subset(array=w1080, new element #1=w1081, index #1=w1083, new element #2=w1081, index #2=w1082, new element #3=w1069, index #3=w1070, new element #4=w1058, index #4=w1059, new element #5=w1044, index #5=w1045, new element #6=w1042, index #6=w1041, new element #7=w1035, index #7=w1036, new element #8=w1033, index #8=w1034) -> (w1084:u16[])
            }
            frame "DispenseWater" {
              # "D"
              # "C"
              # "B"
              # "A"
              # "(A) Add COUNT and INCREMENT\n(B) Is (A) smaller than Tcycle?\n(C) Are we dispensing water or in the delay phase?\n(D) If (A) is smaller than Tcycle   AND   if we are dispensing water\n      then send TRUE to solenoid"
              # "delay"
              # "Tcycle"
              # "Solenoid__R"
              # "count"
              # "delay"
              # "Tcycle"
              # "Solenoid__L"
              # "count"
              n710 = To Unsigned Word Integer(number=w1111) -> (unsigned 16bit integer=w1093:u16)
              n711 = call "myRIO_BRig_RT_dataMTrig_Solenoid_delay__R.vi"() -> ("output_Solenoid_delay__R"=w1097:i32)  [unwired: 11 in]
              n712 = call "myRIO_BRig_RT_dataMTrig_Solenoid_c__R.vi"() -> ("output_Solenoid_c__R"=w1096:i32)  [unwired: 11 in]
              n713 = call "myRIO_BRig_RT_dataMTrig_Solenoid_Tcycle__R.vi"() -> ("output_Solenoid_Tcycle__R"=w1098:i32)  [unwired: 11 in]
              n714 = call "myRIO_BRig_RT_dataMTrig_Solenoid_delay__L.vi"() -> ("output_Solenoid_delay__L"=w1113:i32)  [unwired: 11 in]
              n715 = call "myRIO_BRig_RT_dataMTrig_Solenoid_c__L.vi"() -> ("output_Solenoid_c__L"=w1105:i32)  [unwired: 11 in]
              n716 = call "myRIO_BRig_RT_dataMTrig_Solenoid_Tcycle__L.vi"() -> ("output_Solenoid_Tcycle__L"=w1114:i32)  [unwired: 11 in]
              n717 = Index Array(array=w1107, index #1=w1105, index #2=w1114, index #3=w1113, index #4=w1096, index #5=w1098, index #6=w1097) -> (element #1=w1112:u16, element #2=w1102:u16, element #3=w1110:u16, element #4=w1092:u16, element #5=w1089:u16, element #6=w1088:u16)
              n718 = Add(x=w1112, y=w1093) -> (x+y=w1103:u16)
              n719 = Add(x=w1092, y=w1093) -> (x+y=w1094:u16)
              n720 = Less?(x=w1103, y=w1102) -> (x < y?=w1086:bool)
              n721 = Equal To 0?(x=w1110) -> (x = 0?=w1109:bool)
              n722 = Less?(x=w1094, y=w1089) -> (x < y?=w1087:bool)
              n723 = Equal To 0?(x=w1088) -> (x = 0?=w1095:bool)
              n724 = And(x=w1086, y=w1109) -> (x .and. y?=w1108:bool)
              n725 = Or(x=w1086, y=w1087) -> (x .or. y?=w1085:bool)
              n726 = And(x=w1087, y=w1095) -> (x .and. y?=w1090:bool)
              n727 = Select(t=w1103, s=w1086, f=w1102) -> (s? t:f=w1104:u16)
              n728 = Select(t=w1094, s=w1087, f=w1089) -> (s? t:f=w1091:u16)
              n729 = Replace Array Subset(array=w1107, new element #1=w1104, index #1=w1105, new element #2=w1091, index #2=w1096) -> (w1106:u16[])
              n730 = Select(t=w1101, s=w1085, f=myRIO_BRig_RT__Case_NonExp_stateList."DispenseWater_post" ("Enum")) -> (s? t:f=w1099:T1)
            }
            frame "DispenseWater_post" {
              # "nCycle"
              # "delay"
              # "Solenoid__R"
              # "nCycle"
              # "delay"
              # "Solenoid__L"
              n731 = call "myRIO_BRig_RT_dataMTrig_Solenoid_N__L.vi"() -> ("output_Solenoid_N__L"=w1131:i32)  [unwired: 11 in]
              n732 = call "myRIO_BRig_RT_dataMTrig_Solenoid_delay__L.vi"() -> ("output_Solenoid_delay__L"=w1130:i32)  [unwired: 11 in]
              n733 = call "myRIO_BRig_RT_dataMTrig_Solenoid_N__R.vi"() -> ("output_Solenoid_N__R"=w1127:i32)  [unwired: 11 in]
              n734 = call "myRIO_BRig_RT_dataMTrig_Solenoid_delay__R.vi"() -> ("output_Solenoid_delay__R"=w1126:i32)  [unwired: 11 in]
              n735 = Index Array(array=w1133, index #1=w1131, index #2=w1130, index #3=w1127, index #4=w1126) -> (element #1=w1135:u16, element #2=w1134:u16, element #3=w1118:u16, element #4=w1120:u16)
              n736 = Not Equal To 0?(x=w1135) -> (x != 0?=w1136:bool)
              n737 = Not Equal To 0?(x=w1118) -> (x != 0?=w1119:bool)
              n738 = case shown="True" w1119 {
                selector: w1119 -> [_ w1140]
                tunnel: w1118 -> [w1138 w1146]
                tunnel: w1120 -> [_ w1147]
                tunnel: [w1138 w1144] -> w1117
                tunnel: [u16 0 w1143] -> w1116
                tunnel: [_ w1140] -> w1115
                frame False {
                }
                frame True {
                  n739 = Equal To 0?(x=w1147) -> (x = 0?=w1139:bool)
                  n740 = Decrement(x=w1146) -> (x-1=w1145:u16)
                  n741 = Select(t=w1145, s=w1139, f=w1146) -> (s? t:f=w1144:u16)
                  n742 = Select(t=u16 1, s=w1139, f=u16 0) -> (s? t:f=w1143:u16)
                }
              }
              n743 = case shown="True" w1136 {
                selector: w1136 -> [_ w1151]
                tunnel: w1135 -> [w1149 w1157]
                tunnel: w1134 -> [_ w1158]
                tunnel: [w1149 w1155] -> w1129
                tunnel: [u16 0 w1154] -> w1128
                tunnel: [_ w1151] -> w1125
                frame False {
                }
                frame True {
                  n744 = Equal To 0?(x=w1158) -> (x = 0?=w1150:bool)
                  n745 = Decrement(x=w1157) -> (x-1=w1156:u16)
                  n746 = Select(t=w1156, s=w1150, f=w1157) -> (s? t:f=w1155:u16)
                  n747 = Select(t=u16 1, s=w1150, f=u16 0) -> (s? t:f=w1154:u16)
                }
              }
              n748 = Or(x=w1125, y=w1115) -> (x .or. y?=w1124:bool)
              n749 = Replace Array Subset(array=w1133, new element #1=w1129, index #1=w1131, new element #2=w1128, index #2=w1130, new element #3=w1117, index #3=w1127, new element #4=w1116, index #4=w1126) -> (w1132:u16[])
              n750 = Select(t=myRIO_BRig_RT__Case_NonExp_stateList."DispenseWater_pre" ("Enum"), s=w1124, f=myRIO_BRig_RT__Case_NonExp_stateList."Idle" ("Enum")) -> (s? t:f=w1121:T1)
            }
            frame "TestConnection" {
              n751 = local read "Host Password"() -> (w1164:string)
              n752 = local read "Host UserName"() -> (w1165:string)
              n753 = call "myRIO_BRig_RT_comm_webdav_testConnect.vi"("input_password"=w1164, "input_username"=w1165) -> ("output_Iconnected"=w1162:bool)  [unwired: 9 in]
              n754 = Select(t="Connection accepted!" ("message"), s=w1162, f="Error!") -> (s? t:f=w1160:string)
              n755 = One Button Dialog(message=w1160) -> ()  [unwired: 1 in, 1 out]
            }
            frame "SendData" {
              n756 = local read "Data Set Prefix"() -> (w1167:string)
              n757 = local read "Host Password"() -> (w1168:string)
              n758 = local read "Host UserName"() -> (w1169:string)
              n759 = call "myRIO_BRig_RT_comm_webdav_sendData_all.vi"("Host Filename Prefix"=w1167, "Host Password"=w1168, "Host UserName"=w1169) -> ()  [unwired: 9 in]
            }
            frame "Get_FPGA_count_per_ms" {
              n760 = case shown="False" w1182 {
                selector: w1182 -> [w1184 _]
                tunnel: w1180 -> [_ w1197]
                tunnel: [w1188 w1197] -> w1179
                tunnel: w1178 -> [w1187 w1195]
                tunnel: w1177 -> [w1186 w1194]
                tunnel: [w1185 w1192] -> w1176
                tunnel: [w1184 w1191] -> w1175
                frame False {
                  n761 = Get Date/Time In Seconds() -> (seconds since 1Jan1904=w1189:timestamp)
                  n762 = xnode "Read/Write Control"("FPGA VI Reference In"=w1187, "error in"=w1186, "timeTrial_trig"=TRUE ("timeTrial")) -> ("error out"=w1185:errorcluster)  [unwired: 1 out]
                  n763 = To Double Precision Float(number=w1189) -> (double precision float=w1188:dbl)
                  n764 = local write "get_countPerMS"(w1184) -> ()
                }
                frame True {
                  w1193 = 1.0
                  n765 = Get Date/Time In Seconds() -> (seconds since 1Jan1904=w1198:timestamp)
                  n766 = To Double Precision Float(number=w1198) -> (double precision float=w1199:dbl)
                  n767 = Subtract(x=w1199, y=w1197) -> (x-y=w1196:dbl)
                  n768 = Less Or Equal?(x=w1193, y=w1196) -> (x <= y?=w1191:bool)
                  n769 = case shown="True" w1191 {
                    tunnel: w1195 -> [_ w1212]
                    tunnel: w1194 -> [w1200 w1211]
                    tunnel: w1193 -> [_ w1202]
                    tunnel: [w1200 w1201] -> w1192
                    frame False {
                    }
                    frame True {
                      n770 = xnode "Read/Write Control"("FPGA VI Reference In"=w1212, "error in"=w1211) -> ("FPGA VI Reference Out"=w1209:refnum<k20>, "error out"=w1208:errorcluster, "timeTrial_count"=w1203:u32)
                      n771 = Multiply(x=w1202, y=1000.0) -> (x*y=w1206:dbl)
                      n772 = To Double Precision Float(number=w1203) -> (double precision float=w1205:dbl)
                      n773 = Divide(x=w1205, y=w1206) -> (x/y=w1207:dbl)
                      n774 = local write "FPGA_count2ms"(w1207) -> ()
                      n775 = xnode "Read/Write Control"("FPGA VI Reference In"=w1209, "error in"=w1208, "timeTrial_trig"=FALSE ("timeTrial")) -> ("error out"=w1201:errorcluster)  [unwired: 1 out]
                    }
                  }
                }
              }
              "error out 5" <- w1176
              n776 = Select(t=myRIO_BRig_RT__Case_NonExp_stateList."Idle" ("Enum"), s=w1175, f=w1173) -> (s? t:f=w1172:T1)
            }
            frame "End" {
            }
          }
          n777 = local read "MTrig_Audio_trig__R"() -> (w89:bool)
          n778 = local read "MTrig_Audio_trig__L"() -> (w90:bool)
          n779 = local read "MTrig_Laser_trig"() -> (w88:bool)
          n780 = Compound Arithmetic op=OR(w90, w89, w88) -> (w87:bool)
          n781 = local read "START"() -> (w113:bool)
          n782 = local read "STOP_abort"() -> (w112:bool)
          n783 = case shown="True" w87 {
            frame False {
            }
            frame True {
              w129 = FALSE
              n784 = local write "MTrig_Audio_trig__R"(w129) -> ()
              n785 = local write "MTrig_Audio_trig__L"(w129) -> ()
              n786 = local write "MTrig_Laser_trig"(w129) -> ()
            }
          }
          n787 = call "myRIO_BRig_RT_dataMTrig_main__v2.vi"("input_dataMTrig"=w116, "input_Audio_trig_L"=w90, "input_Audio_trig_R"=w89, "input_Laser_trig"=w88) -> ("output_dataMTrig"=w115:u16[], "output_Audio_L"=w107:bool, "output_Audio_R"=w108:bool, "output_Laser"=w86:bool)  [unwired: 12 in]
          n788 = Or(x=w113, y=w112) -> (x .or. y?=w111:bool)
          n789 = Select(t=myRIO_BRig_RT__Case_NonExp_stateList."End" ("Enum"), s=w111, f=w110) -> (s? t:f=w109:T1)
          n790 = Not(x="MTrig_Laser_Switch") -> (.not. x?=w83:bool)
          n791 = And(x=w86, y=w83) -> (x .and. y?=w84:bool)
          n792 = And(x=w86, y="MTrig_Laser_Switch") -> (x .and. y?=w85:bool)
          n793 = xnode "Read/Write Control"("FPGA VI Reference In"=w96, "error in"=w95, "A1_SR"=w117, "A3_SL"=w118, "audioTrigger_L"=w107, "audioTrigger_R"=w108, "LC_Laser_l1"=w84, "LC_Laser_l2"=w85) -> ("FPGA VI Reference Out"=w123:refnum<k20>, "error out"=w122:errorcluster)
          n794 = node-c288() -> ()  [unwired: 1 in, 1 out]
          "cState_NonExp" <- w121
        }
        n795 = node-c288(w70) -> ()  [unwired: 1 out]
        n796 = flat-sequence {
          tunnel: w63 -> [w81]
          tunnel: [w81] -> w62
          tunnel: w61 -> [w80]
          tunnel: [w80] -> w60
          frame #0 {
            w79 = FALSE
            n797 = local write "STOP_endBlock"(w79) -> ()
            n798 = local write "STOP_endTrial"(w79) -> ()
          }
        }
      }
      frame True {
        w1224 = u16 0
        w1242 = u8 0
        w1243 = u16 0 ("idxDataBlock")
        w1245 = u16 100 ("new element/subarray")
        w1246 = u16 100 ("new element/subarray")
        w1266 = T6 refnum items=["Session NI_WebDAV"] ("output_hSession")
        w1275 = FALSE
        w1276 = u16 0
        # "dummyState counter"
        # "audio__L\naudio__R"
        # "Audio params"
        # "nRewards"
        # "idxDataBlock"
        # "Solenoid_Tdelay_R"
        # "Solenoid_Tdelay_L"
        # "RewCalib_N__R"
        # "RewCalib_N__L"
        # "Save dataLick to file\nSend file to Host\nSave dataMTrig\nSend file to Host\nDisconnect"
        # "dataTrial"
        # "dataTrial"
        # "Solenoid_Tcycle_R"
        # "Solenoid_Tcycle_L"
        # "Laser_Tcycle"
        # "Audio_Tcycle_R"
        # "Audio_Tcycle_L"
        # "dataLick"
        # "dataLC"
        # "dataLC"
        # "dataBlock"
        # "dataBlock"
        # "dataMTrig"
        # "dataMTrig"
        # "dataExp"
        # "dataCurrent"
        # "dataExp"
        # "dataCurrent"
        # "spout"
        # "state"
        n799 = call "myRIO_BRig_RT_dataMTrig_Solenoid_Tcycle__L.vi"() -> ("output_Solenoid_Tcycle__L"=w1272:i32)  [unwired: 11 in]
        n800 = call "myRIO_BRig_RT_dataMTrig_Solenoid_Tcycle__R.vi"() -> ("output_Solenoid_Tcycle__R"=w1271:i32)  [unwired: 11 in]
        n801 = call "myRIO_BRig_RT_dataMTrig_Audio_Tcycle__L.vi"() -> ("output_Audio_Tcycle__L"=w1270:i32)  [unwired: 11 in]
        n802 = call "myRIO_BRig_RT_dataMTrig_Audio_Tcycle__R.vi"() -> ("output_Audio_Tcycle__R"=w1269:i32)  [unwired: 11 in]
        n803 = call "myRIO_BRig_RT_dataMTrig_Laser_Tcycle.vi"() -> ("output_Laser_Tcycle"=w1268:i32)  [unwired: 11 in]
        n804 = local read "MTrig_Solenoid_Tcycle__L"() -> (w1251:u16)
        n805 = local read "MTrig_Solenoid_Tcycle__R"() -> (w1250:u16)
        n806 = local read "Tcycle_Reward_L"() -> (w1247:u16)
        n807 = local read "Tcycle_Reward_R"() -> (w1248:u16)
        n808 = local read "MTrig_Laser_Tcycle"() -> (w1249:u16)
        n809 = call "myRIO_BRig_RT_dataMTrig_Solenoid_RewCalib_nCycle__L.vi"() -> ("output_Solenoid_RewCalib_nCycle__L"=w1254:i32)  [unwired: 11 in]
        n810 = call "myRIO_BRig_RT_dataMTrig_Solenoid_Tdelay__L.vi"() -> ("output_Solenoid_Tdelay__L"=w1256:i32)  [unwired: 11 in]
        n811 = call "myRIO_BRig_RT_dataMTrig_Solenoid_RewCalib_nCycle__R.vi"() -> ("output_Solenoid_RewCalib_nCycle__R"=w1255:i32)  [unwired: 11 in]
        n812 = call "myRIO_BRig_RT_dataMTrig_Solenoid_Tdelay__R.vi"() -> ("output_Solenoid_Tdelay__R"=w1257:i32)  [unwired: 11 in]
        n813 = case shown="False" w1234 {
          selector: w1234 -> [_ w1298]
          tunnel: w1233 -> [w1295 w1300]
          tunnel: [w1296 w1300] -> w1229
          tunnel: w1232 -> [_ w1299]
          tunnel: [w1297 w1299] -> w1230
          tunnel: [w1294 w1298] -> w1228
          frame False {
            n814 = call "myRIO__TCP_connect_forWriting.vi"("input_error"=w1295) -> ("output_error"=w1296:errorcluster, "output_connected"=w1294:bool, "output_hTCP"=w1297:refnum<k5>)  [unwired: 8 in]
          }
          frame True {
          }
        }
        n815 = call "myRIO_BRig_RT_dataLick_init.vi"() -> ("output_dataLick"=w1278:u16[][])  [unwired: 11 in]
        n816 = call "myRIO_BRig_RT_dataCurrent_init.vi"() -> ("output_dataCurrent"=w1285:u16[])  [unwired: 11 in]
        n817 = call "myRIO_BRig_RT_dataExp_init.vi"() -> ("output_dataExp"=w1284:u16[])  [unwired: 11 in]
        n818 = call "myRIO_BRig_RT_dataMTrig_init.vi"() -> ("output_dataMTrig"=w1274:u16[])  [unwired: 5 in]
        n819 = call "myRIO_BRig_RT_dataLC_init.vi"() -> ("output_dataLC"=w1282:u16[])  [unwired: 11 in]
        n820 = call "myRIO_BRig_RT_dataBlock_init.vi"() -> ("output_dataBlock"=w1283:u16[][])  [unwired: 11 in]
        n821 = call "myRIO_BRig_RT_dataTrial_init.vi"() -> ("output_dataTrial"=w1267:u16[][])  [unwired: 11 in]
        n822 = local write "I_connect_TCP"(w1228) -> ()
        n823 = Replace Array Subset(array=w1274, new element #1=w1246, index #1=w1254, new element #2=w1246, index #2=w1255, new element #3=w1245, index #3=w1256, new element #4=w1245, index #4=w1257, new element #5=w1251, index #5=w1272, new element #6=w1250, index #6=w1271, new element #7=w1247, index #7=w1270, new element #8=w1248, index #8=w1269, new element #9=w1249, index #9=w1268) -> (w1273:u16[])
        n824 = call "myRIO_BRig_RT_dataAnalog_init.vi"() -> ("output_dataAnalog"=w1239:u16[][])  [unwired: 11 in]
        n825 = call "myRIO_BRig_RT_TCP__start_exp.vi"("input_hTCP"=w1230, "input_I_connected_TCP"=w1228, "input_error"=w1229) -> ("output_hTCP"=w1227:refnum<k5>, "output_error"=w1226:errorcluster)  [unwired: 11 in]
        n826 = Get Date/Time In Seconds() -> (seconds since 1Jan1904=w1253:timestamp)
        n827 = call "myRIO_BRig_RT_arrTrig_init.vi"() -> ("output_arrTrig"=w1223:bool[])  [unwired: 11 in]
        n828 = To Double Precision Float(number=w1253) -> (double precision float=w1252:dbl)
        n829 = node-c288() -> (w1293:T3)  [unwired: 4 in]
        n830 = timed-loop {
          timing: w1293 -> [_]
          timing-out: [_] -> w1292
          shift-right: [w1418] -> _
          shift-left: myRIO_BRig_RT__Case_Exp_stateList."Start1" ("Enum") -> [w1370]
          shift-right: [w1367] -> _
          shift-left: enum16{"Left", "Right"}."Left" -> [w1467]
          tunnel: w1222 -> [w1465]
          tunnel: w1221 -> [w1464]
          shift-right: [w1459] -> _
          shift-left: w1290 -> [w1463]
          shift-right: [w1458] -> _
          shift-left: w1289 -> [w1462]
          tunnel: [w1441] -> w1287
          tunnel: [w1442] -> w1288
          shift-right: [w1443] -> w1258
          shift-left: w1285 -> [w1410]
          shift-right: [w1457] -> _
          shift-left: w1284 -> [w1408]
          shift-right: [w1430] -> w1262
          shift-left: w1273 -> [w1431]
          shift-right: [w1455] -> _
          shift-left: w1283 -> [w1456]
          shift-right: [w1453] -> _
          shift-left: w1282 -> [w1454]
          shift-right: [w1445] -> w1264
          shift-left: w1278 -> [w1446]
          shift-right: [w1432] -> _
          shift-left: w1276 -> [w1440]
          shift-right: [w1405] -> _
          shift-left: w1242 -> [w1439]
          shift-right: [w1433] -> _
          shift-left: w1276 -> [w1438]
          shift-right: [w1434] -> _
          shift-left: w1242 -> [w1437]
          shift-right: [w1406] -> _
          shift-left: w1275 -> [w1435]
          shift-right: [w1407] -> _
          shift-left: w1275 -> [w1436]
          shift-right: [w1416] -> _
          shift-left: w1267 -> [w1417]
          shift-right: [w1415] -> w1260
          shift-left: w1266 -> [w1413]
          shift-right: [w1414] -> w1261
          shift-left: FALSE ("output_Iconnected") -> [w1412]
          tunnel: "Data Set Prefix" -> [w1411]
          tunnel: [w1411] -> w1259
          tunnel: w1252 -> [w1409]
          shift-right: [w1403] -> _
          shift-left: 0 ("idxDataBlock") -> [w1404]
          shift-right: [w1400] -> _
          shift-left: w1243 -> [w1402]
          shift-right: [w1399] -> _
          shift-left: w1243 -> [w1401]
          shift-right: [w1389] -> w1237
          shift-left: 0 -> [w1373]
          shift-right: [w1368] -> _
          shift-left: w1224 -> [w1384]
          shift-right: [w1369] -> _
          shift-left: w1224 -> [w1380]
          shift-right: [w1393] -> _
          shift-left: FALSE -> [w1393]
          shift-right: [w1379] -> _
          shift-left: w1224 -> [w1387]
          shift-right: [w1390] -> w1238
          shift-left: w1239 -> [w1391]
          tunnel: w1227 -> [w1378]
          tunnel: [w1377] -> w1236
          tunnel: w1228 -> [w1374]
          tunnel: [w1374] -> w1235
          tunnel: w1226 -> [w1376]
          tunnel: [w1375] -> w1231
          shift-right: [w1365] -> _
          shift-left: u16 0 -> [w1366]
          shift-right: [w1363] -> _
          shift-left: w1224 -> [w1364]
          shift-right: [w1360] -> _
          shift-left: w1223 -> [w1361]
          stop <- w1452 stop-if-true
          # "arrTrig"
          # "arrTrig"
          # "LC_Laser_l2"
          # "LC_Event_l2"
          # "LC_Laser_l1"
          # "LC_Event_l1"
          # "CueLed"
          # "LC_Laser_l2"
          # "LC_Event_l2"
          # "LC_Laser_l1"
          # "LC_Event_l1"
          # "solenoid__R"
          # "solenoid__L"
          # "spout"
          # "iState"
          # "dataAnalog"
          # "index"
          # "iEvent"
          # "iBlock"
          # "iTrial"
          # "Laser"
          # "Audio R"
          # "Audio L"
          # "Solenoid R"
          # "Solenoid L"
          # "manual triggering"
          # "dataTrial"
          # "dataBlock"
          # "nRewards"
          # "dataExp"
          # "dataCurrent"
          # "audio__L\naudio__R"
          # "time stamp"
          # "Audio params"
          # "nRewards"
          # "idxDataBlock"
          # "idxDataBlock"
          # "activate"
          # "audio__L\naudio__R"
          # "amp__R\nfreq__R"
          # "amp__L\nfreq__L"
          # "dataLC"
          # "solenoid__R"
          # "solenoid__L"
          # "Did a lick occur?"
          # "Update lick counter"
          # "spout"
          # "spout"
          # "state"
          # "state"
          n831 = node-c288() -> ()  [unwired: 1 in, 1 out]
          n832 = local read "MTrig_Solenoid_trig__L"() -> (w1428:bool)
          n833 = local read "MTrig_Solenoid_trig__R"() -> (w1427:bool)
          n834 = local read "MTrig_Audio_trig__L"() -> (w1426:bool)
          n835 = local read "MTrig_Audio_trig__R"() -> (w1425:bool)
          n836 = xnode "Read/Write Control"("FPGA VI Reference In"=w1465, "error in"=w1464) -> ("FPGA VI Reference Out"=w1398:refnum<k20>, "error out"=w1397:errorcluster, "A2_LickL"=w1459:u32, "A4_LickR"=w1458:u32)
          "A2" <- w1459
          "A4" <- w1458
          n837 = local read "MTrig_Laser_trig"() -> (w1424:bool)
          n838 = Greater?(x=w1459, y=w1463) -> (0:w1461:bool)
          n839 = Greater?(x=w1458, y=w1462) -> (0:w1460:bool)
          n840 = Or(x=w1461, y=w1460) -> (x .or. y?=w1466:bool)
          n841 = call "myRIO_BRig_RT_dataMTrig_main.vi"("input_dataMTrig"=w1431, "input_Solenoid_trig_L"=w1428, "input_Solenoid_trig_R"=w1427, "input_Audio_trig_L"=w1426, "input_Audio_trig_R"=w1425, "input_Laser_trig"=w1424) -> ("output_Laser"=w1356:bool, "output_dataMTrig"=w1430:u16[], "output_Solenoid_L"=w1359:bool, "output_Solenoid_R"=w1420:bool, "output_Audio_L"=w1422:bool, "output_Audio_R"=w1423:bool)  [unwired: 8 in]
          n842 = Compound Arithmetic op=OR(w1428, w1427, w1426, w1425, w1424) -> (w1429:bool)
          n843 = case shown="True" w1429 {
            frame False {
            }
            frame True {
              w1468 = FALSE
              n844 = local write "MTrig_Solenoid_trig__L"(w1468) -> ()
              n845 = local write "MTrig_Solenoid_trig__R"(w1468) -> ()
              n846 = local write "MTrig_Audio_trig__L"(w1468) -> ()
              n847 = local write "MTrig_Audio_trig__R"(w1468) -> ()
              n848 = local write "MTrig_Laser_trig"(w1468) -> ()
            }
          }
          n849 = case shown="\"ENL1_pre\"" w1370 {
            selector: w1370 -> [_ _ _ _ _ _ _ _ _ _ _ _ _ _ _ _ _ _ _ _ _ _ _ _ _ _ w2530 _ w2585 _ _ _ _ _ w2702 _ w2769 _ _ _ _ _ w2888 _ w2959 _ w3023 _ w3067 _ _ w3137 _ _ _ _ _ w3308 _ _ _ _ _ _ _ _ _ _ _ _ w3589 w3622]
            tunnel: [myRIO_BRig_RT__Case_Exp_stateList."Start2" ("Enum") myRIO_BRig_RT__Case_Exp_stateList."Start3" ("Enum") myRIO_BRig_RT__Case_Exp_stateList."saveSettings1" ("Enum") myRIO_BRig_RT__Case_Exp_stateList."saveSettings2" ("Enum") myRIO_BRig_RT__Case_Exp_stateList."saveSettings3" ("Enum") myRIO_BRig_RT__Case_Exp_stateList."saveSettings4" ("Enum") myRIO_BRig_RT__Case_Exp_stateList."saveSettings_LC_ENL_l1" ("Enum") myRIO_BRig_RT__Case_Exp_stateList."saveSettings_LC_ENL_l2" ("Enum") myRIO_BRig_RT__Case_Exp_stateList."saveSettings_LC_Cue_l1" ("Enum") myRIO_BRig_RT__Case_Exp_stateList."saveSettings_LC_Cue_l2" ("Enum") myRIO_BRig_RT__Case_Exp_stateList."saveSettings6_LC_l1_Other" ("Enum") myRIO_BRig_RT__Case_Exp_stateList."SaveSettings6_LC_l2_Other" ("Enum") myRIO_BRig_RT__Case_Exp_stateList."setSettings_Audio" ("Enum") myRIO_BRig_RT__Case_Exp_stateList."setSettings_Laser" ("Enum") myRIO_BRig_RT__Case_Exp_stateList."commConnect" ("Enum") w2251 myRIO_BRig_RT__Case_Exp_stateList."initTrial" ("Enum") w2296 myRIO_BRig_RT__Case_Exp_stateList."initTrial3" ("Enum") myRIO_BRig_RT__Case_Exp_stateList."initTrial_LC_ENL1" ("Enum") myRIO_BRig_RT__Case_Exp_stateList."ENL1_pre" ("Enum") myRIO_BRig_RT__Case_Exp_stateList."initTrial_LC_Cue1" ("Enum") myRIO_BRig_RT__Case_Exp_stateList."initTrial_LC_Cue1_2" ("Enum") myRIO_BRig_RT__Case_Exp_stateList."initTrial_LC_Sel" ("Enum") myRIO_BRig_RT__Case_Exp_stateList."initTrial4" ("Enum") w2501 w2527 myRIO_BRig_RT__Case_Exp_stateList."ENL1Penalty" ("Enum") w2586 myRIO_BRig_RT__Case_Exp_stateList."endExp" ("Enum") myRIO_BRig_RT__Case_Exp_stateList."endExp" ("Enum") myRIO_BRig_RT__Case_Exp_stateList."endExp" ("Enum") myRIO_BRig_RT__Case_Exp_stateList."endExp" ("Enum") w2675 w2701 myRIO_BRig_RT__Case_Exp_stateList."Cue1Penalty" ("Enum") w2767 myRIO_BRig_RT__Case_Exp_stateList."endExp" ("Enum") myRIO_BRig_RT__Case_Exp_stateList."endExp" ("Enum") myRIO_BRig_RT__Case_Exp_stateList."endExp" ("Enum") myRIO_BRig_RT__Case_Exp_stateList."endExp" ("Enum") w2858 w2887 myRIO_BRig_RT__Case_Exp_stateList."SelectReward" ("Enum") w2960 myRIO_BRig_RT__Case_Exp_stateList."SelectRewardPost" ("Enum") w3024 myRIO_BRig_RT__Case_Exp_stateList."SelectWrong" ("Enum") w3063 myRIO_BRig_RT__Case_Exp_stateList."endTrial1" ("Enum") myRIO_BRig_RT__Case_Exp_stateList."SelectTimeout" ("Enum") w3139 myRIO_BRig_RT__Case_Exp_stateList."endTrial1" ("Enum") myRIO_BRig_RT__Case_Exp_stateList."endTrial2" ("Enum") myRIO_BRig_RT__Case_Exp_stateList."endTrial3" ("Enum") w3225 w3291 w3308 myRIO_BRig_RT__Case_Exp_stateList."initBlock" ("Enum") w3335 myRIO_BRig_RT__Case_Exp_stateList."commUpload_dataExp" ("Enum") myRIO_BRig_RT__Case_Exp_stateList."endBlock" ("Enum") myRIO_BRig_RT__Case_Exp_stateList."commUpload_dataLC" ("Enum") myRIO_BRig_RT__Case_Exp_stateList."commUpload_dataTrial" ("Enum") myRIO_BRig_RT__Case_Exp_stateList."commUpload_dataCurrent" ("Enum") myRIO_BRig_RT__Case_Exp_stateList."saveData_dataCurrent" ("Enum") myRIO_BRig_RT__Case_Exp_stateList."saveData_dataExp" ("Enum") myRIO_BRig_RT__Case_Exp_stateList."saveData_dataLC" ("Enum") myRIO_BRig_RT__Case_Exp_stateList."saveData_dataTrial" ("Enum") myRIO_BRig_RT__Case_Exp_stateList."commUpload_pre" ("Enum") w3588 w3621] -> w1418
            tunnel: [w1497 w1516 w1538 w1599 w1653 w1721 w1788 w1852 w1916 w1980 w2044 w2087 w2131 w2157 w2222 w2228 w2259 w2273 w2310 w2352 w2382 w2406 w2429 w2446 w2483 w2515 w2543 w2568 w2590 w2606 w2628 w2647 w2666 w2674 w2723 w2743 w2766 w2787 w2808 w2827 w2846 w2869 w2909 w2934 w2957 w2971 w3021 w3045 w3077 w3098 w3118 w3149 w3172 w3184 w3203 w3245 w3264 w3307 w3324 w3338 w3372 w3393 w3414 w3435 w3456 w3484 w3504 w3531 w3551 w3575 w3609 w3642] -> w1367
            tunnel: w1467 -> [w1497 w1516 w1538 w1599 w1653 w1721 w1788 w1852 w1916 w1980 w2044 w2087 w2131 w2157 w2222 w2250 w2259 w2273 w2310 w2352 w2382 w2406 w2429 w2446 w2483 w2515 w2543 w2568 w2590 w2606 w2628 w2647 w2666 w2674 w2723 w2743 w2766 w2787 w2808 w2827 w2846 w2869 w2909 w2934 w2957 w2971 w3021 w3045 w3077 w3098 w3118 w3149 w3172 w3184 w3203 w3245 w3264 w3307 w3324 w3338 w3372 w3393 w3414 w3435 w3456 w3484 w3504 w3531 w3551 w3575 w3609 w3642]
            tunnel: w1466 -> [w1500 w1519 w1535 w1602 w1656 w1724 w1791 w1855 w1919 w1983 w2047 w2090 w2134 w2160 w2225 w2244 w2270 w2297 w2334 w2368 w2396 w2419 w2442 w2471 w2496 w2502 w2526 w2571 w2593 w2612 w2631 w2650 w2669 w2678 w2700 w2751 w2773 w2792 w2811 w2830 w2849 w2867 w2907 w2944 w2967 w3002 w3029 w3056 w3080 w3097 w3130 w3154 w3169 w3192 w3202 w3256 w3290 w3311 w3321 w3347 w3375 w3396 w3417 w3438 w3459 w3487 w3507 w3534 w3554 w3578 w3612 w3645]
            tunnel: w1461 -> [w1499 w1518 w1536 w1601 w1655 w1723 w1790 w1854 w1918 w1982 w2046 w2089 w2133 w2159 w2224 w2243 w2269 w2298 w2333 w2369 w2397 w2420 w2443 w2472 w2497 w2519 w2545 w2570 w2592 w2611 w2630 w2649 w2668 w2692 w2724 w2750 w2772 w2791 w2810 w2829 w2848 w2868 w2906 w2943 w2966 w3001 w3028 w3055 w3079 w3096 w3129 w3153 w3170 w3193 w3201 w3255 w3289 w3310 w3322 w3348 w3374 w3395 w3416 w3437 w3458 w3486 w3506 w3533 w3553 w3577 w3611 w3644]
            tunnel: w1460 -> [w1498 w1517 w1537 w1600 w1654 w1722 w1789 w1853 w1917 w1981 w2045 w2088 w2132 w2158 w2223 w2242 w2268 w2299 w2332 w2370 w2398 w2421 w2444 w2473 w2498 w2518 w2544 w2569 w2591 w2610 w2629 w2648 w2667 w2691 w2725 w2749 w2771 w2790 w2809 w2828 w2847 w2879 w2910 w2942 w2965 w3000 w3027 w3054 w3078 w3095 w3128 w3152 w3171 w3194 w3200 w3254 w3288 w3309 w3323 w3349 w3373 w3394 w3415 w3436 w3457 w3485 w3505 w3532 w3552 w3576 w3610 w3643]
            tunnel: [w1500 w1519 w1535 w1602 w1656 w1724 w1791 w1855 w1919 w1983 w2047 w2090 w2134 w2160 w2225 w2244 w2270 w2297 w2334 w2368 w2396 w2419 w2442 w2471 w2496 w2502 w2526 w2571 w2593 w2612 w2631 w2650 w2669 w2678 w2700 w2751 w2773 w2792 w2811 w2830 w2849 w2867 w2907 w2944 w2967 w3002 w3029 w3056 w3080 w3097 w3130 w3154 w3169 w3192 w3202 w3256 w3290 w3311 w3321 w3347 w3375 w3396 w3417 w3438 w3459 w3487 w3507 w3534 w3554 w3578 w3612 w3645] -> w1449
            tunnel: [w1499 w1518 w1536 w1601 w1655 w1723 w1790 w1854 w1918 w1982 w2046 w2089 w2133 w2159 w2224 w2243 w2269 w2298 w2333 w2369 w2397 w2420 w2443 w2472 w2497 w2519 w2545 w2570 w2592 w2611 w2630 w2649 w2668 w2692 w2724 w2750 w2772 w2791 w2810 w2829 w2848 w2868 w2906 w2943 w2966 w3001 w3028 w3055 w3079 w3096 w3129 w3153 w3170 w3193 w3201 w3255 w3289 w3310 w3322 w3348 w3374 w3395 w3416 w3437 w3458 w3486 w3506 w3533 w3553 w3577 w3611 w3644] -> w1448
            tunnel: [w1498 w1517 w1537 w1600 w1654 w1722 w1789 w1853 w1917 w1981 w2045 w2088 w2132 w2158 w2223 w2242 w2268 w2299 w2332 w2370 w2398 w2421 w2444 w2473 w2498 w2518 w2544 w2569 w2591 w2610 w2629 w2648 w2667 w2691 w2725 w2749 w2771 w2790 w2809 w2828 w2847 w2879 w2910 w2942 w2965 w3000 w3027 w3054 w3078 w3095 w3128 w3152 w3171 w3194 w3200 w3254 w3288 w3309 w3323 w3349 w3373 w3394 w3415 w3436 w3457 w3485 w3505 w3532 w3552 w3576 w3610 w3643] -> w1447
            tunnel: w1410 -> [w1496 w1515 w1534 w1566 w1629 w1698 w1773 w1851 w1915 w1979 w2043 w2086 w2130 w2155 w2198 w2249 w2258 w2295 w2309 w2353 w2381 w2405 w2428 w2456 w2482 w2503 w2529 w2562 w2589 w2607 w2627 w2646 w2665 w2677 w2720 w2742 w2770 w2788 w2807 w2826 w2845 w2860 w2890 w2926 w2962 w2973 w3026 w3046 w3076 w3094 w3119 w3151 w3168 w3181 w3205 w3227 w3262 w3306 w3325 w3350 w3369 w3390 w3411 w3432 w3443 w3473 w3492 w3516 w3548 w3564 w3587 w3620]
            tunnel: w1408 -> [w1495 w1514 w1533 w1597 w1651 w1718 w1785 w1849 w1913 w1977 w2041 w2084 w2128 w2148 w2218 w2248 w2267 w2294 w2317 w2351 w2384 w2409 w2432 w2461 w2486 w2517 w2542 w2561 w2587 w2609 w2626 w2645 w2664 w2673 w2722 w2740 w2765 w2789 w2806 w2825 w2844 w2850 w2908 w2940 w2964 w2994 w3022 w3047 w3074 w3093 w3121 w3148 w3167 w3191 w3208 w3226 w3281 w3305 w3326 w3351 w3368 w3389 w3410 w3431 w3444 w3481 w3501 w3512 w3547 w3572 w3606 w3639]
            tunnel: [w1496 w1515 w1534 w1566 w1629 w1697 w1772 w1851 w1915 w1979 w2043 w2086 w2130 w2155 w2204 w2233 w2258 w2283 w2309 w2353 w2381 w2404 w2427 w2455 w2481 w2500 w2528 w2563 w2588 w2607 w2627 w2646 w2665 w2676 w2719 w2741 w2768 w2788 w2807 w2826 w2845 w2859 w2889 w2941 w2961 w2995 w3025 w3048 w3075 w3094 w3122 w3150 w3168 w3180 w3204 w3227 w3260 w3306 w3325 w3350 w3369 w3390 w3411 w3432 w3443 w3473 w3492 w3516 w3548 w3564 w3587 w3620] -> w1444
            tunnel: [w1495 w1514 w1533 w1596 w1650 w1713 w1784 w1849 w1913 w1977 w2041 w2084 w2128 w2148 w2218 w2247 w2267 w2293 w2317 w2351 w2384 w2409 w2432 w2461 w2486 w2517 w2542 w2561 w2587 w2609 w2626 w2645 w2664 w2673 w2722 w2740 w2765 w2789 w2806 w2825 w2844 w2850 w2908 w2940 w2964 w2994 w3022 w3047 w3074 w3093 w3121 w3148 w3167 w3191 w3208 w3226 w3281 w3305 w3326 w3351 w3368 w3389 w3410 w3431 w3444 w3481 w3501 w3515 w3547 w3572 w3606 w3639] -> w1457
            tunnel: [_ _ _ _ _ _ _ _ _ _ _ _ _ _ _ _ _ _ _ _ _ _ _ _ _ _ _ _ _ _ _ _ _ _ _ _ _ _ _ _ _ _ _ _ w2955 _ _ _ _ _ _ _ _ _ _ _ _ _ _ _ _ _ _ _ _ _ _ _ _ _ _ _] -> w1358
            tunnel: [_ _ _ _ _ _ _ _ _ _ _ _ _ _ _ _ _ _ _ _ _ _ _ _ _ _ _ _ _ _ _ _ _ _ _ _ _ _ _ _ _ _ _ _ w2956 _ _ _ _ _ _ _ _ _ _ _ _ _ _ _ _ _ _ _ _ _ _ _ _ _ _ _] -> w1421
            tunnel: w1456 -> [w1493 w1512 w1531 w1568 w1631 w1719 w1786 w1850 w1914 w1978 w2042 w2085 w2129 w2153 w2219 w2245 w2260 w2291 w2325 w2366 w2394 w2401 w2424 w2445 w2478 w2516 w2541 w2558 w2583 w2608 w2624 w2643 w2662 w2690 w2721 w2739 w2763 w2785 w2804 w2823 w2842 w2878 w2904 w2932 w2963 w2975 w3019 w3044 w3072 w3091 w3120 w3147 w3165 w3183 w3210 w3252 w3273 w3303 w3328 w3353 w3366 w3387 w3408 w3429 w3453 w3467 w3494 w3522 w3541 w3566 w3600 w3633]
            tunnel: [w1493 w1512 w1531 w1568 w1631 w1719 w1786 w1850 w1914 w1978 w2042 w2085 w2129 w2153 w2219 w2245 w2257 w2291 w2325 w2366 w2394 w2401 w2424 w2445 w2478 w2516 w2541 w2558 w2583 w2608 w2624 w2643 w2662 w2690 w2721 w2739 w2763 w2785 w2804 w2823 w2842 w2878 w2904 w2932 w2963 w2974 w3019 w3044 w3072 w3091 w3120 w3147 w3165 w3182 w3210 w3252 w3273 w3303 w3328 w3353 w3366 w3387 w3408 w3429 w3453 w3467 w3494 w3522 w3541 w3566 w3600 w3633] -> w1455
            tunnel: w1454 -> [w1494 w1513 w1532 w1567 w1630 w1720 w1787 w1847 w1911 w1975 w2039 w2082 w2126 w2154 w2220 w2246 w2266 w2292 w2308 w2367 w2395 w2407 w2430 w2459 w2484 w2514 w2525 w2559 w2584 w2605 w2625 w2644 w2663 w2689 w2699 w2738 w2764 w2786 w2805 w2824 w2843 w2877 w2905 w2933 w2958 w2992 w3020 w3043 w3073 w3092 w3117 w3146 w3166 w3190 w3209 w3253 w3280 w3304 w3327 w3352 w3367 w3388 w3409 w3430 w3454 w3480 w3500 w3528 w3539 w3571 w3605 w3638]
            tunnel: [w1494 w1513 w1532 w1567 w1630 w1720 w1787 w1848 w1912 w1976 w2040 w2083 w2127 w2154 w2220 w2246 w2266 w2292 w2308 w2367 w2395 w2407 w2430 w2459 w2484 w2514 w2525 w2559 w2584 w2605 w2625 w2644 w2663 w2689 w2699 w2738 w2764 w2786 w2805 w2824 w2843 w2877 w2905 w2933 w2958 w2992 w3020 w3043 w3073 w3092 w3117 w3146 w3166 w3190 w3209 w3253 w3280 w3304 w3327 w3352 w3367 w3388 w3409 w3430 w3454 w3480 w3500 w3528 w3539 w3571 w3605 w3638] -> w1453
            tunnel: [_ _ _ _ _ _ _ _ _ _ _ _ _ _ _ _ _ _ _ _ _ _ _ _ _ _ _ _ _ _ _ _ _ _ _ _ _ _ _ _ _ _ _ _ _ _ _ _ _ _ _ _ _ _ _ _ _ TRUE _ _ _ _ _ _ _ _ _ _ _ _ _ _] -> w1450
            tunnel: w1440 -> [w1491 w1510 w1529 w1558 w1624 w1708 w1783 w1834 w1903 w1962 w2026 w2054 w2108 _ w2210 w2241 w2265 w2290 w2324 w2365 w2393 w2418 w2441 w2470 w2495 w2513 w2540 w2556 w2582 w2603 w2622 w2641 w2660 w2688 w2716 w2736 w2762 w2783 w2802 w2821 w2840 w2876 w2903 w2922 w2954 w2990 w3018 w3041 w3071 w3090 w3115 w3145 w3164 w3188 w3214 w3251 w3277 w3301 w3319 w3346 w3364 w3385 w3406 w3427 w3451 w3478 w3498 w3526 w3545 w3570 w3604 w3637]
            tunnel: w1439 -> [w1490 w1509 w1528 w1557 w1623 w1707 w1782 w1833 w1902 w1961 w2025 w2055 w2109 _ w2209 w2240 w2264 w2289 w2323 w2364 w2392 w2417 w2440 w2469 w2494 w2512 w2539 w2555 w2581 w2602 w2621 w2640 w2659 w2687 w2715 w2735 w2761 w2782 w2801 w2820 w2839 w2875 w2902 w2921 w2953 w2989 w3017 w3040 w3070 w3089 w3114 w3144 w3163 w3187 w3213 w3250 w3276 w3300 w3318 w3345 w3363 w3384 w3405 w3426 w3450 w3477 w3497 w3525 w3544 w3569 w3603 w3636]
            tunnel: w1438 -> [w1489 w1508 w1527 w1556 w1622 w1706 w1781 w1832 w1901 w1960 w2024 w2056 w2110 _ w2208 w2239 w2263 w2288 w2322 w2363 w2391 w2416 w2439 w2468 w2493 w2511 w2538 w2554 w2580 w2601 w2620 w2639 w2658 w2686 w2714 w2734 w2760 w2781 w2800 w2819 w2838 w2874 w2901 w2920 w2952 w2988 w3016 w3039 w3069 w3088 w3113 w3143 w3162 w3186 w3212 w3249 w3275 w3299 w3317 w3344 w3362 w3383 w3404 w3425 w3449 w3476 w3496 w3524 w3543 w3568 w3602 w3635]
            tunnel: w1437 -> [w1488 w1507 w1526 w1555 w1621 w1705 w1780 w1831 w1900 w1959 w2023 w2057 w2111 _ w2207 w2238 w2262 w2287 w2321 w2362 w2390 w2415 w2438 w2467 w2492 w2510 w2537 w2553 w2579 w2600 w2619 w2638 w2657 w2685 w2713 w2733 w2759 w2780 w2799 w2818 w2837 w2873 w2900 w2919 w2951 w2987 w3015 w3038 w3068 w3087 w3112 w3142 w3161 w3185 w3211 w3248 w3274 w3298 w3316 w3343 w3361 w3382 w3403 w3424 w3448 w3475 w3495 w3523 w3542 w3567 w3601 w3634]
            tunnel: w1436 -> [_ _ _ _ _ _ _ _ _ _ _ _ _ _ _ _ _ _ _ _ _ _ _ _ _ _ _ _ _ _ _ _ _ _ w2718 _ _ _ _ _ _ _ _ _ _ _ _ _ _ _ _ _ _ _ _ _ _ _ _ _ _ _ _ _ _ _ _ _ _ _ _ _]
            tunnel: w1435 -> [_ _ _ _ _ _ _ _ _ _ _ _ _ _ _ _ _ _ _ _ _ _ _ _ _ _ _ _ _ _ _ _ _ _ w2717 _ _ _ _ _ _ _ _ _ _ _ _ _ _ _ _ _ _ _ _ _ _ _ _ _ _ _ _ _ _ _ _ _ _ _ _ _]
            tunnel: [w1491 w1510 w1529 w1558 w1624 w1708 w1783 w1834 w1903 w1962 w2026 w2054 w2108 w2147 w2210 w2241 w2265 w2290 w2324 w2365 w2393 w2418 w2441 w2470 w2495 w2513 w2540 w2556 w2582 w2603 w2622 w2641 w2660 w2688 w2716 w2736 w2762 w2783 w2802 w2821 w2840 w2876 w2903 w2922 w2954 w2990 w3018 w3041 w3071 w3090 w3115 w3145 w3164 w3188 w3214 w3251 w3277 w3301 w3319 w3346 w3364 w3385 w3406 w3427 w3451 w3478 w3498 w3526 w3545 w3570 w3604 w3637] -> w1432
            tunnel: [w1490 w1509 w1528 w1557 w1623 w1707 w1782 w1833 w1902 w1961 w2025 w2055 w2109 w2138 w2209 w2240 w2264 w2289 w2323 w2364 w2392 w2417 w2440 w2469 w2494 w2512 w2539 w2555 w2581 w2602 w2621 w2640 w2659 w2687 w2715 w2735 w2761 w2782 w2801 w2820 w2839 w2875 w2902 w2921 w2953 w2989 w3017 w3040 w3070 w3089 w3114 w3144 w3163 w3187 w3213 w3250 w3276 w3300 w3318 w3345 w3363 w3384 w3405 w3426 w3450 w3477 w3497 w3525 w3544 w3569 w3603 w3636] -> w1405
            tunnel: [w1489 w1508 w1527 w1556 w1622 w1706 w1781 w1832 w1901 w1960 w2024 w2056 w2110 w2146 w2208 w2239 w2263 w2288 w2322 w2363 w2391 w2416 w2439 w2468 w2493 w2511 w2538 w2554 w2580 w2601 w2620 w2639 w2658 w2686 w2714 w2734 w2760 w2781 w2800 w2819 w2838 w2874 w2901 w2920 w2952 w2988 w3016 w3039 w3069 w3088 w3113 w3143 w3162 w3186 w3212 w3249 w3275 w3299 w3317 w3344 w3362 w3383 w3404 w3425 w3449 w3476 w3496 w3524 w3543 w3568 w3602 w3635] -> w1433
            tunnel: [w1488 w1507 w1526 w1555 w1621 w1705 w1780 w1831 w1900 w1959 w2023 w2057 w2111 w2136 w2207 w2238 w2262 w2287 w2321 w2362 w2390 w2415 w2438 w2467 w2492 w2510 w2537 w2553 w2579 w2600 w2619 w2638 w2657 w2685 w2713 w2733 w2759 w2780 w2799 w2818 w2837 w2873 w2900 w2919 w2951 w2987 w3015 w3038 w3068 w3087 w3112 w3142 w3161 w3185 w3211 w3248 w3274 w3298 w3316 w3343 w3361 w3382 w3403 w3424 w3448 w3475 w3495 w3523 w3542 w3567 w3601 w3634] -> w1434
            tunnel: [_ _ _ _ _ _ _ _ _ _ _ _ _ _ _ _ _ _ _ _ _ _ _ _ _ _ _ _ _ _ _ _ _ w2672 w2718 _ _ _ _ _ _ _ _ _ _ _ _ _ _ _ _ _ _ _ _ _ _ _ _ _ _ _ _ _ _ _ _ _ _ _ _ _] -> w1407
            tunnel: [_ _ _ _ _ _ _ _ _ _ _ _ _ _ _ _ _ _ _ _ _ _ _ _ _ _ _ _ _ _ _ _ _ w2671 w2717 _ _ _ _ _ _ _ _ _ _ _ _ _ _ _ _ _ _ _ _ _ _ _ _ _ _ _ _ _ _ _ _ _ _ _ _ _] -> w1406
            tunnel: w1417 -> [w1487 w1506 w1525 w1554 w1620 w1704 w1779 w1830 w1899 w1958 w2022 w2053 w2107 w2145 w2217 w2237 w2261 w2286 w2312 w2355 w2380 w2403 w2426 w2457 w2480 w2509 w2536 w2552 w2578 w2599 w2618 w2637 w2656 w2684 w2712 w2732 w2758 w2779 w2798 w2817 w2836 w2872 w2899 w2916 w2950 w2986 w3014 w3035 w3062 w3086 w3109 w3136 w3160 w3179 w3207 w3241 w3272 w3297 w3329 w3354 w3365 w3386 w3407 w3428 w3452 w3479 w3499 w3527 w3546 w3561 w3599 w3632]
            tunnel: [w1487 w1506 w1525 w1554 w1620 w1704 w1779 w1830 w1899 w1958 w2022 w2053 w2107 w2145 w2217 w2237 w2261 w2286 w2311 w2354 w2373 w2402 w2425 w2457 w2479 w2509 w2536 w2552 w2578 w2599 w2618 w2637 w2656 w2684 w2712 w2732 w2758 w2779 w2798 w2817 w2836 w2872 w2899 w2916 w2950 w2986 w3014 w3035 w3062 w3086 w3109 w3136 w3160 w3179 w3206 w3241 w3272 w3297 w3329 w3354 w3365 w3386 w3407 w3428 w3452 w3479 w3499 w3527 w3546 w3561 w3599 w3632] -> w1416
            tunnel: [w1486 w1505 w1524 w1553 w1619 w1703 w1778 w1829 w1898 w1957 w2021 w2052 w2106 w2144 w2216 w2236 w2272 w2285 w2327 w2361 w2389 w2414 w2437 w2466 w2491 w2508 w2535 w2551 w2577 w2598 w2617 w2636 w2655 w2683 w2711 w2731 w2757 w2778 w2797 w2816 w2835 w2871 w2898 w2915 w2949 w2985 w3013 w3034 w3061 w3085 w3108 w3135 w3159 w3178 w3199 w3247 w3271 w3295 w3330 w3340 w3360 w3381 w3402 w3423 w3447 w3483 w3503 w3530 w3550 w3574 w3608 w3641] -> w1415
            tunnel: [w1485 w1504 w1523 w1552 w1618 w1702 w1777 w1828 w1897 w1956 w2020 w2051 w2105 w2143 w2215 w2235 w2271 w2284 w2326 w2360 w2388 w2413 w2436 w2465 w2490 w2507 w2534 w2550 w2576 w2597 w2616 w2635 w2654 w2682 w2710 w2730 w2756 w2777 w2796 w2815 w2834 w2870 w2897 w2914 w2948 w2984 w3012 w3033 w3060 w3084 w3107 w3134 w3158 w3177 w3198 w3246 w3270 w3296 w3312 w3337 w3370 w3391 w3412 w3433 w3455 w3482 w3502 w3529 w3549 w3573 w3607 w3640] -> w1414
            tunnel: w1413 -> [w1486 w1505 w1524 w1553 w1619 w1703 w1778 w1829 w1898 w1957 w2021 w2052 w2106 w2144 w2216 w2236 w2272 w2285 w2327 w2361 w2389 w2414 w2437 w2466 w2491 w2508 w2535 w2551 w2577 w2598 w2617 w2636 w2655 w2683 w2711 w2731 w2757 w2778 w2797 w2816 w2835 w2871 w2898 w2915 w2949 w2985 w3013 w3034 w3061 w3085 w3108 w3135 w3159 w3178 w3199 w3247 w3271 w3295 _ w3340 w3360 w3381 w3402 w3423 w3447 w3483 w3503 w3530 w3550 w3574 w3608 w3641]
            tunnel: w1412 -> [w1485 w1504 w1523 w1552 w1618 w1702 w1777 w1828 w1897 w1956 w2020 w2051 w2105 w2143 w2215 w2235 w2271 w2284 w2326 w2360 w2388 w2413 w2436 w2465 w2490 w2507 w2534 w2550 w2576 w2597 w2616 w2635 w2654 w2682 w2710 w2730 w2756 w2777 w2796 w2815 w2834 w2870 w2897 w2914 w2948 w2984 w3012 w3033 w3060 w3084 w3107 w3134 w3158 w3177 w3198 w3246 w3270 w3296 _ w3337 w3370 w3391 w3412 w3433 w3455 w3482 w3502 w3529 w3549 w3573 w3607 w3640]
            tunnel: w1411 -> [_ _ _ _ _ _ _ _ _ _ _ _ _ _ _ _ _ _ _ _ _ _ _ _ _ _ _ _ _ _ _ _ _ _ _ _ _ _ _ _ _ _ _ _ _ _ _ _ _ _ _ _ _ _ _ _ _ _ _ _ w3358 w3379 w3400 w3421 w3445 _ _ _ _ _ _ _]
            tunnel: w1409 -> [_ _ _ _ _ _ _ _ _ _ _ _ _ _ _ _ _ _ _ _ _ _ _ _ _ _ _ _ _ _ _ _ _ _ _ _ _ _ _ _ _ _ _ _ _ _ _ _ _ _ _ _ _ _ _ _ _ _ _ _ _ _ _ _ _ _ _ w3517 _ _ _ _]
            tunnel: [w1484 w1503 w1522 w1551 w1617 w1701 w1776 w1827 w1896 w1955 w2019 w2050 w2104 w2142 w2214 w2231 w2255 w2281 w2328 w2359 w2387 w2412 w2435 w2464 w2489 w2506 w2533 w2549 w2575 w2596 w2615 w2634 w2653 w2681 w2709 w2729 w2755 w2776 w2795 w2814 w2833 w2866 w2896 w2913 w2947 w2969 w3011 w3032 w3059 w3083 w3106 w3133 w3157 w3176 w3197 w3244 w3257 w3294 w3315 w3339 w3357 w3378 w3399 w3420 w3442 w3462 w3491 w3511 w3538 w3559 w3598 w3631] -> w1403
            tunnel: w1404 -> [w1484 w1503 w1522 w1551 w1617 w1701 w1776 w1827 w1896 w1955 w2019 w2050 w2104 w2142 w2214 w2231 _ w2281 w2328 w2359 w2387 w2412 w2435 w2464 w2489 w2506 w2533 w2549 w2575 w2596 w2615 w2634 w2653 w2681 w2709 w2729 w2755 w2776 w2795 w2814 w2833 w2866 w2896 w2913 w2947 w2969 w3011 w3032 w3059 w3083 w3106 w3133 w3157 w3176 w3197 w3244 w3258 w3294 w3315 w3339 w3357 w3378 w3399 w3420 w3442 w3462 w3491 w3511 w3538 w3559 w3598 w3631]
            tunnel: w1402 -> [w1483 w1502 w1521 w1550 w1616 w1700 w1775 w1826 w1895 w1954 w2018 w2049 w2103 w2141 w2213 w2230 w2254 w2280 w2320 w2358 w2386 w2411 w2434 w2463 w2488 w2505 w2532 w2548 w2574 w2595 w2614 w2633 w2652 w2680 w2708 w2728 w2754 w2775 w2794 w2813 w2832 w2865 w2895 w2912 w2946 w2983 w3010 w3031 w3058 w3082 w3105 w3132 w3156 w3175 w3196 w3243 w3269 w3293 w3314 w3342 w3356 w3377 w3398 w3419 w3441 w3461 w3490 w3510 w3537 w3558 w3597 w3630]
            tunnel: w1401 -> [w1482 w1501 w1520 w1549 w1615 w1699 w1774 w1825 w1894 w1953 w2017 w2048 w2102 w2140 w2212 w2229 w2253 w2279 w2319 w2357 w2385 w2410 w2433 w2462 w2487 w2504 w2531 w2547 w2573 w2594 w2613 w2632 w2651 w2679 w2707 w2727 w2753 w2774 w2793 w2812 w2831 w2864 w2894 w2911 w2945 w2980 w3009 w3030 w3057 w3081 w3104 w3131 w3155 w3174 w3195 w3242 w3268 w3292 w3313 w3341 w3355 w3376 w3397 w3418 w3440 w3460 w3489 w3509 w3536 w3557 w3596 w3629]
            tunnel: [w1483 w1502 w1521 w1550 w1616 w1700 w1775 w1826 w1895 w1954 w2018 w2049 w2103 w2141 w2213 w2230 w2254 w2280 w2320 w2358 w2386 w2411 w2434 w2463 w2488 w2505 w2532 w2548 w2574 w2595 w2614 w2633 w2652 w2680 w2708 w2728 w2754 w2775 w2794 w2813 w2832 w2865 w2895 w2912 w2946 w2982 w3010 w3031 w3058 w3082 w3105 w3132 w3156 w3175 w3196 w3243 w3269 w3293 w3314 w3342 w3356 w3377 w3398 w3419 w3441 w3461 w3490 w3510 w3537 w3558 w3597 w3630] -> w1400
            tunnel: [w1482 w1501 w1520 w1549 w1615 w1699 w1774 w1825 w1894 w1953 w2017 w2048 w2102 w2140 w2212 w2229 w2253 w2279 w2319 w2357 w2385 w2410 w2433 w2462 w2487 w2504 w2531 w2547 w2573 w2594 w2613 w2632 w2651 w2679 w2707 w2727 w2753 w2774 w2793 w2812 w2831 w2864 w2894 w2911 w2945 w2981 w3009 w3030 w3057 w3081 w3104 w3131 w3155 w3174 w3195 w3242 w3268 w3292 w3313 w3341 w3355 w3376 w3397 w3418 w3440 w3460 w3489 w3509 w3536 w3557 w3596 w3629] -> w1399
            tunnel: w1398 -> [w1481 _ _ _ _ _ _ _ _ _ _ _ _ _ w2205 _ _ _ w2331 w2347 _ _ _ _ _ _ _ _ _ _ _ _ _ _ w2704 _ _ _ _ _ _ w2862 w2893 _ _ _ _ _ _ _ w3103 _ _ _ _ w3223 _ _ _ _ _ _ _ _ _ _ _ _ _ _ _ _]
            tunnel: w1397 -> [w1480 _ _ _ _ _ _ _ _ _ _ _ _ _ w2206 _ _ _ w2330 w2346 _ _ _ _ _ _ _ _ _ _ _ _ _ _ w2703 _ _ _ _ _ _ w2863 w2892 _ _ _ _ _ _ _ w3102 _ _ _ _ w3222 _ _ _ _ _ _ _ _ _ _ _ _ _ _ _ _]
            tunnel: [_ _ _ _ _ _ _ _ _ _ _ _ _ _ _ _ _ _ _ _ _ _ _ _ _ _ w2523 _ _ _ _ _ _ _ w2697 _ _ _ _ _ _ w2854 w2883 _ _ _ _ _ _ _ _ _ _ _ _ _ _ _ _ _ _ _ _ _ _ _ _ _ _ _ _ _] -> w1349
            tunnel: [_ _ _ _ _ _ _ _ _ _ _ _ _ _ _ _ _ _ _ _ _ _ _ _ _ _ w2522 _ _ _ _ _ _ _ w2696 _ _ _ _ _ _ w2853 w2882 _ _ _ _ _ _ _ _ _ _ _ _ _ _ _ _ _ _ _ _ _ _ _ _ _ _ _ _ _] -> w1348
            tunnel: [_ _ _ _ _ _ _ _ _ _ _ _ _ _ _ _ _ _ _ _ _ _ _ w2458 w2477 _ _ _ _ _ _ _ _ _ _ _ _ _ _ _ _ _ _ _ _ _ _ _ _ _ _ _ _ _ _ _ _ _ _ _ _ _ _ _ _ _ _ _ _ _ _ _] -> w1395
            tunnel: [_ _ _ _ _ _ _ _ _ _ _ _ _ _ _ _ _ _ _ _ _ _ _ _ TRUE ("Recording") _ _ _ _ _ _ _ _ _ _ _ _ _ _ _ _ _ _ _ _ _ _ _ _ _ _ _ _ _ _ _ _ _ _ _ _ _ _ _ _ _ _ _ _ _ _ _] -> w1392
            tunnel: [_ _ _ _ _ _ _ _ _ _ _ _ _ _ _ _ _ _ _ _ _ _ _ w2458 _ _ _ _ _ _ _ _ _ _ _ _ _ _ _ _ _ _ _ _ _ _ _ _ _ _ _ _ _ _ _ _ _ _ _ _ _ _ _ _ _ _ _ _ _ _ _ _] -> w1388
            tunnel: [_ _ _ _ _ _ _ _ _ _ _ _ _ _ _ TRUE _ _ _ _ _ _ _ _ _ _ _ _ _ _ _ _ _ _ _ _ _ _ _ _ _ _ _ _ _ _ _ _ _ _ _ _ _ _ _ _ _ _ _ _ _ _ _ _ _ _ _ _ _ _ _ _] -> w1385
            tunnel: [_ _ _ _ _ _ _ _ _ _ _ _ _ _ _ w2226 _ _ _ _ _ _ _ _ _ _ _ _ _ _ _ _ _ _ _ _ _ _ _ _ _ _ _ _ _ _ _ _ _ _ _ _ _ _ _ _ _ _ _ _ _ _ _ _ _ _ _ _ _ _ _ _] -> w1383
            tunnel: [_ _ _ _ _ _ _ _ _ _ _ _ _ _ _ _ _ TRUE _ _ _ _ _ _ _ _ _ _ _ _ _ _ _ _ _ _ _ _ _ _ _ _ _ _ _ _ _ _ _ _ _ _ _ _ _ _ _ _ _ _ _ _ _ _ _ _ _ _ _ _ _ _] -> w1382
            tunnel: [_ _ _ _ _ _ _ _ _ _ _ _ _ _ _ _ _ w2274 _ _ _ _ _ _ _ _ _ _ _ _ _ _ _ _ _ _ _ _ _ _ _ _ _ _ _ _ _ _ _ _ _ _ _ _ _ _ _ _ _ _ _ _ _ _ _ _ _ _ _ _ _ _] -> w1381
            tunnel: w1366 -> [_ _ _ _ _ _ _ _ _ _ _ _ _ _ _ _ _ _ _ _ _ _ _ _ _ _ _ _ _ _ _ _ _ _ _ _ _ _ _ _ _ _ _ _ _ _ _ _ _ _ _ _ _ _ _ _ _ _ _ _ _ _ _ _ _ _ _ _ _ _ w3594 w3627]
            tunnel: [_ _ _ _ _ _ _ _ _ _ _ _ _ _ _ _ _ _ _ _ _ _ _ _ _ _ _ _ _ _ _ _ _ _ _ _ _ _ _ _ _ _ _ _ _ _ _ _ _ _ _ _ _ _ _ _ _ _ _ _ _ _ _ _ _ _ _ _ _ _ w3592 w3625] -> w1365
            tunnel: w1361 -> [_ _ _ _ _ _ _ _ _ _ _ _ _ _ _ _ _ _ _ _ w2371 w2400 w2423 w2454 w2475 w2499 w2524 w2546 w2572 _ _ _ _ w2670 w2698 w2726 w2752 _ _ _ _ w2855 w2884 _ _ _ _ _ _ _ _ _ _ _ _ _ _ _ _ _ _ _ _ _ _ _ _ _ _ _ _ _]
            tunnel: [_ _ _ _ _ _ _ _ _ _ _ _ _ _ _ _ _ _ _ w2342 w2371 w2399 w2422 w2453 w2474 w2499 w2524 w2546 w2572 _ _ _ _ w2670 w2698 w2726 w2752 _ _ _ _ w2855 w2884 _ _ _ _ _ _ _ _ _ _ _ _ _ _ _ _ _ _ _ _ _ _ _ _ _ _ _ _ _] -> w1360
            tunnel: [_ _ _ _ _ _ _ _ _ _ _ _ _ _ _ _ _ _ _ _ _ _ _ _ _ _ w2521 _ _ _ _ _ _ _ w2695 _ _ _ _ _ _ w2852 w2881 _ _ _ _ _ _ _ _ _ _ _ _ _ _ _ _ _ _ _ _ _ _ _ _ _ _ _ _ _] -> w1353
            tunnel: [_ _ _ _ _ _ _ _ _ _ _ _ _ _ _ _ _ _ _ _ _ _ _ _ _ _ w2520 _ _ _ _ _ _ _ w2694 _ _ _ _ _ _ w2851 w2880 _ _ _ _ _ _ _ _ _ _ _ _ _ _ _ _ _ _ _ _ _ _ _ _ _ _ _ _ _] -> w1351
            tunnel: [_ _ _ _ _ _ _ _ _ _ _ _ _ _ _ _ _ _ _ _ _ _ _ _ _ _ _ _ _ _ _ _ _ _ w2693 _ _ _ _ _ _ _ _ _ _ _ _ _ _ _ _ _ _ _ _ _ _ _ _ _ _ _ _ _ _ _ _ _ _ _ _ _] -> w1357
            frame "Start1", Default {
              w1479 = FALSE ("SelectionState")
              n850 = xnode "Read/Write Control"("FPGA VI Reference In"=w1481, "error in"=w1480, "SelectionState"=w1479, "LR_reward_Laser_l1"=w1479, "LR_wrong_Laser_l1"=w1479, "LR_reward_Event_l1"=w1479, "LR_wrong_Event_l1"=w1479, "Left(F)_or_Right(T)"=w1479, "ignoreWrong"=w1479, "SelectionState"=w1479, "LR_reward_Laser_l2"=w1479, "LR_wrong_laser_l2"=w1479, "LR_reward_Event_l2"=w1479, "LR_wrong_Event_l2"=w1479, "LC_Event_l1"=w1479, "LC_Laser_l1"=w1479, "LC_Laser_l2"=w1479, "LC_Event_l2"=w1479, "CueLed_Event"=w1479) -> ()  [unwired: 2 out]
            }
            frame "Start2" {
            }
            frame "Start3" {
            }
            frame "saveSettings1" {
              n851 = call "myRIO_BRig_RT_dataExp_Audio_freq__L.vi"() -> ("output_Audio_freq__L"=w1574:i32)  [unwired: 11 in]
              n852 = call "myRIO_BRig_RT_dataExp_Audio_freq__R.vi"() -> ("output_Audio_freq__R"=w1573:i32)  [unwired: 11 in]
              n853 = call "myRIO_BRig_RT_dataExp_Audio_amp__L.vi"() -> ("output_Audio_amp__L"=w1572:i32)  [unwired: 11 in]
              n854 = call "myRIO_BRig_RT_dataExp_Audio_amp__R.vi"() -> ("output_Audio_amp__R"=w1570:i32)  [unwired: 11 in]
              n855 = call "myRIO_BRig_RT_dataExp_TPB_min__L.vi"() -> ("output_TPB_min__L"=w1582:i32)  [unwired: 11 in]
              n856 = call "myRIO_BRig_RT_dataExp_TPB_min__R.vi"() -> ("output_TPB_min__R"=w1580:i32)  [unwired: 11 in]
              n857 = call "myRIO_BRig_RT_dataExp_TPB_max__L.vi"() -> ("output_TPB_max__L"=w1578:i32)  [unwired: 11 in]
              n858 = call "myRIO_BRig_RT_dataExp_TPB_max__R.vi"() -> ("output_TPB_max__R"=w1576:i32)  [unwired: 11 in]
              n859 = call "myRIO_BRig_RT_dataExp_Cue1Param_AudioLed_Count_Switch.vi"() -> ("output_Cue1Param_AudioLed_Count_Switch"=w1544:i32)  [unwired: 11 in]
              n860 = call "myRIO_BRig_RT_dataExp_Cue1Param_AudioLed_Probability_Switch.vi"() -> ("output_Cue1Param_AudioLed_Probability_Switch"=w1542:i32)  [unwired: 11 in]
              n861 = call "myRIO_BRig_RT_dataExp_Cue1Param_CueType_Switch.vi"() -> ("output_Cue1Param_CueType_Switch"=w1540:i32)  [unwired: 11 in]
              n862 = call "myRIO_BRig_RT_dataExp_ItrialUntilReward.vi"() -> ("output_I_trialUntilReward"=w1595:i32)  [unwired: 11 in]
              n863 = call "myRIO_BRig_RT_dataExp_IblockUntilReward.vi"() -> ("output_I_blockUntilReward"=w1591:i32)  [unwired: 11 in]
              n864 = call "myRIO_BRig_RT_dataExp_CueCycles.vi"() -> ("output_CueCycles"=w1590:i32)  [unwired: 11 in]
              n865 = call "myRIO_BRig_RT_dataExp_ENL_min.vi"() -> ("output_ENL_min"=w1588:i32)  [unwired: 11 in]
              n866 = call "myRIO_BRig_RT_dataExp_ENL_max.vi"() -> ("output_ENL_max"=w1586:i32)  [unwired: 11 in]
              n867 = call "myRIO_BRig_RT_dataExp_ENL_penalty.vi"() -> ("output_ENL_penalty"=w1584:i32)  [unwired: 11 in]
              n868 = local read "Audio_Freq__L"() -> (w1548:u8)
              n869 = local read "Audio_Freq__R"() -> (w1546:u8)
              n870 = local read "Audio_Amp__L"() -> (w1571:u16)
              n871 = local read "TpB_Min_L"() -> (w1581:u16)
              n872 = local read "TpB_Min_R"() -> (w1579:u16)
              n873 = local read "TpB_Max_L"() -> (w1577:u16)
              n874 = local read "TpB_Max_R"() -> (w1575:u16)
              n875 = local read "Audio_Amp__R"() -> (w1569:u16)
              n876 = local read "TrialUntilReward"() -> (w1594:bool)
              n877 = local read "CueCycles"() -> (w1589:u16)
              n878 = local read "Tcycle_ENL_min"() -> (w1587:u16)
              n879 = local read "Tcycle_ENL_max"() -> (w1585:u16)
              n880 = local read "Tcycle_ENLPenalty"() -> (w1583:u16)
              n881 = local read "Cue1Param_AudioLed_Count_Switch"() -> (w1543:u16)
              n882 = local read "Cue1Param_AudioLed_Probability_Switch"() -> (w1541:u16)
              n883 = local read "Cue1Param_CueType_Switch"() -> (w1539:u16)
              n884 = To Unsigned Word Integer(number=w1546) -> (unsigned 16bit integer=w1545:u16)
              n885 = To Unsigned Word Integer(number=w1548) -> (unsigned 16bit integer=w1547:u16)
              n886 = Boolean To (0,1)(Boolean=w1594) -> (0, 1=w1593:i16)
              n887 = To Unsigned Word Integer(number=w1593) -> (unsigned 16bit integer=w1592:u16)
              n888 = local read "BUR_min"() -> (w1563:u16)
              n889 = local read "BUR_max"() -> (w1564:u16)
              n890 = Not Equal To 0?(x=w1563) -> (x != 0?=w1562:bool)
              n891 = Not Equal To 0?(x=w1564) -> (x != 0?=w1561:bool)
              n892 = And(x=w1562, y=w1561) -> (x .and. y?=w1560:bool)
              n893 = Boolean To (0,1)(Boolean=w1560) -> (0, 1=w1565:i16)
              n894 = To Unsigned Word Integer(number=w1565) -> (unsigned 16bit integer=w1559:u16)
              n895 = Replace Array Subset(array=w1597, new element #1=w1592, index #1=w1595, new element #2=w1559, index #2=w1591, new element #3=w1589, index #3=w1590, new element #4=w1587, index #4=w1588, new element #5=w1585, index #5=w1586, new element #6=w1583, index #6=w1584, new element #7=w1581, index #7=w1582, new element #8=w1579, index #8=w1580, new element #9=w1577, index #9=w1578, new element #10=w1575, index #10=w1576, new element #11=w1547, index #11=w1574, new element #12=w1545, index #12=w1573, new element #13=w1571, index #13=w1572, new element #14=w1569, index #14=w1570, new element #15=w1543, index #15=w1544, new element #16=w1541, index #16=w1542, new element #17=w1539, index #17=w1540) -> (w1596:u16[])
            }
            frame "saveSettings2" {
              n896 = call "myRIO_BRig_RT_dataExp_Tcycle_RewardPost.vi"() -> ("output_Tcycle_RewardPost"=w1640:i32)  [unwired: 11 in]
              n897 = call "myRIO_BRig_RT_dataExp_Tcycle_Wrong.vi"() -> ("output_Tcycle_Wrong"=w1638:i32)  [unwired: 11 in]
              n898 = call "myRIO_BRig_RT_dataExp_Tcycle_Timeout.vi"() -> ("output_Tcycle_Timeout"=w1636:i32)  [unwired: 11 in]
              n899 = call "myRIO_BRig_RT_dataExp_Tcycle_Cue1_Audio_min.vi"() -> ("output_Tcycle_Cue1_Audio_min"=w1634:i32)  [unwired: 11 in]
              n900 = call "myRIO_BRig_RT_dataExp_Tcycle_Cue1_Audio_max.vi"() -> ("output_Tcycle_Cue1_Audio_max"=w1633:i32)  [unwired: 11 in]
              n901 = call "myRIO_BRig_RT_dataExp_Tcycle_Cue1Penalty_Audio.vi"() -> ("output_Tcycle_Cue1Penalty_Audio"=w1632:i32)  [unwired: 11 in]
              n902 = call "myRIO_BRig_RT_dataExp_SolenoidProbability_L.vi"() -> ("output_SolenoidProbability_L"=w1612:i32)  [unwired: 11 in]
              n903 = call "myRIO_BRig_RT_dataExp_SolenoidProbability_R.vi"() -> ("output_SolenoidProbability_R"=w1611:i32)  [unwired: 11 in]
              n904 = call "myRIO_BRig_RT_dataExp_nBlock.vi"() -> ("output_nBlock"=w1649:i32)  [unwired: 11 in]
              n905 = call "myRIO_BRig_RT_dataExp_nTrial.vi"() -> ("output_nTrial"=w1648:i32)  [unwired: 11 in]
              n906 = call "myRIO_BRig_RT_dataExp_runTime_seconds.vi"() -> ("output_RunTime_minutes"=w1647:i32)  [unwired: 11 in]
              n907 = call "myRIO_BRig_RT_dataExp_Tcycle_Selection.vi"() -> ("output_Tcycle_Selection"=w1646:i32)  [unwired: 11 in]
              n908 = call "myRIO_BRig_RT_dataExp_Tcycle_Reward__L.vi"() -> ("output_Tcycle_Reward__L"=w1644:i32)  [unwired: 11 in]
              n909 = call "myRIO_BRig_RT_dataExp_Tcycle_Reward__R.vi"() -> ("output_Tcycle_Reward__R"=w1642:i32)  [unwired: 11 in]
              n910 = local read "Tcycle_RewardPost"() -> (w1639:u16)
              n911 = local read "Tcycle_Wrong"() -> (w1637:u16)
              n912 = local read "Tcycle_Timeout"() -> (w1635:u16)
              n913 = call "myRIO_BRig_RT_dataExp_Cue1Param_AudioLed_Count_NS.vi"() -> ("output_Cue1Param_AudioLed_Count_NS"=w1608:i32)  [unwired: 11 in]
              n914 = call "myRIO_BRig_RT_dataExp_Cue1Param_AudioLed_Probability_NS.vi"() -> ("output_Cue1Param_AudioLed_Probability_NS"=w1606:i32)  [unwired: 11 in]
              n915 = call "myRIO_BRig_RT_dataExp_Cue1Param_CueType_NS.vi"() -> ("output_Cue1Param_CueType_NS"=w1604:i32)  [unwired: 11 in]
              n916 = local read "Tcycle_CuePenalty"() -> (w1625:u16)
              n917 = local read "Tcycle_Cue_max"() -> (w1613:u16)
              n918 = local read "Tcycle_Cue_min"() -> (w1614:u16)
              n919 = local read "Tcycle_Selection"() -> (w1645:u16)
              n920 = local read "Tcycle_Reward_L"() -> (w1643:u16)
              n921 = local read "Tcycle_Reward_R"() -> (w1641:u16)
              n922 = local read "SolenoidProbability_R"() -> (w1609:u16)
              n923 = local read "SolenoidProbability_L"() -> (w1610:u16)
              n924 = local read "Cue1Param_AudioLed_Count_NS"() -> (w1607:u16)
              n925 = local read "Cue1Param_AudioLed_Probability_NS"() -> (w1605:u16)
              n926 = local read "Cue1Param_CueType_NS"() -> (w1603:u16)
              n927 = Replace Array Subset(array=w1651, new element #1=u16 0, index #1=w1649, new element #2=u16 0, index #2=w1648, new element #3=u16 0, index #3=w1647, new element #4=w1645, index #4=w1646, new element #5=w1643, index #5=w1644, new element #6=w1641, index #6=w1642, new element #7=w1639, index #7=w1640, new element #8=w1637, index #8=w1638, new element #9=w1635, index #9=w1636, new element #10=w1614, index #10=w1634, new element #11=w1613, index #11=w1633, new element #12=w1625, index #12=w1632, new element #13=w1610, index #13=w1612, new element #14=w1609, index #14=w1611, new element #15=w1607, index #15=w1608, new element #16=w1605, index #16=w1606, new element #17=w1603, index #17=w1604) -> (w1650:u16[])
            }
            frame "saveSettings3" {
              w1662 = 100.0 ("y")
              n928 = call "myRIO_BRig_RT_dataExp_laser1_Freq.vi"() -> ("output_laser1_Freq"=w1695:i32)  [unwired: 11 in]
              n929 = call "myRIO_BRig_RT_dataExp_laser1_Tpeak.vi"() -> ("output_laser1_Tpeak"=w1690:i32)  [unwired: 11 in]
              n930 = call "myRIO_BRig_RT_dataExp_laser1_Tshutter.vi"() -> ("output_laser1_Tshutter"=w1685:i32)  [unwired: 11 in]
              n931 = call "myRIO_BRig_RT_dataExp_FPGA_f_count2ms.vi"() -> ("output_FPGA_f_count2ms"=w1680:i32)  [unwired: 11 in]
              n932 = call "myRIO_BRig_RT_dataExp_laser1_Power_min.vi"() -> ("output_laser1_Power_min"=w1675:i32)  [unwired: 11 in]
              n933 = call "myRIO_BRig_RT_dataExp_laser1_Power_max.vi"() -> ("output_laser1_Power_max"=w1668:i32)  [unwired: 11 in]
              n934 = call "myRIO_BRig_RT_dataExp_laser1_Power_step.vi"() -> ("output_laser1_Power_step"=w1667:i32)  [unwired: 11 in]
              n935 = call "myRIO_BRig_RT_dataExp_laser1_duration.vi"() -> ("output_laser1_duration"=w1670:i32)  [unwired: 11 in]
              n936 = local read "Laser_Tshutter_l1"() -> (w1682:dbl)
              n937 = local read "Laser_Tpeak_l1"() -> (w1687:dbl)
              n938 = local read "Laser_power_max_l1"() -> (w1661:dbl)
              n939 = local read "Laser_power_step_l1"() -> (w1660:dbl)
              n940 = local read "Laser_power_min_l1"() -> (w1672:dbl)
              n941 = local read "Laser_Freq_l1"() -> (w1694:dbl)
              n942 = call "myRIO_BRig_RT_dataExp_BUR_min.vi"() -> ("output_BUR_min"=w1717:i32)  [unwired: 11 in]
              n943 = call "myRIO_BRig_RT_dataExp_BUR_max.vi"() -> ("output_BUR_max"=w1715:i32)  [unwired: 11 in]
              n944 = call "myRIO_BRig_RT_dataExp_Audio_sp__L.vi"() -> ("output_Audio_sp__L"=w1712:i32)  [unwired: 11 in]
              n945 = call "myRIO_BRig_RT_dataExp_Audio_sp__R.vi"() -> ("output_Audio_sp__R"=w1711:i32)  [unwired: 11 in]
              n946 = local read "FPGA_count2ms"() -> (w1677:dbl)
              n947 = local read "sp_LeftSpout"() -> (w1710:u16)
              n948 = local read "BUR_max"() -> (w1714:u16)
              n949 = local read "sp_RightSpout"() -> (w1709:u16)
              n950 = local read "BUR_min"() -> (w1716:u16)
              n951 = Multiply(x=w1694, y=w1662) -> (x*y=w1693:dbl)
              n952 = Multiply(x=w1687, y=w1662) -> (x*y=w1689:dbl)
              n953 = Multiply(x=w1682, y=w1662) -> (x*y=w1684:dbl)
              n954 = Multiply(x=w1677, y=w1662) -> (x*y=w1679:dbl)
              n955 = Multiply(x=w1672, y=w1662) -> (x*y=w1674:dbl)
              n956 = Multiply(x=w1661, y=w1662) -> (x*y=w1666:dbl)
              n957 = Multiply(x=w1660, y=w1662) -> (x*y=w1664:dbl)
              n958 = Round To Nearest(number=w1693) -> (nearest integer value=w1692:dbl)
              n959 = Round To Nearest(number=w1689) -> (nearest integer value=w1688:dbl)
              n960 = Round To Nearest(number=w1684) -> (nearest integer value=w1683:dbl)
              n961 = Round To Nearest(number=w1679) -> (nearest integer value=w1678:dbl)
              n962 = Round To Nearest(number=w1674) -> (nearest integer value=w1673:dbl)
              n963 = Round To Nearest(number=w1666) -> (nearest integer value=w1665:dbl)
              n964 = Round To Nearest(number=w1664) -> (nearest integer value=w1663:dbl)
              n965 = To Unsigned Word Integer(number=w1692) -> (unsigned 16bit integer=w1691:u16)
              n966 = To Unsigned Word Integer(number=w1688) -> (unsigned 16bit integer=w1686:u16)
              n967 = To Unsigned Word Integer(number=w1683) -> (unsigned 16bit integer=w1681:u16)
              n968 = To Unsigned Word Integer(number=w1678) -> (unsigned 16bit integer=w1676:u16)
              n969 = To Unsigned Word Integer(number=w1673) -> (unsigned 16bit integer=w1671:u16)
              n970 = To Unsigned Word Integer(number=w1665) -> (unsigned 16bit integer=w1659:u16)
              n971 = To Unsigned Word Integer(number=w1663) -> (unsigned 16bit integer=w1658:u16)
              n972 = local read "Laser_duration_l1"() -> (w1669:u16)
              n973 = call "myRIO_BRig_RT_dataCurrent_laser1_pulse_duration.vi"() -> ("output_laser1_pulse_duration"=w1696:i32)  [unwired: 11 in]
              n974 = Replace Array Subset(array=w1718, new element #1=w1716, index #1=w1717, new element #2=w1714, index #2=w1715, new element #3=w1710, index #3=w1712, new element #4=w1709, index #4=w1711, new element #5=w1691, index #5=w1695, new element #6=w1686, index #6=w1690, new element #7=w1681, index #7=w1685, new element #8=w1676, index #8=w1680, new element #9=w1671, index #9=w1675, new element #10=w1659, index #10=w1668, new element #11=w1658, index #11=w1667, new element #12=w1669, index #12=w1670) -> (w1713:u16[])
              n975 = Replace Array Subset(array=w1698, new element=w1669, index=w1696) -> (w1697:u16[])
            }
            frame "saveSettings4" {
              w1739 = 100.0 ("y")
              n976 = call "myRIO_BRig_RT_dataExp_laser2_Freq.vi"() -> ("output_laser2_Freq"=w1726:i32)  [unwired: 11 in]
              n977 = call "myRIO_BRig_RT_dataExp_laser2_Tpeak.vi"() -> ("output_laser2_Tpeak"=w1728:i32)  [unwired: 11 in]
              n978 = call "myRIO_BRig_RT_dataExp_laser2_Tshutter.vi"() -> ("output_laser2_Tshutter"=w1730:i32)  [unwired: 11 in]
              n979 = call "myRIO_BRig_RT_dataExp_laser2_Power_min.vi"() -> ("output_laser2_Power_min"=w1747:i32)  [unwired: 11 in]
              n980 = call "myRIO_BRig_RT_dataExp_laser2_Power_max.vi"() -> ("output_laser2_Power_max"=w1746:i32)  [unwired: 11 in]
              n981 = call "myRIO_BRig_RT_dataExp_laser2_Power_step.vi"() -> ("output_laser2_Power_step"=w1745:i32)  [unwired: 11 in]
              n982 = call "myRIO_BRig_RT_dataExp_laser2_duration.vi"() -> ("output_laser2_duration"=w1744:i32)  [unwired: 11 in]
              n983 = call "myRIO_BRig_RT_dataExp_CueLed_Freq.vi"() -> ("output_CueLed_Freq"=w1736:i32)  [unwired: 11 in]
              n984 = call "myRIO_BRig_RT_dataExp_CueLed_Tpeak.vi"() -> ("output_CueLed_Tpeak"=w1735:i32)  [unwired: 11 in]
              n985 = call "myRIO_BRig_RT_dataExp_CueLed.vi"() -> ("output_CueLed"=w1732:i32)  [unwired: 11 in]
              n986 = local read "Laser_Tshutter_l2"() -> (w1763:dbl)
              n987 = local read "Laser_Tpeak_l2"() -> (w1766:dbl)
              n988 = local read "Laser_power_max_l2"() -> (w1753:dbl)
              n989 = local read "Laser_power_step_l2"() -> (w1752:dbl)
              n990 = local read "Laser_power_min_l2"() -> (w1760:dbl)
              n991 = local read "Laser_Freq_l2"() -> (w1771:dbl)
              n992 = local read "CueLed_Tpeak"() -> (w1737:dbl)
              n993 = local read "CueLed_duration"() -> (w1731:u16)
              n994 = local read "CueLed_Freq"() -> (w1738:dbl)
              n995 = Multiply(x=w1771, y=w1739) -> (x*y=w1770:dbl)
              n996 = Multiply(x=w1766, y=w1739) -> (x*y=w1768:dbl)
              n997 = Multiply(x=w1763, y=w1739) -> (x*y=w1765:dbl)
              n998 = Multiply(x=w1760, y=w1739) -> (x*y=w1762:dbl)
              n999 = Multiply(x=w1753, y=w1739) -> (x*y=w1757:dbl)
              n1000 = Multiply(x=w1752, y=w1739) -> (x*y=w1755:dbl)
              n1001 = Multiply(x=w1738, y=w1739) -> (x*y=w1740:dbl)
              n1002 = Multiply(x=w1737, y=w1739) -> (x*y=w1741:dbl)
              n1003 = Round To Nearest(number=w1770) -> (nearest integer value=w1769:dbl)
              n1004 = Round To Nearest(number=w1768) -> (nearest integer value=w1767:dbl)
              n1005 = Round To Nearest(number=w1765) -> (nearest integer value=w1764:dbl)
              n1006 = Round To Nearest(number=w1762) -> (nearest integer value=w1761:dbl)
              n1007 = Round To Nearest(number=w1757) -> (nearest integer value=w1756:dbl)
              n1008 = Round To Nearest(number=w1755) -> (nearest integer value=w1754:dbl)
              n1009 = Round To Nearest(number=w1740) -> (nearest integer value=w1743:dbl)
              n1010 = Round To Nearest(number=w1741) -> (nearest integer value=w1742:dbl)
              n1011 = To Unsigned Word Integer(number=w1769) -> (unsigned 16bit integer=w1725:u16)
              n1012 = To Unsigned Word Integer(number=w1767) -> (unsigned 16bit integer=w1727:u16)
              n1013 = To Unsigned Word Integer(number=w1764) -> (unsigned 16bit integer=w1729:u16)
              n1014 = To Unsigned Word Integer(number=w1761) -> (unsigned 16bit integer=w1759:u16)
              n1015 = To Unsigned Word Integer(number=w1756) -> (unsigned 16bit integer=w1751:u16)
              n1016 = To Unsigned Word Integer(number=w1754) -> (unsigned 16bit integer=w1750:u16)
              n1017 = To Unsigned Word Integer(number=w1743) -> (unsigned 16bit integer=w1734:u16)
              n1018 = To Unsigned Word Integer(number=w1742) -> (unsigned 16bit integer=w1733:u16)
              n1019 = local read "Laser_duration_l2"() -> (w1758:u16)
              n1020 = call "myRIO_BRig_RT_dataCurrent_laser2_pulse_duration.vi"() -> ("output_laser2_pulse_duration"=w1748:i32)  [unwired: 11 in]
              n1021 = Replace Array Subset(array=w1773, new element=w1758, index=w1748) -> (w1772:u16[])
              n1022 = Replace Array Subset(array=w1785, new element #1=w1725, index #1=w1726, new element #2=w1727, index #2=w1728, new element #3=w1729, index #3=w1730, new element #4=w1759, index #4=w1747, new element #5=w1751, index #5=w1746, new element #6=w1750, index #6=w1745, new element #7=w1758, index #7=w1744, new element #8=w1734, index #8=w1736, new element #9=w1733, index #9=w1735, new element #10=w1731, index #10=w1732) -> (w1784:u16[])
            }
            frame "saveSettings_LC_ENL_l1" {
              # "Selection First"
              # "Count"
              # "Tdelay"
              # "Probability"
              # "OnOff"
              # "Block"
              # "delayOpt"
              # "Count"
              # "Tdelay"
              # "Probability"
              # "OnOff"
              # "Block"
              # "ENL1 All"
              # "delayOpt"
              # "Count"
              # "Tdelay"
              # "Probability"
              # "OnOff"
              # "Block"
              # "ENL1 First"
              n1023 = local read "LC_ENL1_delayOpt_Switch_l1"() -> (w1823:bool)
              n1024 = call "myRIO_BRig_RT_dataLC_ENL1_Block_NS_l1.vi"() -> ("output_ENL1_All_Block"=w1820:i32)  [unwired: 11 in]
              n1025 = call "myRIO_BRig_RT_dataLC_ENL1_OnOff_NS_l1.vi"() -> ("output_ENL1_OnOff_NS_l1"=w1810:i32)  [unwired: 11 in]
              n1026 = call "myRIO_BRig_RT_dataLC_ENL1_Probability_NS_l1.vi"() -> ("output_ENL1_Probability_NS_l1"=w1809:i32)  [unwired: 11 in]
              n1027 = call "myRIO_BRig_RT_dataLC_ENL1_Tdelay_NS_l1.vi"() -> ("output_ENL1_Tdelay_NS_l1"=w1808:i32)  [unwired: 11 in]
              n1028 = call "myRIO_BRig_RT_dataLC_ENL1_Count_NS_l1.vi"() -> ("output_ENL1_Count_NS_l1"=w1807:i32)  [unwired: 11 in]
              n1029 = call "myRIO_BRig_RT_dataLC_ENL1_delayOpt_NS_l1.vi"() -> ("output_ENL1_delayOpt_NS_l1"=w1806:i32)  [unwired: 11 in]
              n1030 = call "myRIO_BRig_RT_dataLC_ENL1_Block_Switch_l1.vi"() -> ("output_ENL1_Block_Switch_l1"=w1846:i32)  [unwired: 11 in]
              n1031 = call "myRIO_BRig_RT_dataLC_ENL1_OnOff_Switch_l1.vi"() -> ("output_ENL1_OnOff_Switch_l1"=w1844:i32)  [unwired: 11 in]
              n1032 = call "myRIO_BRig_RT_dataLC_ENL1_Probability_Switch_l1.vi"() -> ("output_ENL1_Probability_Switch_l1"=w1840:i32)  [unwired: 11 in]
              n1033 = call "myRIO_BRig_RT_dataLC_ENL1_Tdelay_Switch_l1.vi"() -> ("output_ENL1_Tdelay_Switch_l1"=w1838:i32)  [unwired: 11 in]
              n1034 = call "myRIO_BRig_RT_dataLC_ENL1_Count_Switch_l1.vi"() -> ("output_ENL1_Count_Switch_l1"=w1836:i32)  [unwired: 11 in]
              n1035 = call "myRIO_BRig_RT_dataLC_ENL1_delayOpt_Switch_l1.vi"() -> ("output_ENL1_delayOpt_Switch_l1"=w1822:i32)  [unwired: 11 in]
              n1036 = local read "LC_ENL1_Count_Switch_l1"() -> (w1835:u16)
              n1037 = local read "LC_ENL1_Probability_Switch_l1"() -> (w1839:u16)
              n1038 = local read "LC_ENL1_Block_Switch_l1"() -> (w1845:u16)
              n1039 = local read "LC_ENL1_Tdelay_Switch_l1"() -> (w1837:u16)
              n1040 = local read "LC_ENL1_OnOff_Switch_l1"() -> (w1843:bool)
              n1041 = call "myRIO_BRig_RT_dataLC_Selection_Block_Switch_l1.vi"() -> ("output_Selection_Block_Switch_l1"=w1804:i32)  [unwired: 11 in]
              n1042 = call "myRIO_BRig_RT_dataLC_Selection_OnOff_Switch_l1.vi"() -> ("output_Selection_OnOff_Switch_l1"=w1803:i32)  [unwired: 11 in]
              n1043 = call "myRIO_BRig_RT_dataLC_Selection_Probability_Switch_l1.vi"() -> ("output_Selection_Probability_Switch_l1"=w1802:i32)  [unwired: 11 in]
              n1044 = call "myRIO_BRig_RT_dataLC_Selection_Tdelay_Switch_l1.vi"() -> ("output_Selection_Tdelay_Switch_l1"=w1801:i32)  [unwired: 11 in]
              n1045 = call "myRIO_BRig_RT_dataLC_Selection_Count_Switch_l1.vi"() -> ("output_Selection_Count_Switch_l1"=w1800:i32)  [unwired: 11 in]
              n1046 = local read "LC_ENL1_OnOff_NS_l1"() -> (w1816:bool)
              n1047 = local read "LC_ENL1_Probability_NS_l1"() -> (w1814:u16)
              n1048 = local read "LC_ENL1_delayOpt_NS_l1"() -> (w1812:bool)
              n1049 = local read "LC_Sel_Probability_Switch_l1"() -> (w1795:u16)
              n1050 = local read "LC_ENL1_Tdelay_NS_l1"() -> (w1805:u16)
              n1051 = local read "LC_ENL1_Block_NS_l1"() -> (w1817:u16)
              n1052 = local read "LC_ENL1_Count_NS_l1"() -> (w1813:u16)
              n1053 = local read "LC_Sel_Tdelay_Switch_l1"() -> (w1794:u16)
              n1054 = local read "LC_Sel_OnOff_Switch_l1"() -> (w1798:bool)
              n1055 = local read "LC_Sel_Count_Switch_l1"() -> (w1793:u16)
              n1056 = local read "LC_Sel_Block_Switch_l1"() -> (w1797:u16)
              n1057 = Boolean To (0,1)(Boolean=w1823) -> (0, 1=w1824:i16)
              n1058 = Boolean To (0,1)(Boolean=w1843) -> (0, 1=w1842:i16)
              n1059 = Boolean To (0,1)(Boolean=w1816) -> (0, 1=w1819:i16)
              n1060 = To Unsigned Word Integer(number=w1824) -> (unsigned 16bit integer=w1821:u16)
              n1061 = To Unsigned Word Integer(number=w1842) -> (unsigned 16bit integer=w1841:u16)
              n1062 = Boolean To (0,1)(Boolean=w1812) -> (0, 1=w1818:i16)
              n1063 = To Unsigned Word Integer(number=w1819) -> (unsigned 16bit integer=w1815:u16)
              n1064 = Boolean To (0,1)(Boolean=w1798) -> (0, 1=w1799:i16)
              n1065 = To Unsigned Word Integer(number=w1818) -> (unsigned 16bit integer=w1811:u16)
              n1066 = To Unsigned Word Integer(number=w1799) -> (unsigned 16bit integer=w1796:u16)
              n1067 = Replace Array Subset(array=w1847, new element #1=w1845, index #1=w1846, new element #2=w1841, index #2=w1844, new element #3=w1839, index #3=w1840, new element #4=w1837, index #4=w1838, new element #5=w1835, index #5=w1836, new element #6=w1821, index #6=w1822, new element #7=w1817, index #7=w1820, new element #8=w1815, index #8=w1810, new element #9=w1814, index #9=w1809, new element #10=w1805, index #10=w1808, new element #11=w1813, index #11=w1807, new element #12=w1811, index #12=w1806, new element #13=w1797, index #13=w1804, new element #14=w1796, index #14=w1803, new element #15=w1795, index #15=w1802, new element #16=w1794, index #16=w1801, new element #17=w1793, index #17=w1800) -> (w1848:u16[])
            }
            frame "saveSettings_LC_ENL_l2" {
              # "Selection First"
              # "Count"
              # "Tdelay"
              # "Probability"
              # "OnOff"
              # "Block"
              # "delayOpt"
              # "Count"
              # "Tdelay"
              # "Probability"
              # "OnOff"
              # "Block"
              # "ENL1 All"
              # "delayOpt"
              # "Count"
              # "Tdelay"
              # "Probability"
              # "OnOff"
              # "Block"
              # "ENL1 First"
              n1068 = call "myRIO_BRig_RT_dataLC_ENL1_Block_Switch_l2.vi"() -> ("output_ENL1_Block_Switch_l2"=w1867:i32)  [unwired: 11 in]
              n1069 = call "myRIO_BRig_RT_dataLC_ENL1_OnOff_Switch_l2.vi"() -> ("output_ENL1_OnOff_Switch_l2"=w1868:i32)  [unwired: 11 in]
              n1070 = call "myRIO_BRig_RT_dataLC_ENL1_Probability_Switch_l2.vi"() -> ("output_ENL1_Probability_Switch_l2"=w1869:i32)  [unwired: 11 in]
              n1071 = call "myRIO_BRig_RT_dataLC_ENL1_Tdelay_Switch_l2.vi"() -> ("output_ENL1_Tdelay_Switch_l2"=w1870:i32)  [unwired: 11 in]
              n1072 = call "myRIO_BRig_RT_dataLC_ENL1_Count_Switch_l2.vi"() -> ("output_ENL1_Count_Switch_l2"=w1871:i32)  [unwired: 11 in]
              n1073 = call "myRIO_BRig_RT_dataLC_ENL1_delayOpt_Switch_l2.vi"() -> ("output_ENL1_delayOpt_Switch_l2"=w1872:i32)  [unwired: 11 in]
              n1074 = local read "LC_ENL1_delayOpt_Switch_l2"() -> (w1892:bool)
              n1075 = call "myRIO_BRig_RT_dataLC_ENL1_Block_NS_l2.vi"() -> ("output_ENL1_Block_NS_l2"=w1861:i32)  [unwired: 11 in]
              n1076 = call "myRIO_BRig_RT_dataLC_ENL1_OnOff_NS_l2.vi"() -> ("output_ENL1_OnOff_NS_l2"=w1862:i32)  [unwired: 11 in]
              n1077 = call "myRIO_BRig_RT_dataLC_ENL1_Probability_NS_l2.vi"() -> ("output_ENL1_Probability_NS_l2"=w1863:i32)  [unwired: 11 in]
              n1078 = call "myRIO_BRig_RT_dataLC_ENL1_Tdelay_NS_l2.vi"() -> ("output_ENL1_Tdelay_NS_l2"=w1864:i32)  [unwired: 11 in]
              n1079 = call "myRIO_BRig_RT_dataLC_ENL1_Count_NS_l2.vi"() -> ("output_ENL1_Count_NS_l2"=w1865:i32)  [unwired: 11 in]
              n1080 = call "myRIO_BRig_RT_dataLC_ENL1_delayOpt_NS_l2.vi"() -> ("output_ENL1_delayOpt_NS_l2"=w1866:i32)  [unwired: 11 in]
              n1081 = local read "LC_ENL1_Count_Switch_l2"() -> (w1904:u16)
              n1082 = local read "LC_ENL1_Probability_Switch_l2"() -> (w1906:u16)
              n1083 = local read "LC_ENL1_Block_Switch_l2"() -> (w1910:u16)
              n1084 = local read "LC_ENL1_Tdelay_Switch_l2"() -> (w1905:u16)
              n1085 = local read "LC_ENL1_OnOff_Switch_l2"() -> (w1909:bool)
              n1086 = call "myRIO_BRig_RT_dataLC_Selection_Block_Switch_l2.vi"() -> ("output_Selection_Block_Switch_l2"=w1860:i32)  [unwired: 11 in]
              n1087 = call "myRIO_BRig_RT_dataLC_Selection_OnOff_Switch_l2.vi"() -> ("output_Selection_OnOff_Switch_l2"=w1859:i32)  [unwired: 11 in]
              n1088 = call "myRIO_BRig_RT_dataLC_Selection_Probability_Switch_l2.vi"() -> ("output_Selection_Probability_Switch_l1"=w1858:i32)  [unwired: 11 in]
              n1089 = call "myRIO_BRig_RT_dataLC_Selection_Tdelay_Switch_l2.vi"() -> ("output_Selection_Tdelay_Switch_l2"=w1857:i32)  [unwired: 11 in]
              n1090 = call "myRIO_BRig_RT_dataLC_Selection_Count_Switch_l2.vi"() -> ("output_Selection_Count_Switch_l2"=w1856:i32)  [unwired: 11 in]
              n1091 = local read "LC_ENL1_OnOff_NS_l2"() -> (w1887:bool)
              n1092 = local read "LC_ENL1_Probability_NS_l2"() -> (w1885:u16)
              n1093 = local read "LC_ENL1_delayOpt_NS_l2"() -> (w1883:bool)
              n1094 = local read "LC_Sel_Probability_Switch_l2"() -> (w1876:u16)
              n1095 = local read "LC_ENL1_Tdelay_NS_l2"() -> (w1881:u16)
              n1096 = local read "LC_ENL1_Block_NS_l2"() -> (w1888:u16)
              n1097 = local read "LC_ENL1_Count_NS_l2"() -> (w1884:u16)
              n1098 = local read "LC_Sel_Tdelay_Switch_l2"() -> (w1875:u16)
              n1099 = local read "LC_Sel_OnOff_Switch_l2"() -> (w1879:bool)
              n1100 = local read "LC_Sel_Count_Switch_l2"() -> (w1874:u16)
              n1101 = local read "LC_Sel_Block_Switch_l2"() -> (w1878:u16)
              n1102 = Boolean To (0,1)(Boolean=w1892) -> (0, 1=w1893:i16)
              n1103 = Boolean To (0,1)(Boolean=w1909) -> (0, 1=w1908:i16)
              n1104 = Boolean To (0,1)(Boolean=w1887) -> (0, 1=w1890:i16)
              n1105 = To Unsigned Word Integer(number=w1893) -> (unsigned 16bit integer=w1891:u16)
              n1106 = To Unsigned Word Integer(number=w1908) -> (unsigned 16bit integer=w1907:u16)
              n1107 = Boolean To (0,1)(Boolean=w1883) -> (0, 1=w1889:i16)
              n1108 = To Unsigned Word Integer(number=w1890) -> (unsigned 16bit integer=w1886:u16)
              n1109 = Boolean To (0,1)(Boolean=w1879) -> (0, 1=w1880:i16)
              n1110 = To Unsigned Word Integer(number=w1889) -> (unsigned 16bit integer=w1882:u16)
              n1111 = To Unsigned Word Integer(number=w1880) -> (unsigned 16bit integer=w1877:u16)
              n1112 = Replace Array Subset(array=w1911, new element #1=w1910, index #1=w1867, new element #2=w1907, index #2=w1868, new element #3=w1906, index #3=w1869, new element #4=w1905, index #4=w1870, new element #5=w1904, index #5=w1871, new element #6=w1891, index #6=w1872, new element #7=w1888, index #7=w1861, new element #8=w1886, index #8=w1862, new element #9=w1885, index #9=w1863, new element #10=w1881, index #10=w1864, new element #11=w1884, index #11=w1865, new element #12=w1882, index #12=w1866, new element #13=w1878, index #13=w1860, new element #14=w1877, index #14=w1859, new element #15=w1876, index #15=w1858, new element #16=w1875, index #16=w1857, new element #17=w1874, index #17=w1856) -> (w1912:u16[])
            }
            frame "saveSettings_LC_Cue_l1" {
              # "Selection All"
              # "Count"
              # "Tdelay"
              # "Probability"
              # "OnOff"
              # "Block"
              # "delayOpt"
              # "Count"
              # "Tdelay"
              # "Probability"
              # "OnOff"
              # "Block"
              # "Cue1 All"
              # "delayOpt"
              # "Count"
              # "Tdelay"
              # "Probability"
              # "OnOff"
              # "Block"
              # "Cue1 First"
              n1113 = call "myRIO_BRig_RT_dataLC_Cue1_delayOpt_Switch_l1.vi"() -> ("output_Cue1_delayOpt_Switch_l1"=w1951:i32)  [unwired: 11 in]
              n1114 = call "myRIO_BRig_RT_dataLC_Cue1_Block_Switch_l1.vi"() -> ("output_Cue1_Block_Switch_l1"=w1974:i32)  [unwired: 11 in]
              n1115 = call "myRIO_BRig_RT_dataLC_Cue1_OnOff_Switch_l1.vi"() -> ("output_Cue1_OnOff_Switch_l1"=w1972:i32)  [unwired: 11 in]
              n1116 = call "myRIO_BRig_RT_dataLC_Cue1_Probability_Switch_l1.vi"() -> ("output_Cue1_Probability_Switch_l1"=w1968:i32)  [unwired: 11 in]
              n1117 = call "myRIO_BRig_RT_dataLC_Cue1_Tdelay_Switch_l1.vi"() -> ("output_Cue1_Tdelay_Switch_l1"=w1966:i32)  [unwired: 11 in]
              n1118 = call "myRIO_BRig_RT_dataLC_Cue1_Count_Switch_l1.vi"() -> ("output_Cue1_Count_Switch_l1"=w1964:i32)  [unwired: 11 in]
              n1119 = local read "LC_Cue1_delayOpt_Switch_l1"() -> (w1950:bool)
              n1120 = call "myRIO_BRig_RT_dataLC_Cue1_Block_NS_l1.vi"() -> ("output_Cue1_Block_NS_l1"=w1948:i32)  [unwired: 11 in]
              n1121 = call "myRIO_BRig_RT_dataLC_Cue1_OnOff_NS_l1.vi"() -> ("output_Cue1_OnOff_NS_l1"=w1947:i32)  [unwired: 11 in]
              n1122 = call "myRIO_BRig_RT_dataLC_Cue1_Probability_NS_l1.vi"() -> ("output_Cue1_l1_All_Probability"=w1946:i32)  [unwired: 11 in]
              n1123 = call "myRIO_BRig_RT_dataLC_Cue1_Tdelay_NS_l1.vi"() -> ("output_Cue1_Tdelay_NS_l1"=w1945:i32)  [unwired: 11 in]
              n1124 = call "myRIO_BRig_RT_dataLC_Cue1_Count_NS_l1.vi"() -> ("output_Cue1_Count_NS_l1"=w1944:i32)  [unwired: 11 in]
              n1125 = call "myRIO_BRig_RT_dataLC_Cue1_delayOpt_NS_l1.vi"() -> ("output_Cue1_delayOpt_NS_l1"=w1943:i32)  [unwired: 11 in]
              n1126 = local read "LC_Cue1_Count_Switch_l1"() -> (w1963:u16)
              n1127 = local read "LC_Cue1_Probability_Switch_l1"() -> (w1967:u16)
              n1128 = local read "LC_Cue1_Block_Switch_l1"() -> (w1973:u16)
              n1129 = local read "LC_Cue1_Tdelay_Switch_l1"() -> (w1965:u16)
              n1130 = local read "LC_Cue1_OnOff_Switch_l1"() -> (w1971:bool)
              n1131 = local read "LC_Cue1_OnOff_NS_l1"() -> (w1939:bool)
              n1132 = call "myRIO_BRig_RT_dataLC_Selection_Block_NS_l1.vi"() -> ("output_Selection_Block_NS_l1"=w1932:i32)  [unwired: 11 in]
              n1133 = call "myRIO_BRig_RT_dataLC_Selection_OnOff_NS_l1.vi"() -> ("output_Selection_OnOff_NS_l1"=w1931:i32)  [unwired: 11 in]
              n1134 = call "myRIO_BRig_RT_dataLC_Selection_Probability_NS_l1.vi"() -> ("output_Selection_Probability_NS_l1"=w1930:i32)  [unwired: 11 in]
              n1135 = call "myRIO_BRig_RT_dataLC_Selection_Tdelay_NS_l1.vi"() -> ("output_Selection_Tdelay_NS_l1"=w1929:i32)  [unwired: 11 in]
              n1136 = call "myRIO_BRig_RT_dataLC_Selection_Count_NS_l1.vi"() -> ("output_Selection_Count_NS_l1"=w1922:i32)  [unwired: 11 in]
              n1137 = local read "LC_Cue1_delayOpt_NS_l1"() -> (w1940:bool)
              n1138 = local read "LC_Cue1_Probability_NS_l1"() -> (w1936:u16)
              n1139 = local read "LC_Cue1_Tdelay_NS_l1"() -> (w1935:u16)
              n1140 = local read "LC_Cue1_Count_NS_l1"() -> (w1934:u16)
              n1141 = local read "LC_Cue1_Block_NS_l1"() -> (w1938:u16)
              n1142 = local read "LC_Sel_Probability_NS_l1"() -> (w1924:u16)
              n1143 = local read "LC_Sel_Tdelay_NS_l1"() -> (w1923:u16)
              n1144 = local read "LC_Sel_OnOff_NS_l1"() -> (w1926:bool)
              n1145 = local read "LC_Sel_Count_NS_l1"() -> (w1921:u16)
              n1146 = local read "LC_Sel_Block_NS_l1"() -> (w1928:u16)
              n1147 = Boolean To (0,1)(Boolean=w1950) -> (0, 1=w1952:i16)
              n1148 = Boolean To (0,1)(Boolean=w1971) -> (0, 1=w1970:i16)
              n1149 = Boolean To (0,1)(Boolean=w1939) -> (0, 1=w1942:i16)
              n1150 = To Unsigned Word Integer(number=w1952) -> (unsigned 16bit integer=w1949:u16)
              n1151 = To Unsigned Word Integer(number=w1970) -> (unsigned 16bit integer=w1969:u16)
              n1152 = To Unsigned Word Integer(number=w1942) -> (unsigned 16bit integer=w1937:u16)
              n1153 = Boolean To (0,1)(Boolean=w1940) -> (0, 1=w1941:i16)
              n1154 = Boolean To (0,1)(Boolean=w1926) -> (0, 1=w1927:i16)
              n1155 = To Unsigned Word Integer(number=w1941) -> (unsigned 16bit integer=w1933:u16)
              n1156 = To Unsigned Word Integer(number=w1927) -> (unsigned 16bit integer=w1925:u16)
              n1157 = Replace Array Subset(array=w1975, new element #1=w1973, index #1=w1974, new element #2=w1969, index #2=w1972, new element #3=w1967, index #3=w1968, new element #4=w1965, index #4=w1966, new element #5=w1963, index #5=w1964, new element #6=w1949, index #6=w1951, new element #7=w1938, index #7=w1948, new element #8=w1937, index #8=w1947, new element #9=w1936, index #9=w1946, new element #10=w1935, index #10=w1945, new element #11=w1934, index #11=w1944, new element #12=w1933, index #12=w1943, new element #13=w1928, index #13=w1932, new element #14=w1925, index #14=w1931, new element #15=w1924, index #15=w1930, new element #16=w1923, index #16=w1929, new element #17=w1921, index #17=w1922) -> (w1976:u16[])
            }
            frame "saveSettings_LC_Cue_l2" {
              # "Selection All"
              # "Count"
              # "Tdelay"
              # "Probability"
              # "OnOff"
              # "Block"
              # "delayOpt"
              # "Count"
              # "Tdelay"
              # "Probability"
              # "OnOff"
              # "Block"
              # "Cue1 All"
              # "delayOpt"
              # "Count"
              # "Tdelay"
              # "Probability"
              # "OnOff"
              # "Block"
              # "Cue1 First"
              n1158 = call "myRIO_BRig_RT_dataLC_Cue1_delayOpt_Switch_l2.vi"() -> ("output_Cue1_delayOpt_Switch_l2"=w2015:i32)  [unwired: 11 in]
              n1159 = call "myRIO_BRig_RT_dataLC_Cue1_Block_Switch_l2.vi"() -> ("output_Cue1_Block_Switch_l2"=w2038:i32)  [unwired: 11 in]
              n1160 = call "myRIO_BRig_RT_dataLC_Cue1_OnOff_Switch_l2.vi"() -> ("output_Cue1_OnOff_Switch_l2"=w2036:i32)  [unwired: 11 in]
              n1161 = call "myRIO_BRig_RT_dataLC_Cue1_Probability_Switch_l2.vi"() -> ("output_Cue1_l2_First_Probability"=w2032:i32)  [unwired: 11 in]
              n1162 = call "myRIO_BRig_RT_dataLC_Cue1_Tdelay_Switch_l2.vi"() -> ("output_Cue1_Tdelay_Switch_l2"=w2030:i32)  [unwired: 11 in]
              n1163 = call "myRIO_BRig_RT_dataLC_Cue1_Count_Switch_l2.vi"() -> ("output_Cue1_Count_Switch_l2"=w2028:i32)  [unwired: 11 in]
              n1164 = local read "LC_Cue1_delayOpt_Switch_l2"() -> (w2014:bool)
              n1165 = call "myRIO_BRig_RT_dataLC_Cue1_Block_NS_l2.vi"() -> ("output_Cue1_Block_NS_l2"=w2012:i32)  [unwired: 11 in]
              n1166 = call "myRIO_BRig_RT_dataLC_Cue1_OnOff_NS_l2.vi"() -> ("output_Cue1_OnOff_NS_l2"=w2011:i32)  [unwired: 11 in]
              n1167 = call "myRIO_BRig_RT_dataLC_Cue1_Probability_NS_l2.vi"() -> ("output_Cue1_l2_All_Probability"=w2010:i32)  [unwired: 11 in]
              n1168 = call "myRIO_BRig_RT_dataLC_Cue1_Tdelay_NS_l2.vi"() -> ("output_Cue1_Tdelay_NS_l2"=w2009:i32)  [unwired: 11 in]
              n1169 = call "myRIO_BRig_RT_dataLC_Cue1_Count_NS_l2.vi"() -> ("output_Cue1_Count_NS_l2"=w2008:i32)  [unwired: 11 in]
              n1170 = call "myRIO_BRig_RT_dataLC_Cue1_delayOpt_NS_l2.vi"() -> ("output_Cue1_delayOpt_NS_l2"=w2007:i32)  [unwired: 11 in]
              n1171 = local read "LC_Cue1_Count_Switch_l2"() -> (w2027:u16)
              n1172 = local read "LC_Cue1_Probability_Switch_l2"() -> (w2031:u16)
              n1173 = local read "LC_Cue1_Block_Switch_l2"() -> (w2037:u16)
              n1174 = local read "LC_Cue1_Tdelay_Switch_l2"() -> (w2029:u16)
              n1175 = local read "LC_Cue1_OnOff_Switch_l2"() -> (w2035:bool)
              n1176 = local read "LC_Cue1_OnOff_NS_l2"() -> (w2003:bool)
              n1177 = call "myRIO_BRig_RT_dataLC_Selection_Block_NS_l2.vi"() -> ("output_Selection_Block_NS_l2"=w1988:i32)  [unwired: 11 in]
              n1178 = call "myRIO_BRig_RT_dataLC_Selection_OnOff_NS_l2.vi"() -> ("output_Selection_OnOff_NS_l2"=w1987:i32)  [unwired: 11 in]
              n1179 = call "myRIO_BRig_RT_dataLC_Selection_Probability_NS_l2.vi"() -> ("output_Selection_Probability_NS_l2"=w1986:i32)  [unwired: 11 in]
              n1180 = call "myRIO_BRig_RT_dataLC_Selection_Tdelay_NS_l2.vi"() -> ("output_Selection_Tdelay_NS_l2"=w1985:i32)  [unwired: 11 in]
              n1181 = call "myRIO_BRig_RT_dataLC_Selection_Count_NS_l2.vi"() -> ("output_Selection_Count_NS_l2"=w1984:i32)  [unwired: 11 in]
              n1182 = local read "LC_Cue1_delayOpt_NS_l2"() -> (w2004:bool)
              n1183 = local read "LC_Cue1_Probability_NS_l2"() -> (w2000:u16)
              n1184 = local read "LC_Cue1_Tdelay_NS_l2"() -> (w1999:u16)
              n1185 = local read "LC_Cue1_Count_NS_l2"() -> (w1998:u16)
              n1186 = local read "LC_Cue1_Block_NS_l2"() -> (w2002:u16)
              n1187 = local read "LC_Sel_Probability_NS_l2"() -> (w1992:u16)
              n1188 = local read "LC_Sel_Tdelay_NS_l2"() -> (w1991:u16)
              n1189 = local read "LC_Sel_OnOff_NS_l2"() -> (w1994:bool)
              n1190 = local read "LC_Sel_Count_NS_l2"() -> (w1990:u16)
              n1191 = local read "LC_Sel_Block_NS_l2"() -> (w1996:u16)
              n1192 = Boolean To (0,1)(Boolean=w2014) -> (0, 1=w2016:i16)
              n1193 = Boolean To (0,1)(Boolean=w2035) -> (0, 1=w2034:i16)
              n1194 = Boolean To (0,1)(Boolean=w2003) -> (0, 1=w2006:i16)
              n1195 = To Unsigned Word Integer(number=w2016) -> (unsigned 16bit integer=w2013:u16)
              n1196 = To Unsigned Word Integer(number=w2034) -> (unsigned 16bit integer=w2033:u16)
              n1197 = To Unsigned Word Integer(number=w2006) -> (unsigned 16bit integer=w2001:u16)
              n1198 = Boolean To (0,1)(Boolean=w2004) -> (0, 1=w2005:i16)
              n1199 = Boolean To (0,1)(Boolean=w1994) -> (0, 1=w1995:i16)
              n1200 = To Unsigned Word Integer(number=w2005) -> (unsigned 16bit integer=w1997:u16)
              n1201 = To Unsigned Word Integer(number=w1995) -> (unsigned 16bit integer=w1993:u16)
              n1202 = Replace Array Subset(array=w2039, new element #1=w2037, index #1=w2038, new element #2=w2033, index #2=w2036, new element #3=w2031, index #3=w2032, new element #4=w2029, index #4=w2030, new element #5=w2027, index #5=w2028, new element #6=w2013, index #6=w2015, new element #7=w2002, index #7=w2012, new element #8=w2001, index #8=w2011, new element #9=w2000, index #9=w2010, new element #10=w1999, index #10=w2009, new element #11=w1998, index #11=w2008, new element #12=w1997, index #12=w2007, new element #13=w1996, index #13=w1988, new element #14=w1993, index #14=w1987, new element #15=w1992, index #15=w1986, new element #16=w1991, index #16=w1985, new element #17=w1990, index #17=w1984) -> (w2040:u16[])
            }
            frame "saveSettings6_LC_l1_Other" {
              # "Trial"
              # "Tdelay"
              # "Probability"
              # "OnOff"
              # "Block"
              # "Wrong"
              # "Trial"
              # "Tdelay"
              # "Probability"
              # "OnOff"
              # "Block"
              # "Reward"
              n1203 = call "myRIO_BRig_RT_dataLC_Wrong_Block_l1.vi"() -> ("output_Wrong_Block_l1"=w2069:i32)  [unwired: 11 in]
              n1204 = call "myRIO_BRig_RT_dataLC_Wrong_OnOff_l1.vi"() -> ("output_Wrong_OnOff_l1"=w2068:i32)  [unwired: 11 in]
              n1205 = call "myRIO_BRig_RT_dataLC_Wrong_Probability_l1.vi"() -> ("output_Wrong_Probability_l1"=w2067:i32)  [unwired: 11 in]
              n1206 = call "myRIO_BRig_RT_dataLC_Wrong_Tdelay_l1.vi"() -> ("output_Wrong_Tdelay_l1"=w2066:i32)  [unwired: 11 in]
              n1207 = call "myRIO_BRig_RT_dataLC_Wrong_Trial_l1.vi"() -> ("output_Wrong_Trial_l1"=w2065:i32)  [unwired: 11 in]
              n1208 = call "myRIO_BRig_RT_dataLC_Reward_Block_l1.vi"() -> ("output_Reward_Block_l1"=w2081:i32)  [unwired: 11 in]
              n1209 = call "myRIO_BRig_RT_dataLC_Reward_OnOff_l1.vi"() -> ("output_Reward_OnOff_l1"=w2079:i32)  [unwired: 11 in]
              n1210 = call "myRIO_BRig_RT_dataLC_Reward_Probability_l1.vi"() -> ("output_Reward_Probability_l1"=w2075:i32)  [unwired: 11 in]
              n1211 = call "myRIO_BRig_RT_dataLC_Reward_Tdelay_l1.vi"() -> ("output_Reward_Tdelay_l1"=w2073:i32)  [unwired: 11 in]
              n1212 = call "myRIO_BRig_RT_dataLC_Reward_Trial_l1.vi"() -> ("output_Reward_Trial_l1"=w2071:i32)  [unwired: 11 in]
              n1213 = local read "LC_Wrong_OnOff_l1"() -> (w2063:bool)
              n1214 = local read "LC_Wrong_Probability_l1"() -> (w2060:u16)
              n1215 = local read "LC_Wrong_Block_l1"() -> (w2062:u16)
              n1216 = local read "LC_Wrong_Tdelay_l1"() -> (w2059:u16)
              n1217 = local read "LC_Wrong_Trial_l1"() -> (w2058:u16)
              n1218 = local read "LC_Reward_Probability_l1"() -> (w2074:u16)
              n1219 = local read "LC_Reward_Block_l1"() -> (w2080:u16)
              n1220 = local read "LC_Reward_Tdelay_l1"() -> (w2072:u16)
              n1221 = local read "LC_Reward_OnOff_l1"() -> (w2078:bool)
              n1222 = local read "LC_Reward_Trial_l1"() -> (w2070:u16)
              n1223 = Boolean To (0,1)(Boolean=w2063) -> (0, 1=w2064:i16)
              n1224 = Boolean To (0,1)(Boolean=w2078) -> (0, 1=w2077:i16)
              n1225 = To Unsigned Word Integer(number=w2064) -> (unsigned 16bit integer=w2061:u16)
              n1226 = To Unsigned Word Integer(number=w2077) -> (unsigned 16bit integer=w2076:u16)
              n1227 = Replace Array Subset(array=w2082, new element #1=w2080, index #1=w2081, new element #2=w2076, index #2=w2079, new element #3=w2074, index #3=w2075, new element #4=w2072, index #4=w2073, new element #5=w2070, index #5=w2071, new element #6=w2062, index #6=w2069, new element #7=w2061, index #7=w2068, new element #8=w2060, index #8=w2067, new element #9=w2059, index #9=w2066, new element #10=w2058, index #10=w2065) -> (w2083:u16[])
            }
            frame "SaveSettings6_LC_l2_Other" {
              # "Trial"
              # "Tdelay"
              # "Probability"
              # "OnOff"
              # "Block"
              # "Wrong"
              # "Trial"
              # "Tdelay"
              # "Probability"
              # "OnOff"
              # "Block"
              # "Reward"
              n1228 = call "myRIO_BRig_RT_dataLC_Wrong_Block_l2.vi"() -> ("output_Wrong_Block_l2"=w2092:i32)  [unwired: 11 in]
              n1229 = call "myRIO_BRig_RT_dataLC_Wrong_OnOff_l2.vi"() -> ("output_Wrong_OnOff_l2"=w2093:i32)  [unwired: 11 in]
              n1230 = call "myRIO_BRig_RT_dataLC_Wrong_Probability_l2.vi"() -> ("output_Wrong_Probability_l2"=w2094:i32)  [unwired: 11 in]
              n1231 = call "myRIO_BRig_RT_dataLC_Wrong_Tdelay_l2.vi"() -> ("output_Wrong_Tdelay_l2"=w2095:i32)  [unwired: 11 in]
              n1232 = call "myRIO_BRig_RT_dataLC_Wrong_Trial_l2.vi"() -> ("output_Wrong_Trial_l2"=w2096:i32)  [unwired: 11 in]
              n1233 = call "myRIO_BRig_RT_dataLC_Reward_Block_l2.vi"() -> ("output_Reward_Block_l2"=w2097:i32)  [unwired: 11 in]
              n1234 = call "myRIO_BRig_RT_dataLC_Reward_OnOff_l2.vi"() -> ("output_Reward_OnOff_l2"=w2098:i32)  [unwired: 11 in]
              n1235 = call "myRIO_BRig_RT_dataLC_Reward_Probability_l2.vi"() -> ("output_Reward_Probability_l2"=w2099:i32)  [unwired: 11 in]
              n1236 = call "myRIO_BRig_RT_dataLC_Reward_Tdelay_l2.vi"() -> ("output_Reward_Tdelay_l2"=w2100:i32)  [unwired: 11 in]
              n1237 = call "myRIO_BRig_RT_dataLC_Reward_Trial_l2.vi"() -> ("output_Reward_Trial_l2"=w2101:i32)  [unwired: 11 in]
              n1238 = local read "LC_Wrong_OnOff_l2"() -> (w2117:bool)
              n1239 = local read "LC_Wrong_Probability_l2"() -> (w2114:u16)
              n1240 = local read "LC_Wrong_Block_l2"() -> (w2116:u16)
              n1241 = local read "LC_Wrong_Tdelay_l2"() -> (w2113:u16)
              n1242 = local read "LC_Wrong_Trial_l2"() -> (w2112:u16)
              n1243 = local read "LC_Reward_Probability_l2"() -> (w2121:u16)
              n1244 = local read "LC_Reward_Block_l2"() -> (w2125:u16)
              n1245 = local read "LC_Reward_Tdelay_l2"() -> (w2120:u16)
              n1246 = local read "LC_Reward_OnOff_l2"() -> (w2124:bool)
              n1247 = local read "LC_Reward_Trial_l2"() -> (w2119:u16)
              n1248 = Boolean To (0,1)(Boolean=w2117) -> (0, 1=w2118:i16)
              n1249 = Boolean To (0,1)(Boolean=w2124) -> (0, 1=w2123:i16)
              n1250 = To Unsigned Word Integer(number=w2118) -> (unsigned 16bit integer=w2115:u16)
              n1251 = To Unsigned Word Integer(number=w2123) -> (unsigned 16bit integer=w2122:u16)
              n1252 = Replace Array Subset(array=w2126, new element #1=w2125, index #1=w2097, new element #2=w2122, index #2=w2098, new element #3=w2121, index #3=w2099, new element #4=w2120, index #4=w2100, new element #5=w2119, index #5=w2101, new element #6=w2116, index #6=w2092, new element #7=w2115, index #7=w2093, new element #8=w2114, index #8=w2094, new element #9=w2113, index #9=w2095, new element #10=w2112, index #10=w2096) -> (w2127:u16[])
            }
            frame "setSettings_Audio" {
              # "amp_L"
              # "amp_R"
              # "freq_L"
              # "freq_R"
              n1253 = call "myRIO_BRig_RT_dataExp_Audio_amp__L.vi"() -> ("output_Audio_amp__L"=w2152:i32)  [unwired: 11 in]
              n1254 = call "myRIO_BRig_RT_dataExp_Audio_amp__R.vi"() -> ("output_Audio_amp__R"=w2151:i32)  [unwired: 11 in]
              n1255 = call "myRIO_BRig_RT_dataExp_Audio_freq__L.vi"() -> ("output_Audio_freq__L"=w2150:i32)  [unwired: 11 in]
              n1256 = call "myRIO_BRig_RT_dataExp_Audio_freq__R.vi"() -> ("output_Audio_freq__R"=w2149:i32)  [unwired: 11 in]
              n1257 = Index Array(array=w2148, index #1=w2152, index #2=w2151, index #3=w2150, index #4=w2149) -> (element #1=w2147:u16, element #2=w2146:u16, element #3=w2139:u16, element #4=w2137:u16)
              n1258 = To Unsigned Byte Integer(number=w2139) -> (unsigned 8bit integer=w2138:u8)
              n1259 = To Unsigned Byte Integer(number=w2137) -> (unsigned 8bit integer=w2136:u8)
            }
            frame "setSettings_Laser" {
              w2174 = u32 0 ("laser2_selRew_Ndelay")
              # "tDelay"
              # "Wrong l1"
              # "Reward l1"
              n1260 = local read "Laser_Tpeak_l1"() -> (w2188:dbl)
              n1261 = local read "Laser_Tshutter_l1"() -> (w2186:dbl)
              n1262 = local read "Laser_Freq_l1"() -> (w2187:dbl)
              n1263 = local read "Laser_duration_l1"() -> (w2183:u16)
              n1264 = local read "Laser_Tpeak_l2"() -> (w2182:dbl)
              n1265 = local read "Laser_Tshutter_l2"() -> (w2180:dbl)
              n1266 = local read "Laser_Freq_l2"() -> (w2181:dbl)
              n1267 = local read "Laser_duration_l2"() -> (w2179:u16)
              n1268 = local read "CueLed_Freq"() -> (w2166:dbl)
              n1269 = local read "CueLed_duration"() -> (w2165:u16)
              n1270 = local read "CueLed_Tpeak"() -> (w2167:dbl)
              n1271 = call "myRIO_BRig_RT_dataLC_Reward_Tdelay_l1.vi"() -> ("output_Reward_Tdelay_l1"=w2201:i32)  [unwired: 11 in]
              n1272 = call "myRIO_BRig_RT_dataLC_Wrong_Tdelay_l1.vi"() -> ("output_Wrong_Tdelay_l1"=w2202:i32)  [unwired: 11 in]
              n1273 = local read "FPGA_count2ms"() -> (w2168:dbl)
              n1274 = Index Array(array=w2198, index #1=w2201, index #2=w2202) -> (element #1=w2200:u16, element #2=w2199:u16)
              n1275 = To Double Precision Float(number=w2200) -> (double precision float=w2195:dbl)
              n1276 = To Double Precision Float(number=w2199) -> (double precision float=w2192:dbl)
              n1277 = To Unsigned Word Integer(number=w2168) -> (unsigned 16bit integer=w2189:u16)
              n1278 = call "myRIO_BRig_RT__calc_laser_FPGA_N.vi"("input_FPGA_count2ms"=w2168, "input_Tpeak"=w2188, "input_Freq"=w2187, "input_Tshutter"=w2186, "input_duration"=w2183) -> ("output_laser_Npeak"=w2173:u32, "output_laser_Nvalley"=w2172:u32, "output_laser_Nshutter"=w2171:u32, "output_laser_Nduration"=w2185:u32, "output_laser_Tduration"=w2184:u16)  [unwired: 6 in]
              n1279 = Multiply(x=w2168, y=w2195) -> (x*y=w2196:dbl)
              n1280 = Multiply(x=w2168, y=w2192) -> (x*y=w2193:dbl)
              n1281 = call "myRIO_BRig_RT__calc_laser_FPGA_N__CueLed.vi"("input_FPGA_count2ms"=w2168, "input_Tpeak"=w2167, "input_Freq"=w2166, "input_duration"=w2165) -> ("output_laser_Npeak"=w2164:u32, "output_laser_Nvalley"=w2163:u32, "output_laser_Tduration"=w2161:u16)  [unwired: 9 in]
              n1282 = call "myRIO_BRig_RT__calc_laser_FPGA_N.vi"("input_FPGA_count2ms"=w2168, "input_Tpeak"=w2182, "input_Freq"=w2181, "input_Tshutter"=w2180, "input_duration"=w2179) -> ("output_laser_Npeak"=w2178:u32, "output_laser_Nvalley"=w2177:u32, "output_laser_Nshutter"=w2176:u32, "output_laser_Nduration"=w2175:u32, "output_laser_Tduration"=w2169:u16)  [unwired: 6 in]
              n1283 = Round Toward +Infinity(x=w2196) -> (ceil(x): smallest int >= x=w2197:dbl)
              n1284 = Round Toward +Infinity(x=w2193) -> (ceil(x): smallest int >= x=w2194:dbl)
              n1285 = To Unsigned Long Integer(number=w2197) -> (unsigned 32bit integer=w2191:u32)
              n1286 = To Unsigned Long Integer(number=w2194) -> (unsigned 32bit integer=w2190:u32)
              n1287 = xnode "Read/Write Control"("FPGA VI Reference In"=w2205, "error in"=w2206, "LC_nPeak_l1"=w2173, "LC_nValley_l1"=w2172, "LC_nShutter_l1"=w2171, "LR_reward_nDelay_l1"=w2191, "LR_wrong_nDelay_l1"=w2190, "LR_reward_nTotal_l1"=w2185, "LR_wrong_nTotal_l1"=w2185, "k1__counter_per_ms"=w2189, "LC_nPeak_l2"=w2178, "LC_nValley_l2"=w2177, "LC_nShutter_l2"=w2176, "LR_reward_nDelay_l2"=w2174, "LR_wrong_nDelay_l2"=w2174, "LR_reward_nTotal_l2"=w2175, "LR_wrong_nTotal_l2"=w2175, "CueLed_nPeak"=w2164, "CueLed_nValley"=w2163) -> ("error out"=→"error out":errorcluster)  [unwired: 1 out]
              n1288 = call "myRIO_BRig_RT_dataCurrent_laser1_pulse_duration.vi"() -> ("output_laser1_pulse_duration"=w2203:i32)  [unwired: 11 in]
              n1289 = call "myRIO_BRig_RT_dataCurrent_laser2_pulse_duration.vi"() -> ("output_laser2_pulse_duration"=w2170:i32)  [unwired: 11 in]
              n1290 = call "myRIO_BRig_RT_dataCurrent_CueLed_pulse_duration.vi"() -> ("output_CueLed_pulse_duration"=w2162:i32)  [unwired: 11 in]
              n1291 = Replace Array Subset(array=w2198, new element #1=w2184, index #1=w2203, new element #2=w2169, index #2=w2170, new element #3=w2161, index #3=w2162) -> (w2204:u16[])
            }
            frame "initBlock" {
              n1292 = call "myRIO_Brig_RT__Case_Exp_State_initBlock.vi"("input_spout"=w2250, "input_dataExp"=w2248, "input_dataCurrent"=w2249) -> ("output_spout"=w2228:enum16{"Left", "Right"}, "output_state"=w2251:T2, "output_dataExp"=w2247:u16[], "output_dataCurrent"=w2233:u16[], "output_TpB_target"=→"TpB_target":u16)  [unwired: 4 in]
              "cSpout" <- w2228
              n1293 = call "myRIO_BRig_RT_dataCurrent_iBlock.vi"() -> ("output_iBlock"=w2232:i32)  [unwired: 11 in]
              n1294 = Index Array(array=w2233, index=w2232) -> (element=w2226:u16)
              "iBlock" <- w2226
            }
            frame "initBlock2" {
              n1295 = local write "nRewards_cur"(u16 0 ("nRewards_cur")) -> ()
              n1296 = call "myRIO_BRig_RT__Case_Exp_State_initBlock2.vi"("input_spout"=w2259, "input_dataBlock"=w2260, "input_dataCurrent"=w2258) -> ("idxDataBlock"=w2255:i32, "output_dataBlock"=w2257:u16[][])  [unwired: 7 in]
            }
            frame "initTrial" {
              n1297 = call "myRIO_Brig_RT__Case_Exp_State_initTrial.vi"("input_spout"=w2273, "input_dataExp"=w2294, "input_dataCurrent"=w2295) -> ("output_state"=w2296:T2, "output_dataExp"=w2293:u16[], "output_dataCurrent"=w2283:u16[])  [unwired: 6 in]
              n1298 = call "myRIO_BRig_RT_dataCurrent_iTrial.vi"() -> ("output_iTrial"=w2282:i32)  [unwired: 11 in]
              n1299 = call "myRIO_BRig_RT_dataCurrent_SolenoidReward.vi"() -> ("output_SolenoidReward"=w2278:i32)  [unwired: 11 in]
              n1300 = Index Array(array=w2283, index #1=w2282, index #2=w2278) -> (element #1=w2274:u16, element #2=w2277:u16)
              "iTrial" <- w2274
              n1301 = Not Equal To 0?(x=w2277) -> (x != 0?=→"SolenoidReward":bool)
            }
            frame "initTrial2" {
              # "trialUntilReward"
              n1302 = call "myRIO_BRig_RT__Case_Exp_subState_LC__initTrial__v3.vi"("input_dataCurrent"=w2309, "input_dataLC"=w2308, "input_spout"=w2310, "input_dataTrial"=w2312) -> ("output_dataTrial"=w2311:u16[][], "output_LR_Wrong_Laser_l2"=w2300:bool, "output_LR_Reward_Laser_l2"=w2301:bool, "output_LR_Reward_Event_l1"=w2307:bool, "output_LR_Wrong_Event_l1"=w2306:bool, "output_LR_Reward_Laser_l1"=w2305:bool, "output_LR_Wrong_Laser_l1"=w2304:bool, "output_LR_Reward_Event_l2"=w2303:bool, "output_LR_Wrong_Event_l2"=w2302:bool)  [unwired: 7 in]
              n1303 = call "myRIO_BRig_RT_dataExp_ItrialUntilReward.vi"() -> ("output_I_trialUntilReward"=w2316:i32)  [unwired: 11 in]
              n1304 = Index Array(array=w2317, index=w2316) -> (element=w2315:u16)
              n1305 = Equal?(x=w2310, y=enum16{"Left", "Right"}."Right") -> (x = y?=w2314:bool)
              n1306 = Not Equal To 0?(x=w2315) -> (x != 0?=w2313:bool)
              n1307 = xnode "Read/Write Control"("FPGA VI Reference In"=w2331, "error in"=w2330, "SelectionState"=FALSE, "Left(F)_or_Right(T)"=w2314, "ignoreWrong"=w2313, "LR_reward_Event_l1"=w2307, "LR_wrong_Event_l1"=w2306, "LR_reward_Laser_l1"=w2305, "LR_wrong_Laser_l1"=w2304, "LR_reward_Event_l2"=w2303, "LR_wrong_Event_l2"=w2302, "LR_reward_Laser_l2"=w2301, "LR_wrong_laser_l2"=w2300) -> ("error out"=→"error_initTrial":errorcluster)  [unwired: 1 out]
            }
            frame "initTrial3" {
              n1308 = call "myRIO_BRig_RT_arrTrig_init.vi"() -> ("output_arrTrig"=w2342:bool[])  [unwired: 11 in]
              n1309 = call "myRIO_BRig_RT__Case_Exp_State_initTrial_dataTrial.vi"("input_spout"=w2352, "input_dataCurrent"=w2353, "input_dataExp"=w2351, "input_dataTrial"=w2355) -> ("output_laserPower_l2"=w2338:u16, "output_dataTrial"=w2354:u16[][], "output_laserPower_l1"=w2348:u16)  [unwired: 5 in]
              n1310 = To Double Precision Float(number=w2348) -> (double precision float=w2350:dbl)
              n1311 = To Double Precision Float(number=w2338) -> (double precision float=w2341:dbl)
              n1312 = Divide(x=w2350, y=100.0 ("x")) -> (x/y=w2344:dbl)
              "power_l1" <- w2344
              n1313 = Divide(x=w2341, y=100.0 ("x")) -> (x/y=w2339:dbl)
              "power_l2" <- w2339
              n1314 = call "myRIO__convert__Voltage_to_FPGAvalue.vi"("input_voltage"=w2344) -> ("output_PortC"=w2343:i16)  [unwired: 9 in, 1 out]
              n1315 = call "myRIO__convert__Voltage_to_FPGAvalue.vi"("input_voltage"=w2339) -> ("output_PortC"=w2337:i16)  [unwired: 9 in, 1 out]
              n1316 = xnode "Read/Write Control"("FPGA VI Reference In"=w2347, "error in"=w2346, "AnaOut_0"=w2343, "AnaOut_1"=w2337) -> ("error out"=→"error out 4":errorcluster)  [unwired: 1 out]
            }
            frame "initTrial4" {
              n1317 = call "myRIO_BRig_RT_dataCurrent_idxDataTrial.vi"() -> ("output_idxDataTrial"=w2379:i32)  [unwired: 11 in]
              n1318 = call "myRIO_BRig_RT_dataTrial_activeRecording.vi"() -> ("output_activeRecording"=w2376:i32)  [unwired: 11 in]
              n1319 = Index Array(array=w2381, index=w2379) -> (element=w2378:u16)
              n1320 = Boolean To (0,1)(Boolean="Recording") -> (0, 1=w2375:i16)
              n1321 = To Long Integer(number=w2378) -> (32bit integer=w2377:i32)
              n1322 = To Unsigned Word Integer(number=w2375) -> (unsigned 16bit integer=w2374:u16)
              n1323 = Replace Array Subset(array=w2380, new element=w2374, index (row)=w2377, index (col)=w2376) -> (w2373:u16[][])
            }
            frame "initTrial_LC_ENL1" {
              n1324 = call "myRIO_BRig_RT__Case_Exp_State_initTrial_LC_ENL1__v3.vi"("input_dataTrial"=w2403, "input_spout"=w2406, "input_arrTrig"=w2400, "input_dataBlock"=w2401, "input_dataLC"=w2407, "input_dataCurrent"=w2405) -> ("output_arrTrig"=w2399:bool[], "output_dataTrial"=w2402:u16[][], "output_dataCurrent"=w2404:u16[])  [unwired: 3 in]
            }
            frame "initTrial_LC_Cue1" {
              n1325 = call "myRIO_BRig_RT__Case_Exp_State_initTrial_LC_Cue1__v3.vi"("input_dataTrial"=w2426, "input_spout"=w2429, "input_arrTrig"=w2423, "input_dataBlock"=w2424, "input_dataLC"=w2430, "input_dataCurrent"=w2428) -> ("output_arrTrig"=w2422:bool[], "output_dataTrial"=w2425:u16[][], "output_dataCurrent"=w2427:u16[])  [unwired: 3 in]
            }
            frame "initTrial_LC_Cue1_2" {
              w2458 = TRUE ("Recording")
              n1326 = local read "Cue1Param_AudioLed_Probability_Switch"() -> (w2451:u16)
              n1327 = local read "Cue1Param_AudioLed_Count_Switch"() -> (w2450:u16)
              n1328 = local read "Cue1Param_AudioLed_Probability_NS"() -> (w2448:u16)
              n1329 = local read "Cue1Param_AudioLed_Count_NS"() -> (w2447:u16)
              n1330 = local read "Cue1Param_CueType_Switch"() -> (w2452:u16)
              n1331 = local read "Cue1Param_CueType_NS"() -> (w2449:u16)
              n1332 = call "myRIO_BRig_RT__Case_Exp_State_initTrial_LC_Cue1_2.vi"("input_CueType_Switch"=w2452, "input_Probability_Switch"=w2451, "input_Count_Switch"=w2450, "input_CueType_NS"=w2449, "input_Probability_NS"=w2448, "input_Count_NS"=w2447, "input_spout"=w2446, "input_dataBlock"=w2445, "input_dataCurrent"=w2456, "input_arrTrig"=w2454) -> ("output_dataCurrent"=w2455:u16[], "output_arrTrig"=w2453:bool[])  [unwired: 8 in]
            }
            frame "initTrial_LC_Sel" {
              n1333 = call "myRIO_BRig_RT__Case_Exp_State_initTrial_LC_Sel__v3.vi"("input_dataTrial"=w2480, "input_spout"=w2483, "input_arrTrig"=w2475, "input_dataBlock"=w2478, "input_dataLC"=w2484, "input_dataCurrent"=w2482) -> ("output_arrTrig"=w2474:bool[], "output_dataTrial"=w2479:u16[][], "output_dataCurrent"=w2481:u16[])  [unwired: 3 in]
              n1334 = local read "Recording"() -> (w2477:bool)
            }
            frame "ENL1_pre" {
              n1335 = call "myRIO_BRig_RT__Case_Exp_State_Enl1Pre__v3.vi"("input_I_lick"=w2502, "input_arrTrig"=w2499, "input_dataCurrent"=w2503) -> ("output_dataCurrent"=w2500:u16[], "output_state"=w2501:T2)  [unwired: 3 in, 4 out]
            }
            frame "ENL1" {
              n1336 = call "myRIO_BRig_RT__Case_Exp_State_ENL1__v3.vi"("I_lick"=w2526, "input_arrTrig"=w2524, "input_state"=w2530, "input_dataCurrent"=w2529) -> ("output_l1_laserOn"=w2522:bool, "output_l1_laserEvent"=w2523:bool, "output_state"=w2527:T2, "output_dataCurrent"=w2528:u16[], "output_l2_laserEvent"=w2521:bool, "output_l2_laserOn"=w2520:bool)  [unwired: 2 in]
            }
            frame "ENL1Penalty_pre" {
              # "Tcycle"
              # "counter"
              n1337 = call "myRIO_BRig_RT_dataCurrent_Tcycle_generic.vi"() -> ("output_Tcycle_generic"=w2565:i32)  [unwired: 11 in]
              n1338 = call "myRIO_BRig_RT_dataCurrent_count_generic.vi"() -> ("output_count_generic"=w2567:i32)  [unwired: 11 in]
              n1339 = call "myRIO_BRig_RT_dataExp_ENL_penalty.vi"() -> ("output_ENL_penalty"=w2560:i32)  [unwired: 11 in]
              n1340 = Index Array(array=w2561, index=w2560) -> (element=w2564:u16)
              n1341 = Replace Array Subset(array=w2562, new element #1=u16 0 ("new element/subarray"), index #1=w2567, new element #2=w2564, index #2=w2565) -> (w2563:u16[])
            }
            frame "ENL1Penalty" {
              n1342 = call "myRIO_BRig_RT__Case_Exp_State_ENL1Penalty.vi"("input_state"=w2585, "input_dataCurrent"=w2589) -> ("output_state"=w2586:T2, "output_dataCurrent"=w2588:u16[])  [unwired: 8 in]
            }
            frame "ENL2_pre" {
            }
            frame "ENL2" {
            }
            frame "ENL2Penalty_pre" {
            }
            frame "ENL2Penalty" {
            }
            frame "Cue1_pre" {
              n1343 = call "myRIO_BRig_RT__Case_Exp_State_Cue1Pre__v3.vi"("input_dataCurrent"=w2677, "input_dataExp"=w2673, "input_arrTrig"=w2670, "input_spout"=w2674) -> ("output_audioR"=w2671:bool, "output_audioL"=w2672:bool, "output_state"=w2675:T2, "output_dataCurrent"=w2676:u16[])  [unwired: 7 in, 5 out]
            }
            frame "Cue1" {
              n1344 = call "myRIO_BRig_RT__Case_Exp_State_Cue1__v3.vi"("I_lick"=w2700, "input_arrTrig"=w2698, "input_state"=w2702, "input_dataCurrent"=w2720) -> ("output_l1_laserOn"=w2696:bool, "output_l1_laserEvent"=w2697:bool, "output_state"=w2701:T2, "output_dataCurrent"=w2719:u16[], "output_l2_laserEvent"=w2695:bool, "output_CueLed_Event"=w2693:bool, "output_l2_laserOn"=w2694:bool)  [unwired: 1 in]
              n1345 = Equal?(x=myRIO_BRig_RT__Case_Exp_stateList."Selection_pre", y=w2701) -> (x = y?=w2705:bool)
              n1346 = xnode "Read/Write Control"("FPGA VI Reference In"=w2704, "error in"=w2703, "SelectionState"=w2705) -> ()  [unwired: 2 out]
            }
            frame "Cue1Penalty_pre" {
              # "Tcycle"
              # "counter"
              n1347 = call "myRIO_BRig_RT_dataCurrent_Tcycle_generic.vi"() -> ("output_Tcycle_generic"=w2746:i32)  [unwired: 11 in]
              n1348 = call "myRIO_BRig_RT_dataCurrent_count_generic.vi"() -> ("output_count_generic"=w2748:i32)  [unwired: 11 in]
              n1349 = call "myRIO_BRig_RT_dataExp_Tcycle_Cue1Penalty_Audio.vi"() -> ("output_Tcycle_Cue1Penalty_Audio"=w2745:i32)  [unwired: 11 in]
              n1350 = Index Array(array=w2740, index=w2745) -> (element=w2744:u16)
              n1351 = Replace Array Subset(array=w2742, new element #1=u16 0 ("new element/subarray"), index #1=w2748, new element #2=w2744, index #2=w2746) -> (w2741:u16[])
            }
            frame "Cue1Penalty" {
              n1352 = call "myRIO_BRig_RT__Case_Exp_State_Cue1Penalty.vi"("input_state"=w2769, "input_dataCurrent"=w2770) -> ("output_state"=w2767:T2, "output_dataCurrent"=w2768:u16[])  [unwired: 8 in]
            }
            frame "Cue2_pre" {
            }
            frame "Cue2" {
            }
            frame "Cue2Penalty_pre" {
            }
            frame "Cue2Penalty" {
            }
            frame "Selection_pre" {
              n1353 = xnode "Read/Write Control"("FPGA VI Reference In"=w2862, "error in"=w2863) -> ("error out"=→"error_Selection_pre":errorcluster, "SelectReward"=w2856:bool, "SelectWrong"=w2857:bool)  [unwired: 1 out]
              n1354 = call "myRIO_BRig_RT__Case_Exp_State_SelectPre__v3.vi"("input_dataCurrent"=w2860, "input_SelectWrong"=w2857, "input_SelectReward"=w2856, "input_dataExp"=w2850, "input_arrTrig"=w2855) -> ("output_state"=w2858:T2, "output_dataCurrent"=w2859:u16[], "output_l1_laserEvent"=w2854:bool, "output_l1_laserOn"=w2853:bool, "output_l2_laserOn"=w2851:bool, "output_l2_laserEvent"=w2852:bool)  [unwired: 5 in]
            }
            frame "Selection" {
              n1355 = xnode "Read/Write Control"("FPGA VI Reference In"=w2893, "error in"=w2892) -> ("error out"=→"error_Selection":errorcluster, "SelectReward"=w2886:bool, "SelectWrong"=w2885:bool)  [unwired: 1 out]
              n1356 = call "myRIO_BRig_RT__Case_Exp_State_Selection__v2.vi"("input_dataCurrent"=w2890, "input_state"=w2888, "input_FPGA_SelectReward"=w2886, "input_FPGA_SelectWrong"=w2885, "input_arrTrig"=w2884) -> ("output_state"=w2887:T2, "output_dataCurrent"=w2889:u16[], "output_LC_Event_l1"=w2883:bool, "output_LC_Laser_l2"=w2880:bool, "output_LC_Event_l2"=w2881:bool, "output_LC_Laser_l1"=w2882:bool)  [unwired: 5 in]
            }
            frame "SelectReward_pre" {
              # "iState"
              # "Tcycle\nReward"
              # "nRewTrials"
              # "Tcycle\nGeneric"
              # "counter"
              n1357 = call "myRIO_BRig_RT_dataCurrent_nRewTrials.vi"() -> ("output_nRewTrials"=w2925:i32)  [unwired: 11 in]
              n1358 = Equal?(x=w2934, y=enum16{"Left", "Right"}."Left") -> (x = y?=w2935:bool)
              n1359 = Index Array(array=w2926, index=w2925) -> (element=w2924:u16)
              n1360 = call "myRIO_BRig_RT_dataExp_Tcycle_Reward__L.vi"() -> ("output_Tcycle_Reward__L"=w2938:i32)  [unwired: 11 in]
              n1361 = call "myRIO_BRig_RT_dataExp_Tcycle_Reward__R.vi"() -> ("output_Tcycle_Reward__R"=w2939:i32)  [unwired: 11 in]
              n1362 = Increment(x=w2924) -> (x+1=w2923:u16)
              n1363 = Select(t=w2938, s=w2935, f=w2939) -> (s? t:f=w2937:i32)
              n1364 = call "myRIO_BRig_RT__Case_Exp_subState_LC__Reward.vi"("input_spout"=w2934, "input_dataCurrent"=w2926, "input_dataLC"=w2933) -> ()  [unwired: 6 in, 2 out]
              n1365 = call "myRIO_BRig_RT_dataCurrent_count_generic.vi"() -> ("output_count_generic"=w2928:i32)  [unwired: 11 in]
              n1366 = call "myRIO_BRig_RT_dataCurrent_Tcycle_generic.vi"() -> ("output_Tcycle_generic"=w2929:i32)  [unwired: 11 in]
              n1367 = Index Array(array=w2940, index=w2937) -> (element=w2930:u16)
              n1368 = call "myRIO_BRig_RT_dataCurrent_iState.vi"() -> ("output_iState"=w2918:i32)  [unwired: 11 in]
              n1369 = Replace Array Subset(array=w2926, new element #1=w2923, index #1=w2925, new element #2=u16 0 ("new element/subarray"), index #2=w2928, new element #3=w2930, index #3=w2929, new element #4=u16 1 ("new element/subarray"), index #4=w2918) -> (w2941:u16[])
            }
            frame "SelectReward" {
              n1370 = call "myRIO_BRig_RT__Case_Exp_State_Reward.vi"("input_dataCurrent"=w2962, "input_state"=w2959, "input_spout"=w2957) -> ("output_dataCurrent"=w2961:u16[], "output_state"=w2960:T2, "output__L"=w2955:bool, "output__R"=w2956:bool)  [unwired: 9 in]
            }
            frame "SelectRewardPost_pre" {
              # "nRewards"
              # "nRewTrials"
              # "Tcycle"
              # "counter"
              n1371 = call "myRIO_BRig_RT_dataBlock_nRewards__L.vi"() -> ("output_nRewards__L"=w2978:i32)  [unwired: 11 in]
              n1372 = call "myRIO_BRig_RT_dataBlock_nRewards__R.vi"() -> ("output_nRewards__R"=w2977:i32)  [unwired: 11 in]
              n1373 = call "myRIO_BRig_RT_dataCurrent_Tcycle_generic.vi"() -> ("output_Tcycle_generic"=w2997:i32)  [unwired: 11 in]
              n1374 = call "myRIO_BRig_RT_dataCurrent_count_generic.vi"() -> ("output_count_generic"=w2999:i32)  [unwired: 11 in]
              n1375 = case shown="\"Left\", Default" w2971 {
                tunnel: w2983 -> [w3004 w3008]
                tunnel: [w3003 w3008] -> w2982
                tunnel: [w3005 w3006] -> w2981
                tunnel: w2980 -> [w3005 w3007]
                frame "Left", Default {
                  n1376 = Increment(x=w3004) -> (x+1=w3003:u16)
                }
                frame "Right" {
                  n1377 = Increment(x=w3007) -> (x+1=w3006:u16)
                }
              }
              "nRewards_Left" <- w2982
              "nRewards_Right" <- w2981
              n1378 = Equal?(x=w2971, y=enum16{"Left", "Right"}."Left") -> (x = y?=w2970:bool)
              n1379 = Select(t=w2978, s=w2970, f=w2977) -> (s? t:f=w2976:i32)
              n1380 = call "myRIO_BRig_RT_dataExp_Tcycle_RewardPost.vi"() -> ("output_Tcycle_RewardPost"=w2993:i32)  [unwired: 11 in]
              n1381 = call "myRIO_BRig_RT_dataCurrent_nRewTrials.vi"() -> ("output_nRewTrials"=w2979:i32)  [unwired: 11 in]
              n1382 = Index Array(array=w2994, index=w2993) -> (element=w2996:u16)
              n1383 = Index Array(array=w2973, index=w2979) -> (element=w2968:u16)
              n1384 = Replace Array Subset(array=w2973, new element #1=u16 0 ("new element/subarray"), index #1=w2999, new element #2=w2996, index #2=w2997) -> (w2995:u16[])
              n1385 = Replace Array Subset(array=w2975, new element=w2968, index (row)=w2969, index (col)=w2976) -> (w2974:u16[][])
              n1386 = local write "nRewards_cur"(w2968) -> ()
            }
            frame "SelectRewardPost" {
              n1387 = call "myRIO_BRig_RT__Case_Exp_State_RewardPost.vi"("input_state"=w3023, "input_dataCurrent"=w3026) -> ("output_state"=w3024:T2, "output_dataCurrent"=w3025:u16[])  [unwired: 8 in]
            }
            frame "SelectWrong_pre" {
              # "iState"
              # "Tcycle"
              # "counter"
              n1388 = call "myRIO_BRig_RT_dataCurrent_Tcycle_generic.vi"() -> ("output_Tcycle_generic"=w3051:i32)  [unwired: 11 in]
              n1389 = call "myRIO_BRig_RT_dataCurrent_count_generic.vi"() -> ("output_count_generic"=w3053:i32)  [unwired: 11 in]
              n1390 = call "myRIO_BRig_RT_dataExp_Tcycle_Wrong.vi"() -> ("output_Tcycle_Wrong"=w3049:i32)  [unwired: 11 in]
              n1391 = call "myRIO_BRig_RT__Case_Exp_subState_LC__Wrong.vi"("input_spout"=w3045, "input_dataCurrent"=w3046, "input_dataLC"=w3043) -> ()  [unwired: 6 in, 2 out]
              n1392 = Index Array(array=w3047, index=w3049) -> (element=w3050:u16)
              n1393 = call "myRIO_BRig_RT_dataCurrent_iState.vi"() -> ("output_iState"=w3037:i32)  [unwired: 11 in]
              n1394 = Replace Array Subset(array=w3046, new element #1=u16 0 ("new element/subarray"), index #1=w3053, new element #2=w3050, index #2=w3051, new element #3=u16 2 ("new element/subarray"), index #3=w3037) -> (w3048:u16[])
            }
            frame "SelectWrong" {
              n1395 = call "myRIO_BRig_RT__Case_Exp_State_Wrong.vi"("input_state"=w3067, "input_dataCurrent"=w3076) -> ("output_state"=w3064:T2, "output_dataCurrent"=w3075:u16[])  [unwired: 8 in]
              n1396 = Not Equal?(x=w3067, y=w3064) -> (x != y?=w3066:bool)
              n1397 = Select(t=myRIO_BRig_RT__Case_Exp_stateList."SelectWrong_post" ("Enum"), s=w3066, f=w3064) -> (s? t:f=w3063:T2)
            }
            frame "SelectWrong_post" {
            }
            frame "SelectTimeout_pre" {
              # "iState"
              # "Tcycle"
              # "counter"
              n1398 = xnode "Read/Write Control"("FPGA VI Reference In"=w3103, "error in"=w3102, "SelectionState"=FALSE) -> ("error out"=→"error out 3":errorcluster)  [unwired: 1 out]
              n1399 = call "myRIO_BRig_RT_dataCurrent_Tcycle_generic.vi"() -> ("output_Tcycle_generic"=w3125:i32)  [unwired: 11 in]
              n1400 = call "myRIO_BRig_RT_dataCurrent_count_generic.vi"() -> ("output_count_generic"=w3123:i32)  [unwired: 11 in]
              n1401 = call "myRIO_BRig_RT_dataExp_Tcycle_Timeout.vi"() -> ("output_Tcycle_Timeout"=w3127:i32)  [unwired: 11 in]
              n1402 = call "myRIO_BRig_RT__Case_Exp_subState_LC__Timeout.vi"("input_spout"=w3118, "input_dataCurrent"=w3119, "input_dataLC"=w3117) -> ()  [unwired: 6 in, 2 out]
              n1403 = Index Array(array=w3121, index=w3127) -> (element=w3126:u16)
              n1404 = call "myRIO_BRig_RT_dataCurrent_iState.vi"() -> ("output_iState"=w3111:i32)  [unwired: 11 in]
              n1405 = Replace Array Subset(array=w3119, new element #1=u16 0 ("new element/subarray"), index #1=w3123, new element #2=w3126, index #2=w3125, new element #3=u16 3 ("new element/subarray"), index #3=w3111) -> (w3122:u16[])
            }
            frame "SelectTimeout" {
              n1406 = call "myRIO_BRig_RT__Case_Exp_State_Timeout.vi"("input_dataLC"=w3146, "input_state"=w3137, "input_dataCurrent"=w3151) -> ("output_state"=w3138:T2, "output_dataCurrent"=w3150:u16[])  [unwired: 6 in, 1 out]
              n1407 = Not Equal?(x=w3137, y=w3138) -> (x != y?=w3141:bool)
              n1408 = Select(t=myRIO_BRig_RT__Case_Exp_stateList."SelectTimeout_post" ("Enum"), s=w3141, f=w3138) -> (s? t:f=w3139:T2)
            }
            frame "SelectTimeout_post" {
            }
            frame "endTrial1" {
              # "Update dataBlock"
              n1409 = call "myRIO_BRig_RT__Case_Exp_State_endTrial1.vi"("input_spout"=w3184, "input_dataBlock"=w3183, "input_dataCurrent"=w3181) -> ("output_dataBlock"=w3182:u16[][], "output_dataCurrent"=w3180:u16[])  [unwired: 7 in]
            }
            frame "endTrial2" {
              # "update dataTrial"
              n1410 = call "myRIO_BRig_RT__Case_Exp_State_endTrial2.vi"("input_spout"=w3203, "input_dataTrial"=w3207, "input_dataCurrent"=w3205) -> ("output_dataTrial"=w3206:u16[][], "output_dataCurrent"=w3204:u16[])  [unwired: 7 in]
            }
            frame "endTrial3" {
              # "nRewTrials"
              # "iTrial"
              # "I_blockUntilReward"
              # "TPB"
              # "end block?"
              n1411 = local read "STOP_endTrial"() -> (w3233:bool)
              n1412 = local read "STOP_abort"() -> (w3232:bool)
              n1413 = xnode "Read/Write Control"("FPGA VI Reference In"=w3223, "error in"=w3222, "SelectionState"=FALSE) -> ("error out"=→"error out 2":errorcluster)  [unwired: 1 out]
              n1414 = local read "START"() -> (w3230:bool)
              n1415 = call "myRIO_BRig_RT_dataExp_IblockUntilReward.vi"() -> ("output_I_blockUntilReward"=w3240:i32)  [unwired: 11 in]
              n1416 = Index Array(array=w3226, index=w3240) -> (element=w3224:u16)
              n1417 = Not(x=w3230) -> (.not. x?=w3231:bool)
              n1418 = Not Equal To 0?(x=w3224) -> (x != 0?=w3238:bool)
              n1419 = Compound Arithmetic op=OR(w3233, w3231, w3232) -> (w3218:bool)
              n1420 = call "myRIO_BRig_RT_dataCurrent_nRewTrials.vi"() -> ("output_nRewTrials"=w3236:i32)  [unwired: 11 in]
              n1421 = call "myRIO_BRig_RT_dataCurrent_iTrial.vi"() -> ("output_iTrial"=w3237:i32)  [unwired: 11 in]
              n1422 = Select(t=w3236, s=w3238, f=w3237) -> (s? t:f=w3235:i32)
              n1423 = call "myRIO_BRig_RT_dataCurrent_TpB.vi"() -> ("output_TpB"=w3239:i32)  [unwired: 11 in]
              n1424 = Index Array(array=w3227, index #1=w3239, index #2=w3235) -> (element #1=w3228:u16, element #2=w3229:u16)
              n1425 = Less Or Equal?(x=w3228, y=w3229) -> (x <= y?=w3219:bool)
              n1426 = Or(x=w3218, y=w3219) -> (x .or. y?=w3216:bool)
              n1427 = Select(t=myRIO_BRig_RT__Case_Exp_stateList."saveData_dataBlock" ("Enum"), s=w3216, f=myRIO_BRig_RT__Case_Exp_stateList."dummyState" ("Enum")) -> (s? t:f=w3225:T2)
            }
            frame "endBlock" {
              # "R"
              # "L"
              # "idxDataBlock"
              n1428 = Equal?(x=w3264, y=enum16{"Left", "Right"}."Left") -> (x = y?=w3263:bool)
              n1429 = call "myRIO_BRig_RT_dataCurrent_idxDataBlockL.vi"() -> ("output_idxDataBlock__L"=w3267:i32)  [unwired: 11 in]
              n1430 = call "myRIO_BRig_RT_dataCurrent_idxDataBlockR.vi"() -> ("output_idxDataBlock__R"=w3266:i32)  [unwired: 11 in]
              n1431 = Increment(x=w3258) -> (x+1=w3257:i32)
              n1432 = local read "START"() -> (w3287:bool)
              n1433 = local read "STOP_endBlock"() -> (w3282:bool)
              n1434 = local read "STOP_endTrial"() -> (w3285:bool)
              n1435 = local read "STOP_abort"() -> (w3284:bool)
              n1436 = Select(t=w3267, s=w3263, f=w3266) -> (s? t:f=w3261:i32)
              n1437 = To Unsigned Word Integer(number=w3257) -> (unsigned 16bit integer=w3259:u16)
              n1438 = Not(x=w3287) -> (.not. x?=w3286:bool)
              n1439 = Replace Array Subset(array=w3262, new element=w3259, index=w3261) -> (w3260:u16[])
              n1440 = Compound Arithmetic op=OR(w3286, w3282, w3285, w3284) -> (w3283:bool)
              n1441 = Select(t=myRIO_BRig_RT__Case_Exp_stateList."endExp" ("Enum"), s=w3283, f=myRIO_BRig_RT__Case_Exp_stateList."dummyState_endBlock" ("Enum")) -> (s? t:f=w3291:T2)
            }
            frame "endExp" {
            }
            frame "commConnect" {
              n1442 = call "myRIO_BRig_RT_comm_webdav_connect.vi"("input_password"="Host Password", "input_username"="Host UserName") -> ("output_Iconnected"=w3312:bool, "output_hSession"=w3330:T6)  [unwired: 7 in, 1 out]
              "Connected To Host?" <- w3312
              n1443 = case shown="False" w3312 {
                frame False {
                  n1444 = One Button Dialog(message="Connection Failed!\nData not being saved!") -> ()  [unwired: 1 in, 1 out]
                }
                frame True {
                }
              }
            }
            frame "commUpload_pre" {
              n1445 = Select(t=myRIO_BRig_RT__Case_Exp_stateList."commUpload_dataBlock" ("Enum"), s=w3337, f=myRIO_BRig_RT__Case_Exp_stateList."endBlock") -> (s? t:f=w3335:T2)
            }
            frame "commUpload_dataBlock" {
              n1446 = call "myRIO_BRig_RT_comm_webdav_uploadFile__data.vi"("input_fileName_prefix"=w3358, "input_fileName"="dataBlock" ("input_filename"), "input_hSession"=w3360) -> ()  [unwired: 8 in, 1 out]
            }
            frame "commUpload_dataCurrent" {
              n1447 = call "myRIO_BRig_RT_comm_webdav_uploadFile__data.vi"("input_fileName_prefix"=w3379, "input_fileName"="dataCurrent" ("input_filename"), "input_hSession"=w3381) -> ()  [unwired: 8 in, 1 out]
            }
            frame "commUpload_dataExp" {
              n1448 = call "myRIO_BRig_RT_comm_webdav_uploadFile__data.vi"("input_fileName_prefix"=w3400, "input_fileName"="dataExp" ("input_filename"), "input_hSession"=w3402) -> ()  [unwired: 8 in, 1 out]
            }
            frame "commUpload_dataLC" {
              n1449 = call "myRIO_BRig_RT_comm_webdav_uploadFile__data.vi"("input_fileName_prefix"=w3421, "input_fileName"="dataLC" ("input_filename"), "input_hSession"=w3423) -> ()  [unwired: 8 in, 1 out]
            }
            frame "commUpload_dataTrial" {
              n1450 = call "myRIO_BRig_RT_comm_webdav_uploadFile__data.vi"("input_fileName_prefix"=w3445, "input_fileName"="dataTrial" ("input_filename"), "input_hSession"=w3447) -> ()  [unwired: 8 in, 1 out]
            }
            frame "saveData_dataBlock" {
              # "idxDataBlockR"
              # "idxDataBlockL"
              n1451 = call "myRIO_BRig_RT_dataCurrent_idxDataBlockL.vi"() -> ("output_idxDataBlock__L"=w3471:i32)  [unwired: 11 in]
              n1452 = call "myRIO_BRig_RT_dataCurrent_idxDataBlockR.vi"() -> ("output_idxDataBlock__R"=w3472:i32)  [unwired: 11 in]
              n1453 = Index Array(array=w3473, index #1=w3471, index #2=w3472) -> (element #1=w3470:u16, element #2=w3469:u16)
              n1454 = Greater?(x=w3470, y=w3469) -> (0:w3468:bool)
              n1455 = Select(t=w3470, s=w3468, f=w3469) -> (s? t:f=w3466:u16)
              n1456 = Increment(x=w3466) -> (x+1=w3465:u16)
              n1457 = To Long Integer(number=w3465) -> (32bit integer=w3464:i32)
              n1458 = Array Subset(array=w3467, length (row)=w3464) -> (w3463:u16[][])  [unwired: 3 in]
              n1459 = call "myRIO_BRig_RT_comm_webdav_saveArrayToFile__2D_u16.vi"("Array"=w3463, "input_filename"="dataBlock") -> ()  [unwired: 10 in]
            }
            frame "saveData_dataCurrent" {
              n1460 = call "myRIO_BRig_RT_comm_webdav_saveArrayToFile__1D_u16.vi"("Array"=w3492, "input_filename"="dataCurrent") -> ()  [unwired: 10 in]
            }
            frame "saveData_dataExp" {
              # "runTime"
              n1461 = Get Date/Time In Seconds() -> (seconds since 1Jan1904=w3520:timestamp)
              n1462 = To Double Precision Float(number=w3520) -> (double precision float=w3519:dbl)
              n1463 = call "myRIO_BRig_RT_dataExp_runTime_seconds.vi"() -> ("output_RunTime_minutes"=w3518:i32)  [unwired: 11 in]
              n1464 = Subtract(x=w3519, y=w3517) -> (x-y=w3514:dbl)
              n1465 = To Unsigned Word Integer(number=w3514) -> (unsigned 16bit integer=w3513:u16)
              n1466 = Replace Array Subset(array=w3512, new element=w3513, index=w3518) -> (w3515:u16[])
              n1467 = call "myRIO_BRig_RT_comm_webdav_saveArrayToFile__1D_u16.vi"("Array"=w3515, "input_filename"="dataExp") -> ()  [unwired: 10 in]
            }
            frame "saveData_dataLC" {
              n1468 = call "myRIO_BRig_RT_comm_webdav_saveArrayToFile__1D_u16.vi"("Array"=w3539, "input_filename"="dataLC") -> ()  [unwired: 10 in]
            }
            frame "saveData_dataTrial" {
              # "idxTrial"
              n1469 = call "myRIO_BRig_RT_dataCurrent_idxDataTrial.vi"() -> ("output_idxDataTrial"=w3563:i32)  [unwired: 11 in]
              n1470 = Index Array(array=w3564, index=w3563) -> (element=w3556:u16)
              n1471 = Increment(x=w3556) -> ()  [unwired: 1 out]
              n1472 = To Long Integer(number=w3556) -> (32bit integer=w3560:i32)
              n1473 = Array Subset(array=w3561, length (row)=w3560) -> (w3562:u16[][])  [unwired: 3 in]
              n1474 = call "myRIO_BRig_RT_comm_webdav_saveArrayToFile__2D_u16.vi"("Array"=w3562, "input_filename"="dataTrial") -> ()  [unwired: 10 in]
            }
            frame "dummyState" {
              n1475 = call "myRIO_BRig_RT_dataCurrent_iTrial.vi"() -> ("output_iTrial"=w3586:i32)  [unwired: 11 in]
              n1476 = Index Array(array=w3587, index=w3586) -> (element=w3585:u16)
              n1477 = Equal?(x=w3585, y=u16 1) -> (x = y?=w3583:bool)
              n1478 = Equal To 0?(x=w3594) -> (x = 0?=w3595:bool)
              n1479 = Select(t=u16 13, s=w3583, f=u16 15) -> (s? t:f=w3580:u16)
              n1480 = Select(t=w3580, s=w3595, f=w3594) -> (s? t:f=w3593:u16)
              n1481 = Decrement(x=w3593) -> (x-1=w3592:u16)
              n1482 = Equal To 0?(x=w3592) -> (x = 0?=w3591:bool)
              n1483 = Select(t=myRIO_BRig_RT__Case_Exp_stateList."initTrial" ("Enum"), s=w3591, f=w3589) -> (s? t:f=w3588:T2)
            }
            frame "dummyState_endBlock" {
              n1484 = call "myRIO_BRig_RT_dataCurrent_iTrial.vi"() -> ("output_iTrial"=w3619:i32)  [unwired: 11 in]
              n1485 = Index Array(array=w3620, index=w3619) -> (element=w3618:u16)
              n1486 = Equal?(x=w3618, y=u16 1) -> (x = y?=w3616:bool)
              n1487 = Equal To 0?(x=w3627) -> (x = 0?=w3628:bool)
              n1488 = Select(t=u16 1, s=w3616, f=u16 3) -> (s? t:f=w3613:u16)
              n1489 = Select(t=w3613, s=w3628, f=w3627) -> (s? t:f=w3626:u16)
              n1490 = Decrement(x=w3626) -> (x-1=w3625:u16)
              n1491 = Equal To 0?(x=w3625) -> (x = 0?=w3624:bool)
              n1492 = Select(t=myRIO_BRig_RT__Case_Exp_stateList."initBlock" ("Enum"), s=w3624, f=w3622) -> (s? t:f=w3621:T2)
            }
          }
          n1493 = local read "MTrig_Laser_Switch"() -> (w1354:bool)
          n1494 = Not(x=w1354) -> (.not. x?=w1355:bool)
          n1495 = Select(t=w1392, s=w1395, f=w1393) -> (s? t:f=w1394:bool)
          n1496 = And(x=w1356, y=w1355) -> (x .and. y?=w1350:bool)
          n1497 = And(x=w1356, y=w1354) -> (x .and. y?=w1352:bool)
          n1498 = Or(x=w1353, y=w1352) -> (x .or. y?=w1343:bool)
          n1499 = Or(x=w1352, y=w1351) -> (x .or. y?=w1342:bool)
          n1500 = Or(x=w1349, y=w1350) -> (x .or. y?=w1345:bool)
          n1501 = Or(x=w1350, y=w1348) -> (x .or. y?=w1344:bool)
          n1502 = Or(x=w1358, y=w1359) -> (x .or. y?=w1347:bool)
          n1503 = Or(x=w1421, y=w1420) -> (x .or. y?=w1346:bool)
          n1504 = case shown="True" w1449 {
            tunnel: w1446 -> [w1470 w1478]
            tunnel: w1448 -> [_ w1474]
            tunnel: w1447 -> [_ w1473]
            tunnel: w1370 -> [_ w1472]
            tunnel: w1418 -> [_ w1471]
            tunnel: [w1470 w1477] -> w1445
            tunnel: w1444 -> [w1469 w1476]
            tunnel: [w1469 w1475] -> w1443
            frame False {
            }
            frame True {
              n1505 = call "myRIO_BRig_RT__Case_Exp__recordLick.vi"("intput_state__trialEnd"=w1471, "intput_state__trialStart"=w1472, "input_lick__R"=w1473, "input_lick__L"=w1474, "input_dataCurrent"=w1476, "input_dataLick"=w1478) -> ("output_dataCurrent"=w1475:u16[], "output_dataLick"=w1477:u16[][])  [unwired: 4 in]
            }
          }
          n1506 = Or(x=w1422, y=w1407) -> (x .or. y?=w1396:bool)
          n1507 = Or(x=w1406, y=w1423) -> (x .or. y?=w1419:bool)
          n1508 = Or(x=w1450, y="STOP_abort") -> (x .or. y?=w1452:bool)
          n1509 = Select(t=w1381, s=w1382, f=w1380) -> (s? t:f=w1369:u16)
          n1510 = Select(t=w1383, s=w1385, f=w1384) -> (s? t:f=w1368:u16)
          n1511 = Select(t=u16 0, s=w1388, f=w1387) -> (s? t:f=w1372:u16)
          n1512 = xnode "Read/Write Control"("FPGA VI Reference In"=w1398, "error in"=w1397, "A6_Act"=w1394, "audioTrigger_L"=w1396, "audioAmp_L"=w1432, "audioFreq_L_kHz"=w1405, "audioTrigger_R"=w1419, "audioAmp_R"=w1433, "audioFreq_R_kHz"=w1434, "CueLed_Event"=w1357, "A3_SL"=w1347, "A1_SR"=w1346, "LC_Event_l1"=w1345, "LC_Laser_l1"=w1344, "LC_Event_l2"=w1343, "LC_Laser_l2"=w1342) -> ("FPGA VI Reference Out"=w1442:refnum<k20>, "error out"=w1441:errorcluster, "AnaIn_0"=w1362:i16, "AnaIn_1"=w1371:i16)
          n1513 = call "myRIO_BRig_RT_dataAnalog_enterData__PortC.vi"("input_iState"=w1370, "input_AI0"=w1362, "input_iEvent"=w1372, "input_AI1"=w1371, "input_iTrial"=w1369, "input_iBlock"=w1368, "input_index"=w1373, "input_dataAnalog"=w1391) -> ("output_dataAnalog"=w1390:u16[][])  [unwired: 3 in]
          n1514 = call "myRIO_BRig_RT_TCP__v3__PortC.vi"("input_hTCP"=w1378, "input_AI1"=w1371, "input_AI0"=w1362, "input_I_connected_TCP"=w1374, "input_iBlock"=w1368, "input_spout"=w1367, "input_iTrial"=w1369, "input_error"=w1376, "input_countTrial"=w1364, "input_iState"=w1370) -> ("output_hTCP"=w1377:refnum<k5>, "output_countTrial"=w1363:u16, "output_error"=w1375:errorcluster)  [unwired: 3 in]
          n1515 = node-c288() -> ()  [unwired: 1 in, 1 out]
          n1516 = Increment(x=w1372) -> (x+1=w1379:u16)
          n1517 = Increment(x=w1373) -> (x+1=w1389:i32)
          "cState" <- w1370
        }
        n1518 = node-c288(w1292) -> ()  [unwired: 1 out]
        n1519 = flat-sequence {
          tunnel: w1288 -> [w1337]
          tunnel: w1287 -> [w1336]
          tunnel: [w1335] -> w1280
          tunnel: [w1334] -> w1279
          tunnel: [w1340] -> w1281
          tunnel: [w1341] -> w1286
          tunnel: w1280 -> [w1341]
          tunnel: w1279 -> [w1340]
          frame #0 {
            w1331 = u8 0
            w1332 = u16 0 ("AudioLeft_phase_inc")
            w1333 = FALSE
            n1520 = xnode "Read/Write Control"("FPGA VI Reference In"=w1337, "error in"=w1336, "Counts_Reset"=TRUE, "audioTrigger_L"=w1333, "audioFreq_L_kHz"=w1331, "audioAmp_L"=w1332, "audioTrigger_R"=w1333, "audioFreq_R_kHz"=w1331, "audioAmp_R"=w1332, "A3_SL"=w1333, "A1_SR"=w1333, "A6_Act"=w1333) -> ("FPGA VI Reference Out"=w1335:refnum<k20>, "error out"=w1334:errorcluster)
          }
          frame #1 {
            w1339 = FALSE ("START")
            n1521 = local write "START"(w1339) -> ()
            n1522 = local write "STOP_endTrial"(w1339) -> ()
            n1523 = local write "STOP_endBlock"(w1339) -> ()
          }
        }
        n1524 = stacked-sequence {
          tunnel: w1264 -> [w1311 _]
          tunnel: w1262 -> [w1312 _]
          tunnel: w1261 -> [_ w1317]
          tunnel: w1260 -> [_ w1316]
          tunnel: w1259 -> [_ w1315]
          tunnel: w1258 -> [w1305 _]
          tunnel: w1238 -> [w1302 _]
          tunnel: w1237 -> [w1301 _]
          frame #0 {
            n1525 = call "myRIO_BRig_RT_dataCurrent_idxDataLick.vi"() -> ("output_idxDataLick"=w1306:i32)  [unwired: 11 in]
            n1526 = Index Array(array=w1305, index=w1306) -> (element=w1308:u16)
            n1527 = Array Subset(array=w1302, length (row)=w1301) -> (w1303:u16[][])  [unwired: 3 in]
            n1528 = Increment(x=w1308) -> (x+1=w1309:u16)
            n1529 = call "myRIO_BRig_RT_comm_webdav_saveArrayToFile__1D_u16.vi"("Array"=w1312, "input_filename"="dataMTrig") -> ()  [unwired: 10 in]
            n1530 = To Long Integer(number=w1309) -> (32bit integer=w1307:i32)
            n1531 = Array Subset(array=w1311, length (row)=w1307) -> (w1310:u16[][])  [unwired: 3 in]
            n1532 = call "myRIO_BRig_RT_comm_webdav_saveArrayToFile__2D_u16.vi"("Array"=w1310, "input_filename"="dataLick") -> ()  [unwired: 10 in]
            n1533 = call "myRIO_BRig_RT_comm_webdav_saveArrayToFile__2D_u16.vi"("Array"=w1303, "input_filename"="dataAnalog") -> ()  [unwired: 10 in]
          }
          frame #1 {
            n1534 = case shown="True" w1317 {
              tunnel: w1316 -> [_ w1319]
              tunnel: w1315 -> [_ w1318]
              frame False {
              }
              frame True {
                n1535 = stacked-sequence {
                  tunnel: w1319 -> [w1321 w1328 w1330]
                  tunnel: w1318 -> [w1322 w1327 _]
                  frame #0 {
                    n1536 = call "myRIO_BRig_RT_comm_webdav_uploadFile__announce.vi"("input_addText"=TRUE, "input_fileName_prefix"=w1322, "intput_fileName"="curExp_end", "intput_hSession"=w1321) -> ("output_Isuccess"=w1320:bool)  [unwired: 6 in, 1 out]
                    n1537 = case shown="True" w1320 {
                      frame False {
                        n1538 = One Button Dialog(message="!!! Warning !!! Your data is located at C:\\BehaviorRig\\commTransfer") -> ()  [unwired: 1 in, 1 out]
                      }
                      frame True {
                        n1539 = Wait (ms)(milliseconds to wait=u32 20) -> ()  [unwired: 1 out]
                      }
                    }
                  }
                  frame #1 {
                    n1540 = call "myRIO_BRig_RT__endExp_sendData.vi"("input_fileName_prefix"=w1327, "input_hSession"=w1328) -> ()  [unwired: 8 in, 2 out]
                  }
                  frame #2 {
                    n1541 = local write "Connected To Host?"(FALSE ("Connected To Host?")) -> ()
                    n1542 = call <vilib>:"Close Session.vi"("session handle"=w1330) -> ()  [unwired: 14 in, 1 out]
                  }
                }
              }
            }
          }
        }
      }
    }
    n1543 = local read "STOP_abort"() -> (w44:bool)
  }
  n1544 = case shown="True" w5 {
    tunnel: w4 -> [_ w3651]
    tunnel: w3 -> [_ w3650]
    frame False {
    }
    frame True {
      n1545 = call "myRIO__TCP_disconnect_forWrite.vi"("input_error"=w3650, "input_hTCP"=w3651) -> ()  [unwired: 9 in, 1 out]
    }
  }
  n1546 = xnode "Read/Write Control"("FPGA VI Reference In"=w16, "error in"=w15, "FPGA_Stop"=TRUE) -> ("FPGA VI Reference Out"=w21:refnum<k20>, "error out"=w22:errorcluster)
  n1547 = xnode "Close FPGA VI Reference"("FPGA VI Reference In"=w21, "error in"=w22) -> ("error out"=w20:errorcluster)
  n1548 = call <vilib>:"Reset myRIO.vi"("error in (no error)"=w20) -> ()  [unwired: 10 in, 1 out]
